vi "SOUR_POW_CORR_DATA.vi"(0 "VISA IN":refnum<visa-resource-name>, 5 "error in":errorcluster, 7 "Channel":i32) -> (14 "VISA Out":refnum<visa-resource-name>, 19 "error out":errorcluster)   [LabVIEW 2018, in "PNA-X.lvlib"]
doc: "SOURce:POWer:CORRection:DATA \nParameters \n<char> Choose from: \nREAL,32 - (default value for REAL) Best for transferring large amounts of \nmeasurement data. \nREAL,64 - Slower but has more significant digits than REAL,32. Use \nREAL,64 if you have a computer that doesn't support REAL,32. \nASCii,0 - The easiest to implement, but very slow. Use if small amounts of \ndata to transfer. \nNote: The REAL,32 and REAL,64 arguments transfer data in block format as \nexplained in Transferring Measurement Data. \nExamples FORM REAL,64 \nformat:data ascii \nQuery Syntax FORMat:DATA? \nReturn Type Character,Character \nDefault ASCii,0 \n1603\n\nHardcopy Command \nLearn about Printing \nSCPI Command Tree \nHCOPy:FILE <filename> \n(Write-only) Saves the screen image to a file. \nParameters \n<filename> Name of the file to save the screen to. The file is saved to the current working \ndirectory unless a valid full path name is specified. \nUse one of the following suffixes: \n.bmp - not recommended due to large file size \n.jpg - not recommended due to poor quality \n.png - recommended \nExamples HCOPY:FILE \"myFile.png\" \nhcopy:file \"c:\\data\\myfile.png\" \nQuery Syntax Not Applicable \nDefault Not Applicable \nHCOPy[:IMMediate] \n(Write-only) Prints the screen to the default printer. \nExamples HCOP \nhcopy:immediate \nQuery Syntax Not applicable \nDefault Not Applicable \n1604\n\nInitiate Commands \nControls triggering signals \nClick on a blue keyword to view the command details. \nSee Also \nExample Triggering the PNA \nLearn about Triggering \nSynchronizing the PNA and Controller \nSCPI Command Tree \nINITiate:CONTinuous <boolean> \n(Read-Write) Specifies whether the PNA trigger source is set to Internal (continuous) or Manual. \nThis command is a subset of TRIG:SEQ:SOURce, which can also set the trigger source to External. \nTo set how a channel responds to trigger signals, use SENS:SWE:MODE. \nSee a map of user interface to SCPI triggering commands. \nFor more information on triggering, see the PNA Trigger Model. \nSee the Example program: Triggering the PNA using SCPI. \nParameters \n<boolean> ON (or 1) - Internal (continuous) trigger. \nOFF (or 0) - Manual sweep. Use INIT:IMMediate to send a trigger signal \nExamples INIT:CONT ON \ninitiate:continuous off \nQuery Syntax INITiate:CONTinuous? \nReturn Type Boolean (1 = ON, 0 = OFF) \nDefault ON \n1605\n\nINITiate<cnum>[:IMMediate] \n(Write-only) Stops the current sweeps and immediately sends a trigger. (Same as Trigger! on the PNA \nfront panel). \nSee the Example program: Triggering the PNA using SCPI \nNote: An SMC Fixed Output measurement cannot be triggered using this command. For more \ninformation, see the example program. \nThis command requires Trigger:Source to be set to Manual. This causes ONE trigger signal to be \nSENT each time INIT:IMM is issued. \nSens<ch>:Sweep:Mode sets the number of trigger signals each channel will ACCEPT (Continuous - \nunlimited, Groups - a specific number, or HOLD - none.) \nTo trigger ALL channels in turn: \nSet ALL channels to Sens<ch>:Sweep:Mode Continuous. The <ch> argument in INIT<ch>:IMM is \nignored. \nThen�\nTRIG:SCOP ALL triggers ALL channels (in sequence) each time Init:Imm is sent. \nTRIG:SCOP CURRent triggers ONLY the NEXT channel each time Init:Imm is sent. \nTo trigger ONLY a specified channel: \nSet ALL channels to Sens<ch>:Sweep:Mode HOLD 1. \nSend TRIG:SCOP CURRent 2. \nSend Init<ch>:Imm where <ch> is the channel to be triggered. 3. \nAdvanced Situations that require some channels to be in CONT and others in HOLD are rare. The \nfollowing describes the behavior of the Init:Imm command in these situations: \nWhen Trigger:Scope = Global: \nIf the SPECIFIED <cnum> channel is in hold mode, it is put in single trigger (accepts 1 trigger signal) and \ngoes to the end of the queue of channels to be triggered. The other 'non-hold' channels are triggered. The \nnext Init:Imm triggers the specified channel first. \nFor example: ch1 is in Hold, ch2 and ch3 are in CONT and we send INIT1:IMM \n1606\n\nOn the first INIT:IMM, ch2 and ch3 is triggered. \nnext INIT:IMM, ch1, ch2, ch3 is triggered. \nnext INIT:IMM, ch2 and ch3 is triggered. \nnext INIT:IMM, ch1, ch2, ch3 is triggered, and so forth. \nWhen Trigger:Scope = Channel \nOnly ONE channel is triggered for each issued INIT<ch>:IMM command. \nIf the specified channel is in hold, it is put in single trigger (accepts 1 trigger signal) and goes the end of the \nqueue of channels to be triggered as in the 'Global' example. \nThis is one of the PNA overlapped commands. Learn more. \nParameters \n<cnum> Any existing channel number. If unspecified, value is set to 1 \nExamples INIT \ninitiate2:immediate \nQuery Syntax Not applicable \nDefault Not applicable \nLast modified: \nApril 23, 2007 Updated Init:Imm \n1607\n\nMemory Commands \nThe memory commands control saving and loading instrument states and measurement trace data to the \nhard drive. To read and write trace data in GPIB format, see CALC:DATA. \nClick on a blue keyword to view the command details. \nSee Also \nExample Programs \nLearn about Save / Recall and File Types \nSynchronizing the PNA and Controller \nSCPI Command Tree \nSpecifying Path Names \nThe MMEM commands use the following rules to specify path names: \nThe default folder is \"C:\\Program Files\\Agilent\\Network Analyzer\\Documents\" \nYou can change the active directory using MMEMory:CDIRectory. \nSpecify only the file name if using the active directory. \nYou can also use an absolute path name to specify the folder and file. \nMMEMory:CATalog[:<char>]? [<folder>] \n1608\n\n(Read-only) Returns a comma-separated string of file names that are in the specified folder. If there \nare no files of the specified type, \"NO CATALOG\" is returned. Learn about File Types \nParameters \n<char> The type of files to list. Choose from: \nSTATe - Instrument states (.sta) \nCORRection - Calibration Data (.cal) \nCSARchive - Instrument state and calibration data (.csa) \nCSTate - Instrument state and link to Calibration data (.cst) \nIf unspecified then ALL file types (even unknown types) are listed. \n<folder> String - Any existing folder name. See Specifying Path Names \nExamples MMEM:CAT? 'lists all files from the current folder \nmmemory:catalog:correction? 'C:\\Program Files\\Agilent\\Network \nAnalyzer\\Documents' 'lists .cal files from the specified folder \nDefault Not applicable \nMMEMory:CDIRectory <folder> \n(Read-Write) Changes the folder name. \nParameters \n<folder> Any drive and folder name that already exists. \nIf the same level as \"C:\\Program Files\\Agilent\\Network Analyzer\\Documents\", \nthen no punctuation is required \nMMEM:CDIR Service \nIf the new folder is at a different level than \"C:\\Program Files\\Agilent\\Network \nAnalyzer\\Documents\", use a slash (\\) before the folder name and enclose in \nquotes. \nmmemory:cdirectory '\\automation' 'changes default directory up \none level. \nYou can use an absolute path to specify the new folder. \nmmemory:cdirectory 'c:\\automation\\service' \nQuery Syntax MMEMory:CDIRectory? 'Returns the current folder name \n1609\n\nReturn Type String \nDefault 'C:\\Program Files\\Agilent\\Network Analyzer\\Documents' \nMMEMory:COPY <file1>,<file2> \n(Write-only) Copies file1 to file2. Extensions must be specified. \nParameters \n<file1> String - Name of the file to be copied. See Specifying Path Names \n<file2> String - Name of the file to be created from file1. \nExamples MMEM:COPY 'MyFile.cst','YourFile.cst' \nQuery Syntax Not applicable \nDefault Not applicable \nMMEMory:DELete <file> \n(Write-only) Deletes file. Extensions must be specified. \nParameters \n<file> String - Name of the file to be deleted. See Specifying Path Names \nExamples MMEM:DEL 'MyFile.cst' \nQuery Syntax Not applicable \nDefault Not applicable \nMMEMory:LOAD[:<char>] <file> \n1610\n\n(Write-only) Loads the specified file. Learn about File Types \nParameters \n<char> The type of file to load. Choose from: \nSTATe - Instrument states (.sta) \nCORRection - Calibration Data (.cal) \nCSARchive - Instrument state and calibration data (.csa) \nCSTate - Instrument state and link to Calibration data (.cst) \nIf <char> is unspecified, the extension must be included in the filename. \nIf an extension is specified in <file> that does not agree with <char> then no \naction is taken. \n<file> String - Name of the file to be loaded. See Specifying Path Names \nExamples MMEM:LOAD 'MyFile.cst' \nmmemory:load:state 'MyInstState' \nQuery Syntax Not applicable \nDefault Not applicable \nMMEMory:MDIRectory <folder> \n(Write-only) Makes a folder. \nParameters \n<folder> String - Name of the folder to make. See Specifying Path Names \nExamples MMEM:MDIR 'MyFolder' \nmmemory:mdirectory 'c:\\NewFolder' \nQuery Syntax Not applicable \nDefault Not applicable \nMMEMory:MOVE <file1>,<file2> \n1611\n\n(Write-only) Renames <file1> to <file2>. File extensions must be specified. \nParameters \n<file1> String - Name of the file to be renamed. See Specifying Path Names \n<file2> String - Name of the new file. \nExamples MMEM:MOVE 'MyFile.cst','YourFile.cst' \nQuery Syntax Not applicable \nDefault Not applicable \nMMEMory:RDIRectory <folder> \n(Write-only) Removes the specified folder. \nParameters \n<folder> String - Name of the folder to remove. See Specifying Path Names \nExamples MMEM:RDIR 'MyFolder' \nQuery Syntax Not applicable \nDefault Not applicable \nMMEMory:STORe[:<char>] <file> \n(Write-only) Stores the specified file (.sta, .cal, .csa, .cst, prn). \nTo save snp files, use Calc:Data:SNP:PORTs:SAVE. \nTo save *.cti files, use MMEM:STOR:CIT:DATA or MMEM:STOR:CIT:FORM. \nParameters \n<char> The type of file to store. Choose from: \nSTATe - Instrument states (.sta) \nCORRection - Calibration Data (.cal) \nCSARchive - Instrument state and calibration data (.csa) \nCSTate - Instrument state and link to Calibration data (.cst) \nNo <char> is specified for prn. \n1612\n\nIf <char> is unspecified, then the extension must be included in the filename. \nIf an extension is specified in <file> that does not agree with <char> then no \naction is taken. \nLearn about File Types \n<file> String - Name of any valid file that is not already in existence. See Specifying \nPath Names \nExamples MMEM:STOR:STAT 'myState' \nmmemory:store 'c:\\bin\\myState.sta' \nMMEM:STOR 'MyData.prn' \nQuery Syntax Not applicable \nDefault Not applicable \nMMEMory:STORe:CITifile:DATA <filename> \n(Write only) Saves UNFORMATTED trace data to .cti file. Learn more. \nParameters \n<filename> Any drive and folder name that already exists. \nIf the same level as \"C:\\Program Files\\Agilent\\Network Analyzer\\Documents\", \nthen no punctuation is required \nMMEM:STOR:CIT:DATA MYCTIFile \nIf the new folder is at a different level than \"C:\\Program Files\\Agilent\\Network \nAnalyzer\\Documents\", use a slash (\\) before the folder name and enclose in \nquotes. \nmmemory:cdirectory '\\automation' 'changes default directory up \none level. \nYou can use an absolute path to specify the new folder. \nmmemory:cdirectory 'c:\\automation\\service' \nQuery Syntax Not Applicable \nDefault C:\\Program Files\\Agilent\\Network Analyzer\\Documents' \nMMEMory:STORe:CITifile:FORMat <filename> \n1613\n\n(Write only) Saves FORMATTED trace data to .cti file. Learn more. \nParameters \n<filename> Any drive and folder name that already exists. \nIf the same level as \"C:\\Program Files\\Agilent\\Network Analyzer\\Documents\", \nthen no punctuation is required \nMMEM:STOR:CIT:DATA MYFile \nIf the new folder is at a different level than \"C:\\Program Files\\Agilent\\Network \nAnalyzer\\Documents\", use a slash (\\) before the folder name and enclose in \nquotes. \nmmemory:cdirectory '\\automation' 'changes default directory up \none level. \nYou can use an absolute path to specify the new folder. \nmmemory:cdirectory 'c:\\automation\\service' \nQuery Syntax Not Applicable \nDefault C:\\Program Files\\Agilent\\Network Analyzer\\Documents' \nMMEMory:STORe:TRACe:CONTents:CITifile <char> \n(Read-Write) Specifies the contents of subsequent citifile save statements. (See Data Define Saves) \nParameters \n<char> Choose from: \nSING - Single trace \nDISP - All displayed traces \nAUTO - All displayed traces \nExamples MMEM:STOR:TRAC:CONT:CIT SING \nQuery Syntax MMEMory:STORe:TRACe:CONTents? \nReturn Type Character \nDefault Auto \nMMEMory:STORe:TRACe:FORMat:CITifile <char> \n1614\n\n(Read-Write) Specifies the format of subsequent citifile save statements. (See Data Define Saves) \nParameters \n<char> Format in which the citifile will be saved with subsequent \nMMEMory:STORe:CIT:FORMat statements. Choose from: \nMA - Linear Magnitude / degrees \nDB - Log Magnitude / degrees \nRI - Real / Imaginary \nAUTO - Format in which the trace is already displayed. If other than Log \nMag, Linear Magnitude, or Real/Imag, then the format will be in Real/Imag. \nExamples MMEM:STOR:TRAC:FORM:CIT MA \nQuery Syntax MMEMory:STORe:TRACe:FORMat:CITifile? \nReturn Type Character \nDefault Auto' \nMMEMory:STORe:TRACe:FORMat:SNP <char> \n(Read-Write) Specifies the format of subsequent .s1p, .s2p, .s3p; s4p save statements. (See Data \nDefine Saves). \nParameters \n<char> Choose from: \nMA - Linear Magnitude / degrees \nDB - Log Magnitude / degrees \nRI - Real / Imaginary \nAUTO - data is output in currently selected trace format. If other than LogMag, \nLinMag, or Real/Imag, then output is in Real/Imag. \nExamples MMEM:STOR:TRAC:FORM:SNP MA \nQuery Syntax MMEMory:STORe:TRACe:FORMat:SNP? \nReturn Type Character \nDefault Auto' \n1615\n\nMMEMory:TRANsfer <fileName>,<dataBlock> \n(Read-Write) Transfers data between the PNA and an external controller. Other MMEM commands \ntransfer data between the PNA application and the PNA hard drive. If <fileName> already exists, it \nwill be overwritten. The file must be no larger than 20MB. \nTo read trace data from the PNA in block format, use CALC:DATA. \nParameters \n<fileName> String - File name. See Specifying Path Names \n<dataBlock> Block Data - The contents of the file. \nThe data block is a block of binary data. Use the following syntax: \n#<num digits><byte count><data bytes><NL><END> \nwhere: \n<num_digits> specifies how many digits are contained in <byte_count> \n<byte_count> specifies how many data bytes will follow in <data bytes> \nExample See example program \nQuery Syntax MMEMory:TRANsfer? <fileName> \nReads block data from the specified file location. \nDefault Not applicable \nLast modified: \n9/12/06 MQ Store command has reference to PORTS Snp. \n1616\n\nOutput Command \nLearn about Power \nOUTPut[:STATe] <ON | OFF> \n(Read-Write) Turns RF power from the source ON or OFF. \nSee note about source power state with instrument state save and recall. \nParameters \n<ON | OFF> ON (or 1) - turns RF power ON \nOFF (or 0) - turns RF power OFF \nExamples OUTP ON \noutput:state off \nQuery Syntax OUTPut[:STATe]? \nReturn Type Boolean (1 = ON, 0 = OFF) \nDefault ON \n1617\n\nRoute Command \nLearn about Frequency Offset \nSCPI Command Tree \nROUTe<cnum>:PATH:LOOP[:R1] <char> \n(Read-Write) Throws internal switch to reference receiver when the specified channel is measured. \nThis feature is only available on PNA models with Option 081 - external reference switch. See block \ndiagram of the reference switch. \nParameters \n<cnum> Any existing channel number. If unspecified, value is set to 1 \n<char> Position of the switch. Choose from: \nINTernal - bypass R1 Loop. Connects the port 1 source directly to the R1 \nreceiver. \nEXTernal - flow through R1 Loop. Allows direct access to the R1 receiver \nthrough the Reference 1 front-panel connectors. \nExamples ROUT:PATH:LOOP INT \nroute2:path:loop:r1 external \nQuery Syntax ROUTe<cnum>:PATH:LOOP:R1? \nReturn Type Character \nDefault INTernal \n1618\n\nSense:Average Commands \nSets sweep-to-sweep averaging parameters. Averaging is a noise reduction technique that averages \neach data point over a user-specified number of sweeps. Averaging affects all of the measurements in \nthe channel. \nClick on a blue keyword to view the command details. \nSee Also \nExample using some of these commands. \nLearn about Averaging \nSynchronizing the PNA and Controller \nSCPI Command Tree \nSENSe<cnum>:AVERage:CLEar \n(Write-only) Clears and restarts averaging of the measurement data. Must also set \nSENS:AVER[:STATe] ON \nParameters \n<cnum> Any existing channel number; if unspecified, value is set to 1. \nExamples SENS:AVER:CLE \nsense2:average:clear \nQuery Syntax Not applicable \nDefault Not applicable \nSENSe<cnum>:AVERage:COUNt <num> \n1619\n\n(Read-Write) Sets the number of measurement sweeps to combine for an average. Must also set \nSENS:AVER[:STATe] ON \nParameters \n<cnum> Any existing channel number; if unspecified, value is set to 1. \n<num> Number of measurement sweeps to average. Choose any number between 1 \nand 65536 (2^16). \nExamples SENS:AVER:COUN 999 \nsense2:average:count 73 \nQuery Syntax SENSe<cnum>:AVERage:COUNt? \nReturn Type Numeric \nDefault 1 \nSENSe<cnum>:AVERage[:STATe] <ON | OFF> \n(Read-Write) Turns trace averaging ON or OFF. \nParameters \n<cnum> Any existing channel number; if unspecified, value is set to 1. \n<ON | OFF> ON (or 1) - turns averaging ON. \nOFF (or 0) - turns averaging OFF. \nExamples SENS:AVER ON \nsense2:average:state off \nQuery Syntax SENSe<cnum>:AVERage[:STATe]? \nReturn Type Boolean (1 = ON, 0 = OFF) \nDefault Off \n1620\n\nSense:Bandwidth Commands \nSee Also \nExample Programs \nLearn about IF Bandwidth \nSynchronizing the PNA and Controller \nSCPI Command Tree \nSENSe<cnum>:BANDwidth | BWIDth[:RESolution] <num> \n(Read-Write) Sets the bandwidth of the digital IF filter to be used in the measurement. (Use either \nSense:Bandwidth or Sense:Bwidth) \nParameters \n<cnum> Any existing channel number. If unspecified, value is set to 1 \n<num> IF Bandwidth in Hz. The list of valid IF Bandwidths is different depending on \nthe PNA model. (Click to see the lists.) If an invalid number is specified, the \nanalyzer will round up to the closest valid number. \nExamples SENS:BWID 1KHZ \nsense2:bandwidth:resolution 1000 \nQuery Syntax SENSe<cnum>:BANDwidth | BWIDth[:RESolution]? \nReturn Type Numeric \nDefault See Preset IFBW for your PNA model. \nSENSe<cnum>:BANDwidth | BWIDth:TRACk <bool> \n1621\n\n(Read-Write) Sets and returns the state of the Reduce IF BW at Low Frequencies feature. \n(Use either Sense:Bandwidth:Track or Sense:Bwidth:Track). \nParameters \n<cnum> Any existing channel number. If unspecified, value is set to 1 \n<bool> Choose from: \nON or 1 - Reduce IF BW at Low Frequencies is set ON \nOFF or 0 - Reduce IF BW at Low Frequencies is set OFF \nExamples SENS:BWID:TRAC OFF \nsense2:bandwidth:track 1 \nQuery Syntax SENSe<cnum>:BANDwidth | BWIDth:TRACk? \nReturn Type Boolean \nDefault ON \n1622\n\nSense:Correction Commands \nPerforms and applies calibration and other error correction features. \nTo perform Guided Calibration, see Sens:Corr Coll:GUIDed. \n1623\n\nClick on a blue keyword to view the command details. \nSee Also \nExample Programs \nNew See Calibrating the PNA Using SCPI \nLearn about Measurement Calibration \nSynchronizing the PNA and Controller \nSCPI Command Tree \nSENSe<cnum>:CORRection:CCHeck[:ACQuire] <mod>[,char] \n(Write-only) Reads the 'confidence data' associated with the specified ECal module and puts it into \nmemory. The measurement is selected using SENS:CORR:CCH:PAR. This command is compatible \nwith *OPC. \nParameters \n<cnum> Any existing channel number. If unspecified, value is set to 1. \n<mod> ECAL Module that contains the confidence data. Choose from: \nECAL1 \n..through.. \nECAL8 \n[char] Optional argument. Specifies which characterization within the ECal module \nthat the confidence data will be read from. \nCHAR0 Factory characterization (data that was stored in the ECal module by \n1624\n\nAgilent). Default if not specified. \nCHAR1 User characterization #1 \nCHAR2 User characterization #2 \nCHAR3 User characterization #3 \nCHAR4 User characterization #4 \nCHAR5 User characterization #5 \nExamples SENS:CORR:CCHeck ECAL2 \nsense2:correction:ccheck:acquire ecal1,char1 \nQuery Syntax Not applicable \nDefault Not applicable \nSENSe<cnum>:CORRection:CCHeck:DONE \n(Write-only) Concludes the Confidence Check and sets the ECal module back into the idle state. \nParameters \n<cnum> Any existing channel number. If unspecified, value is set to 1 \nExamples SENS:CORR:CCH:DONE \nsense2:correction:ccheck:done \nQuery Syntax Not applicable \nDefault Not applicable \nSENSe<cnum>:CORRection:CCHeck:PARameter <Mname> \n1625\n\n(Read-Write) Specifies an existing measurement to be used for the Confidence Check. \nParameters \n<cnum> Any existing channel number. If unspecified, value is set to 1 \n<Mname> Name of the measurement you are selecting for the confidence check. The \nmeasurement must already exist. \nExamples SENS:CORR:CCH:PAR 'TEST' \n'selects the measurement \"test\" on channel 1 for the confidence \ncheck \nsense2:correction:ccheck:parameter 'test' \n'selects the measurement \"test\" on channel 2 for the confidence \ncheck \nQuery Syntax SENSe<cnum>:CORRection:CCHeck:PARameter? \nReturns the name of the selected measurement on channel <cnum>. \nReturn Type String \nDefault Not applicable \nSENSe<cnum>:CORRection:COLLect[:ACQuire] <class>[,subclass] \n(Write-only) For UNGUIDED calibration, measures the specified standards from the selected \ncalibration kit. The calibration kit is selected using the Sense:Correction:Collect:CKIT command. \nFor using two sets of standards, see SENS:CORR:TST. \nNote: Before using this command you must select two items: \n1. Select a calibration method using SENS:CORR:COLL:METH \n2. Select a measurement using CALC:PAR:SEL. You can select one measurement for each channel. \nParameters \n<cnum> Any existing channel number. If unspecified, value is set to 1 \n<class> Measures the standards associated with these class labels. Choose from: \n1626\n\nLabel Forward Reverse \nSTAN1 S11A S22A \nSTAN2 S11B S22B \nSTAN3 S11C S22C \nSTAN4 S21T S12T \nSTAN5 Generic Isolation; not associated with calibration kit definition. \nECAL1 \nthrough \nECAL8 \nECAL modules \nPOWer Take a receiver power cal sweep and turn correction ON \nSLSET Sets 'sliding load type', and increments the \"number of slides\" count. \nThe total number of slides is critical to the correct calculation of the \nsliding load algorithm. See a sliding load cal example. \nSLDONE Computes the sliding load using a circle fit algorithm. \n[subclass] Optional argument. For mechanical calibration kits, choose from the following to \nspecify the standard to be acquired from the SENS:CORR:COLL:CKIT:ORDer list. \nIf not specified, subclass is set to SST1. \nSST1 First standard in the order list \nSST2 Second standard in the order list \nSST3 Third standard in the order list \nSST4 Fourth standard in the order list \nSST5 Fifth standard in the order list \nSST6 Sixth standard in the order list \nSST7 Seventh standard in the order list \nIf an ECAL module (1 through 8) is specified for <class>, choose one of the \nfollowing for specifying which characterization within the ECal module will be \nused for the acquire. If not specified, the default is CHAR0. \nCHAR0 Factory characterization (data that was stored in the ECal module by \nAgilent) \nCHAR1 User characterization #1 \nCHAR2 User characterization #2 \nCHAR3 User characterization #3 \nCHAR4 User characterization #4 \nCHAR5 User characterization #5 \n1627\n\nExamples SENS:CORR:COLL STAN1 \n'If SENS:CORR:COLL:CKIT:ORDer2 5,3,7 \nwas specified, the following command measures standard 3 (the \nsecond in the order list) \nsense1:correction:collect:acquire stan3,sst2 \nSENS:CORR:COLL ECAL4 \nsense2:correction:collect:acquire ecal2,char1 \nQuery Syntax Not applicable \nDefault Not applicable \nSENSe<cnum>:CORRection:COLLect:APPLy \n(Write-only) Applies error terms to the measurement that is selected using Calc:Par:Select. \nNote: Before using this command you must select a measurement using CALC:PAR:SEL. You can \nselect one measurement for each channel. \nNote: This command is only necessary if you need to modify error terms. If you do not need to modify \nerror terms, SENSe<cnum>:CORRection:COLLect:SAVE calculates and then automatically applies \nerror terms after you use SENS:CORR:COLL:ACQuire to measure cal standards. \nParameters \n<cnum> Any existing channel number. If unspecified, value is set to 1 \nExample CALCulate2:PARameter:SELect S21_2 'select the measurement to \napply terms to \n1. \nSENSe2:CORRection:COLLect:METHod SPARSOLT 'set type of cal \nmethod. \n2. \nCALCulate2:DATA? SCORR1 'download the error term of interest 3. \n'Modify the error term here 4. \nCALCulate2:DATA SCORR1 'upload the error term of interest 5. \nSENSe2:CORRection:COLLect:APPLy 'applies the error terms to \nthe measurement \n6. \nQuery Syntax Not applicable \nDefault Not applicable \n1628\n\nSENSe:CORRection:COLLect:ISOLation:AVERage:INCRement <num> \n(Read-Write) Specifies amount to increment (increase) the channel averaging factor during isolation \nmeasurement of the ECal module during an unguided ECal calibration. \nNote: if the channel currently has averaging turned OFF and <num> is greater than 1, averaging will \nbe turned ON only during the isolation measurements and with the averaging factor equal to <num>. \nParameters \n<num> Incremental Averaging factor. The maximum averaging factor is 65536 (2^16). \nExamples SENS:CORR:COLL:ISOL:AVER:INCR 16 \nsense:correction:collect:isolation:average:increment 0 \nQuery Syntax SENSe:CORRection:COLLect:ISOLation:AVERage:INCRement? \nReturn Type Numeric \nDefault 8 - If this command is NOT sent, but ECal isolation is measured, then \naveraging will be turned ON with factor set to 8 during the isolation \nmeasurement. \nSENSe<cnum>:CORRection:COLLect:ISOLation:ECAL:[:STATe] <bool> \n(Read-Write) Specifies whether or not the isolation state of the ECal module will be measured as part \nof an unguided ECal calibration. \nAn unguided calibration is performed using the SENS:CORR:COLL:METH and \nSENS:CORR:COLL:ACQ commands. \nNote: The inherent isolation of the PNA is better than that attained with this command. ONLY use \nthis command when using an external test set, and ONLY using a 8509x ECal module. \nParameters \n<cnum> Any existing channel number. If unspecified, value is set to 1 \n<bool> ON (or 1) - isolation is measured during the unguided ECal calibration. \nOFF (or 0) isolation is NOT measured during the unguided ECal calibration. \nExamples SENS1:CORR:COLL:ISOL:ECAL ON \nsense2:correction:collect:isolation:ecal:state 0 \nQuery Syntax SENSe:CORRection:COLLect:ISOLation:ECAL:STATe? \nReturn Type Boolean (1 = ON, 0 = OFF) \nDefault OFF \n1629\n\nSENSe<cnum>:CORRection:COLLect:METHod <char> \n(Read-Write) For UNGUIDED calibration, sets the calibration method (also known as 'Calibration \nType' on calibration dialog box.) To select a Cal Type from a Cal Set, use CALC:CORR:TYPE. \nNote: Before using this command you must select a measurement using CALC:PAR:SEL. You can \nselect one measurement for each channel. \nParameters \n<cnum> Any existing channel number. If unspecified, value is set to 1 \n<char> Choose from: \nMethod Description \nNONE No Cal method \nREFL1OPEN Response Open \nREFL1SHORT or \nREFL1 \nResponse Short \nREFL3 Full 1 port \nRPOWer Receiver Power Cal \nTRAN1 Response Thru \nTRAN2 Response Thru and Isolation \nSPARSOLT Full SOLT 2 port \nSPARTRL TRL Cal (not available on all PNAs.) \nExamples SENS:CORR:COLL:METH REFL1 \nsense2:correction:collect:method sparsolt \nQuery Syntax SENSe<cnum>:CORRection:COLLect:METHod? \nReturn Type Character \nDefault Not Applicable \nSENSe<cnum>:CORRection:COLLect:SAVE \n1630\n\n(Write-only) For UNGUIDED calibrations ONLY. This command does the following: \ncalculates the error terms using the selected :METHod, \napplies the error terms to the selected measurement (turns error correction ON.) \nsaves the calibration error-terms to the channels Cal Register or a User Cal Set. \nThe Cal Register or User Cal Set is determined by the setting of the \nSENS:CORR:PREFerence:CSET:SAVE command. \nDo NOT use this command during an ECAL. When performing an ECAL calibration using \nSENS:CORR:COLL:ACQuire, this SAVE operation is performed automatically before the \ncompletion of a successful ACQuire. \nBefore using this command you must select a measurement using CALC:PAR:SEL. You can select \none measurement for each channel. \nParameters \n<cnum> Any existing channel number. If unspecified, value is set to 1 \nExamples SENS:CORR:COLL:SAVE \nsense2:correction:collect:save \nQuery Syntax Not applicable \nDefault Not applicable \nSENSe:CORRection:IMPedance:INPut:MAGNitude <num> \n(Read-Write) Sets and returns the system impedance value for the analyzer. \nParameters \n<num> System Impedance value in ohms. Choose any number between 0 and 1000 \nohms. \nExamples SENS:CORR:IMP:INP:MAGN 75 \nsense:correction:impedance:input:magnitude 50.5 \nQuery Syntax SENSe:CORRection:IMPedance: \nINPut:MAGNitude? \nReturn Type Numeric \nDefault 50 \n1631\n\nSENSe<cnum>:CORRection:INTerpolate[:STATe] <ON | OFF> \n(Read-Write) Turns correction interpolation ON or OFF. \nNote: Before using this command you must select a measurement using CALC:PAR:SEL. You can \nselect one measurement for each channel. \nParameters \n<cnum> Any existing channel number. If unspecified, value is set to 1 \n<ON | OFF> ON (or 1) - turns interpolation ON. \nOFF (or 0) - turns interpolation OFF. \nExamples SENS:CORR:INT ON \nsense2:correction:interpolate:state off \nQuery Syntax SENSe<cnum>:CORRection:INTerpolate[:STATe]? \nReturn Type Boolean (1 = ON, 0 = OFF) \nDefault ON \nSENSe<cnum>:CORRection:ISOLation[:STATe] <ON | OFF> OBSOLETE \nThis command no longer works beginning in the PNA 5.2 release. To perform isolation as part of an \nunguided calibration, you must explicitly measure the isolation standard using \nSENS:CORR:COLL:ACQ Stan5. See Example program. \nTo measure isolation as part of an ECal, use SENS:CORR:COLL:ISOL:ECAL. \n(Read-Write) Turns isolation cal ON or OFF during Full 2-port calibration. If this command is not \nsent, the default state is to disable Isolation. \nParameters \n<cnum> Any existing channel number. If unspecified, value is set to 1 \n<ON | OFF> ON (or 1) - turns isolation ON. \nOFF (or 0) - turns isolation OFF. \nExamples SENS:CORR:ISOL ON \nsense2:correction:isolation:state off \nQuery Syntax SENSe<cnum>:CORRection:ISOLation[:STATe]? \nReturn Type Boolean (1 = ON, 0 = OFF) \nDefault OFF - (Isolation disabled) \nSENSe:CORRection:PREFerence:CSET:SAVE <char> \n1632\n\nImportant Notes: \nThis command replaces SENS:CORR:PREF:CSET:SAVU \nWith 6.0 we implemented a change that defaults to saving completed calibrations to Cal Registers instead \nof User Cal Sets. To revert to the old behavior, send this command with the USER argument. \n(Read-Write) Specifies the default manner in which calibrations that are performed using SCPI or \nCOM are to be stored. Cal data is ALWAYS stored to the channel Cal Register regardless of this \nsetting. \nThis setting survives instrument preset and reboot. It remains until changed by another execution of \nthis command. \nNote: Cal Set arguments used with commands such as SENS:CORR:COLL:GUID:INIT, \nSENS:CORR:COLL:GUID:SAVE and SENS:CORR:COLL:GUID:SAVE:CSET will override of any \nof these default preference settings. \nLearn about Cal Registers and User Cal Sets. \nParameters \n<char> CALRegister - Cal is saved ONLY to the channel Cal Register. \nUSER - Cal is saved to a new User Cal Set file when performing a SCPI \ncalibration. The Cal Set name is automatically generated. To change the name, \nsend SENS:CORR:CSET:NAME after the cal is complete. This reverts to pre- \n6.0 behavior. \nREUSe - The cal is saved to the Cal Set that is currently selected on the \nspecified channel, which could be the channel Cal Register. If the channel does \nnot yet have a selected Cal Set, the cal will be saved to a new User Cal Set with \nan automatically-generated name. \nExamples SENS:CORR:PREF:CSET:SAVE USER \nsense:correction:preference:cset:save reuse \nQuery Syntax SENSe:CORRection:PREFerence:CSET:SAVE? \nReturn Type Character \nDefault CALRegister \nSENSe:CORRection:PREFerence:CSET:SAVUser <bool> Superseded \n1633\n\nThis command is replace with SENS:CORR:PREF:CSET:SAVE \nNOTE: With 6.0 we implemented a change that defaults to saving completed calibrations to Cal \nRegisters instead of User Cal Sets. To revert to the old behavior, send this command as ON (1). For \nUI and COM use, this can be done from the GPIB console. \n(Read-Write) Specifies whether cal data is automatically saved to a User Cal Set file after performing \na SCPI calibration. Cal data is always saved to a Cal Register regardless of this setting. \nThis setting survives instrument preset and reboot. It remains until changed by another execution of \nthis command. \nLearn about Cal Registers and User Cal Sets. \nParameters \n<bool> ON or 1 - Cal is automatically saved to a User Cal Set file when performing a \nSCPI calibration. The Cal Set name is automatically generated. To change the \nname, send SENS:CORR:CSET:NAME after the cal is complete. Reverts to \npre-6.0 behavior. \nOFF or 0 - Cal is NOT automatically saved to a User Cal Set. To save a \ncalibration to a User Cal Set, use SENS:CORR:COLL:GUID:INIT. \nExamples SENS:CORR:PREF:CSET:SAVU 1 \nsense:correction:preference:cset:savuser 0 \nQuery Syntax SENSe:CORRection:PREFerence:CSET:SAVUser? \nReturn Type Boolean (1 = ON, 0 = OFF) \nDefault OFF (0) \nSENSe:CORRection:PREFerence:ECAL:ORIentation[:STATe] <ON|OFF> \n1634\n\n(Read-Write) Specifies whether or not the PNA should perform orientation of the ECal module \nduring calibration. Orientation is a technique by which the PNA automatically determines which \nports of the module are connected to which ports of the PNA. Orientation begins to fail at very low \npower levels or if there is much attenuation in the path between the PNA and the ECal module. If \norientation is turned OFF, the SENS:CORR:PREF:ECAL:PMAP command must be used to specify \nthe port connections before performing a cal. \nNote: For 3-port or 4-port measurements, when orientation is OFF, you are not allowed to specify \nhow the ECAL module is connected. Instead, the PNA determines the orientation. Use \nSENS:CORR:COLL:GUID:DESC? to query the orientation. The PNA does not verify that you made \nthe connection properly. \nThis setting remains until the PNA is restarted or this command is sent again. \nParameters \n<bool> ECAL orientation state. Choose from: \nON or 1 - PNA performs orientation of the ECal module. \nOFF or 0 - PNA does NOT performs orientation of the ECal module. \nExamples SENS:CORR:PREF:ECAL:ORI OFF \nsense:correction:preference:ecal:orientation:state on \nQuery Syntax SENSe:CORRection:PREFerence:ECAL:ORIentation[:STATe]? \nReturn Type Boolean (1 = ON, 0 = OFF) \nDefault ON (1) \nSENSe:CORRection:PREFerence:ECAL:PMAP <module>,<string> \n(Read-Write) When ECal module orientation is turned OFF (SENS:CORR:PREF:ECAL:ORI), this \ncommand specifies the port mapping (which ports of the module are connected to which ports of the \nPNA) prior to performing ECal calibrations. \nThis setting remains until the PNA is restarted or this command is sent again. \nParameters \n<module> Specifies which ECal module this port map is being applied to. Choose from: \nECAL1 \n.through. \nECAL8 \n1635\n\n<string> Format this parameter in the following manner: \nAw,Bx,Cy,Dz \nwhere\nA, B, C, and D are literal ports on the ECAL module \nw,x,y, and z are substituted for PNA port numbers to which the ECAL module port \nis connected. \nPorts of the module which are not used are omitted from the string. \nFor example, on a 4-port ECal module with \nport A connected to PNA port 2 \nport B connected to PNA port 3 \nport C not connected \nport D connected to PNA port 1 \nthe string would be: A2,B3,D1 \nIf either the receive port or source port (or load port for 2-port cal) of the \nCALC:PAR:SELected measurement is not in this string and orientation is OFF, \nan attempt to perform an ECal calibration will fail. \nExamples SENS:CORR:PREF:ECAL:PMAP ECAL2, 'A1,B2' \nsense:correction:preference:ecal:pmap ecal3, 'a2,b1,c3' \nQuery Syntax SENSe:CORRection:PREFerence:ECAL:PMAP? <module> \nReturn Type String \nDefault Null string () \nSENSe:CORRection:PREFerence:SIMCal <bool> \n1636\n\n(Read-Write) Sets and returns a preference for the Unguided Cal behavior described below. This \nsetting persists until it is changed. \nThis preference can also be set True by executing the script on the PNA at C:/Program \nFiles/Agilent/Network Analyzer/System/wincal32.reg. \nParameters \n<bool> Boolean - Choose from: \n0 - False - Reverts to new (preferred) behavior. An error is returned if standard \ndata is not acquired before sending SENS:CORR:COLL:SAVE. \n1 - True - (WinCal compatible) Prevents SENS:CORR:COLL:SAVE from \nfailing when standard data has not, and will not, be acquired. \nLearn more about old and new behaviors. \nExamples SENS:CORR:PREF:SIMC 0 \nsense:correction:preference:simcal 1 \nQuery Syntax SENSe:CORRection:PREFerence:SIMCal? \nReturn Type Boolean \nDefault 0 \nSENSe:CORRection:PREFerence:TRIG:FREE <char>, <bool> \n(Read-Write) Sets and returns the preference for the trigger behavior during a calibration. This setting \npersists until it is changed. \nNote: If TRIGger:SOURce = Manual, during a calibration the PNA ALWAYS switches to Internal for \none trigger, then back to Manual, regardless of this preference command. \nParameters \n<char> Character - Calibration type. Choose from: \nGUIDed - preference setting pertains to a Guided calibration. \nUNGuided - preference setting pertains to an Unguided calibration. \n<bool> Boolean - Choose from: \n0 - False - The trigger behavior during the specified calibration type DOES \nrespect the setting of the TRIGger:SOURce command. For example,when \nTrigger source = External, the single trigger method will wait for the External \n1637\n\ntrigger signal and then allow only one sweep. \n1 - True - (Pre-6.0 behavior) The trigger behavior during the specified \ncalibration type does NOT respect the setting of the TRIGger:SOURce \ncommand. For example, when Trigger source = External, during calibration the \nPNA switches to Internal sweep, responds to one trigger signal to measure the \nstandard, then switches back to External. \nExamples SENS:CORR:PREF:TRIG:FREE GUID,1 \nsense:correction:preference:trig:free unguided,0 \nQuery Syntax SENSe:CORRection:PREFerence:TRIG:FREE? <char> \nReturn Type Boolean \nDefault False for both calibration types. \nSENSe<cnum>:CORRection:RPOWer:OFFSet[:AMPLitude] <num> \n(Read-Write) Adjusts a receiver power cal to account for components or adapters that are added \nbetween the source port and receiver while performing this cal. For more information, see Receiver \nCal. \nParameters \n<cnum> Any existing channel number. If unspecified, value is set to 1 \n<num> Offset Value in dB. Specify loss as a negative number; and gain as a positive \nnumber. Choose a number between -200 and 200. \nExamples SENS:CORR:RPOW:OFFS .5 \nsense2:correction:rpower:offset:amplitude .-5 \nQuery Syntax SENSe<cnum>:CORRection:RPOWer:OFFSet[:AMPLitude]? \nReturn Type Numeric \nDefault 0 \nSENSe<cnum>:CORRection:RVELocity:COAX <num> \n1638\n\n(Read-Write) Sets the velocity factor to be used with Electrical Delay and Port Extensions. \nParameters \n<cnum> Any existing channel number. If unspecified, value is set to 1 \n<num> Velocity factor. Choose a number between 0 and 10 \n(.66 polyethylene dielectric; .7 teflon dielectric) \nExamples SENS:CORR:RVEL:COAX .66 \nsense2:correction:rvelocity:coax .70 \nQuery Syntax SENSe<cnum>:CORRection:RVELocity:COAX? \nReturn Type Numeric \nDefault 1 \nSENSe:CORRection:SFORward[:STATe] <boolean> \n(Read-Write) Sets the direction a calibration will be performed when only one set of standards is used. \nUse SENSe:CORRection:TSTandards[:STATe] OFF to specify that only one set of standards will be \nused. \nParameters \n<boolean> ON (1) - FORWARD direction of a 2-port calibration will be performed \nOFF (0) - REVERSE direction of a 2-port calibration will be performed \nExamples SENS:CORR:SFOR 1 \nsense:correction:sforward:state 0 \nSee an example using this command \nQuery Syntax SENSe:CORRection:SFORward[:STATe]? \nReturn Type Boolean \nDefault ON \nSENSe<cnum>:CORRection[:STATe] <ON | OFF> \n1639\n\n(Read-Write) Turns error correction ON and OFF for the specified channel. \nNote: Before using this command you must select a measurement using CALC:PAR:SEL. You can \nselect one measurement for each channel. \nParameters \n<cnum> Any existing channel number. If unspecified, value is set to 1 \n<ON | OFF> ON (or 1) - correction is applied to the channel. \nOFF (or 0) - correction is NOT applied to the channel. \nExamples SENS:CORR ON \nsense2:correction:state off \nQuery Syntax SENSe<cnum>:CORRection[:STATe]? \nTo query the error correction state for a measurement, use CALC:CORR:STATe? \nReturn Type Boolean (1 = ON, 0 = OFF) \nDefault OFF \nSENSe:CORRection:TSTandards[:STATe] <boolean> \n(Read-Write) Specifies the acquisition of calibration data using ONE or TWO sets of standards. \nParameters \n<boolean> ON (1) - TWO identical sets of standards will be used to simultaneously \ncalibrate two ports (for both Forward and Reverse parameters). \nOFF (0)- ONE set of standards will be used to perform a full 2-port calibration, \none port at a time. \nWhen specifying ON (use two sets), the SENS:CORR:COLL:ACQuire \ncommand uses the same standard index for each calibration class. To specify \nthe calibration standard gender for each port, you must first ensure that the \norder of calibration class accurately reflects the configuration of your DUT. \nFor example, for a DUT with a male connector on port 1 and a female \nconnector on port 2, order the devices within the S11 classes (A, B, and C) \nsuch that the MALE standards are first in the list. Then order the S22 classes \nspecifying the FEMALE standards as the first in the list. \nExamples SENS:CORR:TST 1 \nsense:correction:tstandard:state 0 \nSee an example using this command \n1640\n\nQuery Syntax SENSe:CORRection:TSTandards[:STATe]? \nReturn Type Boolean \nDefault ON \nSENSe:CORRection:TYPE:CATalog? <char> \n(Read-Write) Lists the Cal Types in the PNA by either GUID or registered name. Learn more about \napplying Cal Type using SCPI. \nNote: Before using this command you must select a measurement using CALC:PAR:SEL. You can \nselect one measurement for each channel. \nParameters \n<char> Specifies the type of list. Choose from: \nGUID - the registered GUID of the Cal Type \nNAME - the registered name of the Cal Type \nExamples SENS:CORR:TYPE:CAT? GUID \nQuery Syntax SENSe<cnum>:CORRection:TYPE:CATalog? <char> \nReturn Type Comma-separated string \nDefault Not Applicable \nLast modified: \nApril 14, \n2007 \nAddd ECal isolation commands \nOct 30, \n2006 \nModified SavUser command \n1641\n\nSense:Correction:Collect:Guided Commands \nPerforms and applies a SmartCal (Guided) calibration and other error correction features. \nClick on a blue keyword to view the command details. \nSee Also \nExamples using these commands. \n1642\n\nNew Calibrating the PNA Using SCPI \nLearn about Measurement Calibration \nSynchronizing the PNA and Controller \nSENSe:CORRection:COLLect:GUIDed:ACQuire <std> \n(Write-only) Initiates the measurement of the specified calibration standard. Executing this command \nwith an unnecessary standard has no affect. \nThe measured data is stored and used for subsequent calculations of error correction coefficients. All \nstandards must be measured before a calibration can be completed. Any measurement can be repeated \nuntil the SENS:CORR:COLL:GUID:SAVE command is executed. \nQuery the user prompt description using SENS:CORR:COLL:GUID:DESC? \nQuery the required calibration steps using SENS:CORR:COLL:GUID:STEP? \nParameters \n<cnum> Any existing channel number. If unspecified, value is set to 1 \n<std> Choose from:STAN1, STAN2, STAN3, through STAN40 \nExamples SENS:CORR:COLL:GUID:ACQ STAN1 \nsense:correction:collect:guided:acquire stan1 \nQuery Syntax Not Applicable \nDefault Not Applicable \nSENSe<cnum>:CORRection:COLLect:GUIDed:ADAPter:CREate? <conn1>, <conn2> \n(Read-only) Specifies the use of a THRU adapter to be used during the Guided Cal Unknown THRU \nand Adapter Removal Cal. Returns an adapter index <n> which is used to refer to the adapter in \nseveral related commands. See Cal Thru Methods. While the choice of which end of the adapter is \n<conn1> and <conn2> is arbitrary, it is necessary to remember which will be used on each test port. \nParameters \n<cnum> Any existing channel number. If unspecified, value is set to 1 \n<conn1> Adapter port 1 connector type. Use SENS:CORR:COLL:GUID:CONN:CAT? \nto return a list of valid connector types. \n<conn2> Adapter port 2 connector type. \nExamples See example using this command. \nReturn Type Numeric \n1643\n\nDefault Not Applicable \nSENSe<cnum>:CORRection:COLLect:GUIDed:ADAPter:COUNt? \n(Read-Only) Returns the number of THRU adapters that have been created for this calibration using \nSENS:CORR:COLL:GUID:ADAP:CREate? \nParameters \n<cnum> Any existing channel number. If unspecified, value is set to 1 \nExamples See example using this command. \nReturn Type Numeric \nDefault Not Applicable \nSENSe<cnum>:CORRection:COLLect:GUIDed:ADAPter<n>:DELay <coax>, [w phase, \nwdelay] \n(Write-only) Specifies the adapter delay. and optionally waveguide delay and optional phase offset \n(degrees) of adapter <n>. \nParameters \n<cnum> Any existing channel number. If unspecified, value is set to 1 \n<n> Adapter index number that was returned from \nSENS:CORR:COLL:GUID:ADAP:CREate? \n<coax> Delay value of coax adapter <n> in seconds. If the adapter has no coax \nconnector, enter 0. \n<wphase> Waveguide phase offset in degrees. If the adapter has no waveguide connector, \ndo not enter a value. \n<wdelay> Waveguide delay in seconds. If the adapter has no waveguide connector, do not \nenter a value. \nExamples See example using this command. \nDefault Not Applicable \nSENSe<cnum>:CORRection:COLLect:GUIDed:ADAPter<n>:DESCription <string> \n1644\n\n(Write-only) Specifies the adapter description for use as the guided cal connection prompts. \nParameters \n<cnum> Any existing channel number. If unspecified, value is set to 1 \n<n> Adapter index number that was returned from \nSENS:CORR:COLL:GUID:ADAP:CREate? \n<string> Adapter description. \nExamples See example using this command. \nQuery Syntax Not Applicable \nDefault Not Applicable \nSENSe<cnum>:CORRection:COLLect:GUIDed:ADAPter<n>PATHs <port pairs> \n(Write-only) Specifies the port pairs for which the adapter will be used for a THRU connection. \nFor example, for a 3-port cal on channel 1 using ports 1,2,and 3), to use adapter 1 between the ports (1 \nto 2) and (1 to 3) the following command is used: SENS1:CORR:COLL:GUID:ADAP1:PATH \n1,2,1,3. \nThe adapter must have the same DUT connectors as the ports that are already specified for these ports. \nParameters \n<cnum> Any existing channel number. If unspecified, value is set to 1 \n<n> Adapter index number that was returned from \nSENS:CORR:COLL:GUID:ADAP:CREate? \n<port pair> Ports for which the adapter will be used. The orientation is not critical, as the \nPNA will align the connector types as necessary. The minimum number of \nThru connections required is the number of ports to calibrated -1. \nExamples See example using this command. \nQuery Syntax Not Applicable \nDefault Not Applicable \nSENSe:CORRection:COLLect:GUIDed:CKIT:PORT<pnum>:CATalog? \n1645\n\n(Read-only) Returns a comma-separated list of valid kits for each port. In addition to mechanical \ncalibration kits, this will include applicable characterizations found within ECal modules currently \nconnected to the PNA. \nIf two or more identical ECal modules are connected to the PNA, the returned list will include the \nserial numbers to distinguish the ECal modules. \nUse items in the list to select the kit to be used with the SENS:CORR:COLL:GUID:CKIT:PORT \ncommand. \nParameters \n<pnum> Any existing port number. If unspecified, value is set to 1 \nExamples SENS:CORR:COLL:GUID:CKIT:PORT1:CAT? \n'When \"Type N (50) male\" is specified for connector type, \nreturns: \n\"85054D, 85032F\" \n'When two identical ECal modules are connected for the connector \ntype, \n'the return string includes serial numbers \n\"85092-60010 ECal 10675, 85092-60010 ECal 00758\" \nReturn Type String \nDefault Not Applicable \nSENSe:CORRection:COLLect:GUIDed:CKIT:PORT<pnum>[:SELect] <kit> \n(Read-Write) Specifies the calibration kit for each port to be used during a guided calibration. An \nunused port does NOT need to have a specified Cal Kit. \nIf two or more identical ECal modules are connected to the PNA, the serial number must be included \nin the <kit> string to distinguish the ECal modules. See \nSENS:CORR:COLL:GUID:CKIT:PORT:CAT? \nNote: Sliding loads are not fully supported from Sens:Corr:Coll:Guided... The Measure button must \nbe manually pressed. \n1. Specify the connector type for the port with SENS:CORR:COLL:GUID:CONN:PORT. \n2. Query the valid available kits for the connector on each port with \nSENS:CORR:COLL:GUID:CKIT:PORT:CAT? \n1646\n\n3. Specify the kit using this command. \n4. Perform a query of this command. If the <kit> parameter was incorrectly entered, an error will be \nreturned.\nParameters \n<pnum> Any existing port number. If unspecified, value is set to 1 \n<kit> Calibration kit to be used for the specified port. \nExamples SENS:CORR:COLL:GUID:CKIT:PORT1 '85055A' \n'The following includes a serial number when two or more ECal \nmods are connected \nsense:correction:collect:guided:ckit:port2:select '85092-60010 \nECal 10685' \nQuery Syntax SENSe:CORRection:COLLect:GUIDed:CKIT:PORT<pnum>[:SELect]? \nReturn Type String - If the <kit> parameter was incorrectly entered while writing, an error \nwill be returned. \nDefault Not Applicable \nSENSe:CORRection:COLLect:GUIDed:CONNector:CATalog? \n(Read only) Returns a list of valid connectors based on the connector descriptions of the available cal \nkits. Use an item from the returned list to specify a connector for \nSENS:CORR:COLL:GUID:CONN:PORT \nExamples SENS:CORR:COLL:GUID:CONN:CAT? \nReturns: \nType N (50) female, Type N (50) male, APC 7 (50), 3.5 mm (50) \nmale, 3.5 mm (50) female, User Connector A \nReturn Type Comma separated string values \nDefault Not Applicable \nSENSe:CORRection:COLLect:GUIDed:CONNector:PORT<pnum>[:SELect] <conn> \n1647\n\n(Read-Write) Specifies a connector type for every port during the Guided Calibration procedure. Valid \nconnector names are stored within calibration kits. Some cal kits may include both male and female \nconnectors. Therefore, specifying connector gender may be required. \nThe PNA remembers previous Guided Cal settings. Therefore, for completeness, unused ports should \nbe defined as \"Not used\". See Guided Cal examples. \nA single port with a valid <conn> name indicates a 1-Port calibration will be performed. \nTwo ports with valid <conn> names indicate either a 2-Port SOLT or TRL calibration will be performed \ndepending on the standards definition found within the cal kit and the capability of the PNA. \nThree ports with valid <conn> names indicate a 3-Port calibration will be performed, and so forth. \nThe following steps could be followed to ensure port connectors are specified correctly: \nUse SENS:CORR:COLL:GUID:CONN:CAT? to query available connectors before specifying the port \nconnector. \n1. \nSelect a connector type using this command. 2. \nPerform a query of this command. If the <conn> parameter was incorrectly entered, an error will be \nreturned. \n3. \nSpecify the cal kit to use for each port with SENS:CORR:COLL:GUID:CKIT:PORT 4. \nParameters \n<pnum> Any existing port number. If unspecified, value is set to 1 \n<conn> String - DUT connector type to connect with PNA port <pnum> \nExamples 'Specifying a 2-port cal (1 & 2) on a 4-port PNA \nSENS:CORR:COLL:GUID:CONN:PORT1 'Type N (50) female' \nSENS:CORR:COLL:GUID:CONN:PORT2 'Type N (50) male' \nSENS:CORR:COLL:GUID:CONN:PORT3 'Not Used' \nSENS:CORR:COLL:GUID:CONN:PORT4 'Not Used' \nQuery Syntax SENSe:CORRection:COLLect:GUIDed:CONNector:PORT<pnum>[:SELect]? \nReturn Type String \nDefault Not Applicable \nSENSe:CORRection:COLLect:GUIDed:DESCription? <step> \n1648\n\n(Read-only) Returns the connection description for the specified calibration step. \nParameters \n<step> A number from 1 to the number of steps required to complete the calibration \n(Use SENS:CORR:COLL:GUID:STEP? to query the number of steps ) \nExamples SENS:CORR:COLL:GUID:DESC? 10 \n'Returns: \nConnect APC 7 Open to port3 \nReturn Type String \nDefault Not Applicable \nSENSe:CORRection:COLLect:GUIDed:DMATch:APPLy[:IMMediate] [<CalSetGUID>] \n(Write-only) Specifies a Cal Set as a source of delta match correction. \nIf CalSetGUID is not specified, then the Global Delta Match Cal Set is assumed. An error is returned \nif the specified Cal Set does not meet the following Delta Match criteria. The Global Delta Match Cal \ncan ALWAYS be applied. \nMust have been performed using ECal or as a guided mechanical cal (not Unguided). \nMust have the same start freq, stop freq, and number of points as the channel being calibrated. \nMust calibrate the ports that are required by the TRL or Unknown Thru cal as indicated by \nSENS:CORR:COLL:GUID:DMATch:APPLy:PORTs?. \nLearn more about Delta match calibration. \nSee example of a complete Delta Match calibration. \nParameters \n<CalSetGUID> Optional. GUID of the Cal Set to use. If unspecified, the Global Delta Match \nCal Set is used. \nExamples SENS:CORR:COLL:GUID:DMAT:APPL \nsense:correction:collect:guided:dmatch:apply:immediate \n\"{2B893E7A-971A-11d5-8D6C-00108334AE96}\" \nQuery Syntax Not Applicable \nDefault Not Applicable \nSENSe:CORRection:COLLect:GUIDed:DMATch:APPLy:PORTs? \n1649\n\n(Read-only) Returns the port numbers for which delta match correction is required. 0 (zero) is \nreturned if the Cal does NOT require Delta Match correction for one of the following reasons: \nThe Cal does NOT involve Unknown THRU or TRL. You specify this using \nSENS:CORR:COLL:GUID:METH <UNKN | TRL>. \nThe Cal DOES involve Unknown THRU or TRL, but the delta match data can be calculated by the Unknown \nThru or TRL Cal. Learn how this is possible. However, you can force the Cal to use the Delta Match data \nfrom a Cal Set. \nLearn more about Delta match calibration. \nSee example of a complete Delta Match calibration. \nParameters \nExamples SENS:CORR:COLL:GUID:APPL:PORT? \n'Returns: \n1,2,3 \nReturn Type Numeric \nDefault Not Applicable \nSENSe:CORRection:COLLect:GUIDed:DMATch[:INITiate] <conn>,<cKit> \n(Write-only) Initiates a global delta match calibration. \nLearn more about Global Delta Match calibration. \nSee example of a complete Delta Match calibration. \nParameters \n<conn> String. Connector type for port 1. All other ports are set automatically. \n<cKit> String Cal Kit for all ports. If incorrectly entered while writing, an error is \nreturned. \nExamples SENS:CORR:COLL:GUID:DMAT APC 3.5 female,\"85052B\" \nQuery Syntax Not Applicable \nDefault Not Applicable \nSENSe:CORRection:COLLect:GUIDed:ETERms:LOAD[:CSET] <cset>,<calPort> [,csPort] \n1650\n\n(Write-only) Loads 1-port error terms from a Cal Set into the current Guided Cal sequence. When the \nCal steps are recomputed, connection steps are removed due to the loading of the error terms. \nSee example of how to use this command. \nParameters \n<cset> String Name of User Cal Set in which the error terms reside. \n<pnum> Integer Port number of the current cal to receive error terms. \n[csPort] Integer Optional argument. Port number associated with the error terms in the \nCal Set. If unspecified, the same port number as <calPort> is used. \nExamples See example \nQuery Syntax Not Applicable \nDefault Not Applicable \nSENSe<cnum>:CORRection:COLLect:GUIDed:INITiate [cal set name or GUID [,bool]] \n(Write-only) Initiates a guided calibration. \nThe PNA determines the measurements needed to perform the calibration using the settings specified from \nthe SENS:CORR:COLL:GUID:CONN:PORT and SENS:CORR:COLL:GUID:CKIT:PORT commands. \nAfter this command is executed, subsequent commands can be used to query the number of measurement \nsteps, issue the acquisition commands, query the connection description strings, and subsequently \ncomplete a guided calibration. \nParameters \n<cnum> Any existing channel number. If unspecified, value is set to 1 \n<cal set name or \nGUID> \n(String) Optional argument. If NOT specified, behavior depends on the \nSENS:CORR:PREFerence:CSET:SAVE setting. \nIf specified, choose an existing Cal Set, either by name or by GUID. \nCal Set name including quotes \nCalset GUID in the form: \"{GUID}\"; including quotes and curly brackets. \nQuery all Cal Set GUIDs with SENS:CORR:CSET:CAT? \nSENS:CORR:COLL:GUID:SAVE:CSET can be used instead of this optional \nargument to specify the GUID for a Cal Set. \nAn error is reported if the Cal Set is not found. \n1651\n\nThe Cal Set is either supplemented or overwritten depending on the method, \nconnectors, and ports selected. Learn more about Cal Sets. \n<bool> Optional argument. \nFalse (0) If Cal Set stimulus settings differ from the existing channel, do not \nchange channel stimulus settings. The Cal Set is save to the current setting of \nthe SENS:CORR:PREF:CSET:SAVE command. This is the default setting if \nnot specified. \nTrue (1) If cal set stimulus settings differ from the existing channel, change \nthe channel stimulus settings to match the Cal Set settings. \nExamples SENS:CORR:COLL:GUID:INIT \"{2B893E7A-971A-11d5-8D6C- \n00108334AE96}\",1 \nsense2:correction:collect:guided:initiate 'myCalSet' \nQuery Syntax Not Applicable \nDefault Not Applicable \nSENSe:CORRection:COLLect:GUIDed:ISOLation:AVERage:INCRement <num> \n(Read-Write) Specifies amount to increment (increase) the channel�s averaging factor during \nmeasurement of isolation standards in a guided calibration. \nNote: If the channel has averaging turned OFF and the value of <num> is greater than 1, averaging \nwill be turned ON only during the isolation measurements and with the averaging factor equal to \n<num>.\nParameters \n<num> Amount to increment the averaging factor for the isolation measurement. The \nmaximum averaging factor for the channel is 65536 (2^16). \nExamples 'Measure isolation on all paths for the cal \nSENS:CORR:COLL:GUID:ISOL ALL \n'Remove the port pairs 1-to-2 and 1-to-3 from the list of paths \non which to measure isolation \nsense:correction:collect:guided:isolation:paths REMove,1,2,1,3 \nQuery Syntax SENSe:CORRection:COLLect:GUIDed:ISOLation:PATHs? \nNote: if isolation is not measured, the query returns 0. \nReturn Type Numeric \n1652\n\nDefault 8 - If this command is NOT sent, but isolation is measured, then averaging will \nbe turned ON with factor set to 8 during the isolation measurements. \nSENSe:CORRection:COLLect:GUIDed:ISOLation[:PATHs] <char>[,<p1a, p1b, p2a, p2b,�>] \n(Read-Write) Specifies the paths (port pairs) to make isolation measurements on during a guided \ncalibration. \nParameters \n<char> ALL � Measure isolation on all pairings of the ports that are to be calibrated. \nNONE � Do not measure isolation on any pairing of the ports to be calibrated. \n(Default behavior). \nADD � Add one or more specific pairings of ports to the list of port pairings \nfor which isolation will be measured. \nREMove � Remove one or more specific pairings of ports from the list of port \npairings for which isolation will be measured. If many paths are to be \nmeasured, it may be easier to first send ALL, then REMove and specify the \npaths to remove. \n<p1a, p2a...> For use when <char> is ADD or REMove. \nSpecify Port numbers in pairs: \nFor 3-port cals, specify up to 3 pairs. \nFor 4-port cals, specify up to 6 pairs. \np1a, p1b (Path1 - port A and port B) \np2a, p2b (Path2 - port A and port B) \np3a, p3b (Path3 - port A and port B) \nExamples 'Measure isolation on all paths for the cal \nSENS:CORR:COLL:GUID:ISOL ALL \n'Remove the port pairs 1-to-2 and 1-to-3 from the list of paths \non which to measure isolation \nsense:correction:collect:guided:isolation:paths REMove,1,2,1,3 \n1653\n\nQuery Syntax SENSe:CORRection:COLLect:GUIDed:ISOLation:PATHs? \nNote: if isolation is not be measured on any of the paths, the query returns 0 \nReturn Type Numeric \nDefault 0 - Isolation not measured on any paths. \nSENSe:CORRection:COLLect:GUIDed:METHod <char> Superseded \nThis command is replaced with SENS:CORR:COLL:GUID:PATH:CMEThod and \nSENS:CORR:COLL:GUID:PATH:TMEThod. \n(Read-Write) Selects from one of several algorithms available for performing the THRU portion of a \nguided calibration. Learn more about THRU methods. \nParameters \n<char> DEFAULT - Informs guided calibrations to use the default algorithm when \ncomputing the number of needed standards acquisition steps. (default selection \nif omitted.) \nADAP - Use the adapter removal algorithm \nFLUSH - Use with insertable devices. \nUNKN - Use the Unknown THRU algorithm with calibrations for noninsertable \ndevices. \nDEFined - Use the THRU definition that you stored in the cal kit file, or ECal \nmodule. \nTRL - Select TRL Cal Type for guided cals. Valid for \"TRL ready\" Cal Kits \nwith properly assigned TRL cal classes. \nSOLT - Select SOLT Cal Type for guided cals. Valid for any kit with \nproperly assigned SOLT cal classes. \nExamples SENS:CORR:COLL:GUID:METH ADAP \nsense:correction:collect:guided:method unkn \nQuery Syntax SENSe:CORRection:COLLect:GUIDed:METHod? \nReturn Type Character \nDefault DEFAULT \n1654\n\nSENSe:CORRection:COLLect:GUIDed:PATH:CMEThod \n<port1>,<port2>,<caltype1[,caltype2]> \nNote: This command replaces SENS:CORR:COLL:GUID:METH. \n(Read-Write) Specifies the calibration method for each port pair. \nNote: Before using this command, first do the following: \nSet the connector types: SENS:CORR:COLL:GUID:CONN:PORTn \nSet cal kit: SENS:CORR:COLL:GUID:CKIT:PORT \nSet or query the thru path pairs: SENS:CORR:COLL:GUID:THRU:PORT \nAfter sending or querying this command, send the Thru method: \nSENS:CORR:COLL:GUID:PATH:TMEThod \nParameters \n<port1> First port of the pair to be calibrated. \n<port2> Second port of the pair to be calibrated. \n<caltype1[caltype2]> (String) Cal types for 1st and 2nd ports of the pair, enclosed in a single pair of \nquotes. NOT case-sensitive. \ncaltype1 Cal type for the pair if caltype2 is not specified. Otherwise, Cal type \nfor port 1. Choose from: \n�TRL� \n�SOLT� \n�QSOLTN� \n�EnhRespN \nFor the last two arguments, replace N with the port to be used as the source \nport, which MUST be one of the port pair. \ncaltype2 Optional argument. Use only when performing an adapter removal \ncal on the pair. This argument specifies the Cal type on the second port. \nCaltype1 then specifies the Cal type of the first port. \nChoose from the same arguments as caltype1. \nExamples SENS:CORR:COLL:GUID:PATH:CMEThod 2,3,\"QSOLT2\" \nsense:correction:collect:guided:path:cmethod 2,3,\"solt,trl\" \n1655\n\nQuery Syntax SENSe:CORRection:COLLect:GUIDed:PATH:CMEThod? <port1>,<port2> \nIf only one caltype is returned then it�s NOT adapter removal. \nReturn Type String \nDefault Not Applicable \nSENSe:CORRection:COLLect:GUIDed:PATH:TMEThod \n<port1>,<port2>,<thruType1[,thruType2]> \nNote: This command replaces SENS:CORR:COLL:GUID:METH. \n(Read-Write) Specifies the calibration THRU method for each port pair. \nNote: Before using this command, first do the following: \nSet the connector types: SENS:CORR:COLL:GUID:CONN:PORTn \nSet cal kit: SENS:CORR:COLL:GUID:CKIT:PORT \nSet or query the thru path pairs: SENS:CORR:COLL:GUID:THRU:PORT \nSet or query the Cal Type: SENS:CORR:COLL:GUID:PATH:CMEThod \nLearn more about thru methods. \nParameters \n<port1> First port of the port pair to be calibrated. \n<port2> Second port of the port pair to be calibrated. \n<thruType1[,thruType2]> (String) Thru methods for 1st and 2nd ports of the pair, enclosed in a \nsingle pair of quotes. NOT case-sensitive. \nthruType1 Calibration thru method for the pair if thruType2 is not \nspecified. Otherwise, thru method for port 1. \nChoose from: \n�Defined Thru� A thru type for which there is a stored definition in the Cal \nKit. \n�Zero Thru� Zero length thru, also known as flush-thru. \n�Undefined Thru� A thru type for which there is NOT a stored definition in \nthe Cal Kit. Also known as Unknown Thru. Valid ONLY for SOLT cal type. \n1656\n\n�Undefined Thru using a Defined Thru� Using an ECal module, measure \nthe internal thru using the \"Undefined Thru\" method. \nthruType2 Optional argument. Use only when performing an adapter \nremoval cal on the pair as determined by \nSENS:CORR:COLL:GUID:PATH:CMEThod. The only valid arguments \nfor ThruType1&2 is \"Defined Thru, Defined Thru\". \nExamples SENS:CORR:COLL:GUID:PATH:TMEThod 2,3,�Zero Thru� \nsense:correction:collect:guided:path:tmethod 2,3,\"Defined \nThru,Defined Thru\" \nQuery Syntax SENSe:CORRection:COLLect:GUIDed:PATH:TMEThod \n<port1>,<port2>? \nAlways returns two parts: \nIf the second part of the string is empty, adapter removal is NOT being \nperformed. \nIf the string is \"Defined Thru, Defined Thru\", adapter removal IS being \nperformed. \nReturn Type String \nDefault Not Applicable \nSENSe:CORRection:COLLect:GUIDed:SAVE [bool] \n(Write-only) Completes the guided cal by computing the error correction terms, turning Correction \nON, and saving the calibration to a Cal Set. \nIf all of the required standards have not been measured, the calibration will not complete properly. \nParameters \n[bool] Optional argument. If unspecified, the default behavior is the current PNA \npreference setting of SENSe:CORRection:PREFerence:CSET:SAVE \nFalse (0) Save cal data ONLY to a Cal Register. \nTrue (1) Save cal data to a Cal Register and a User Cal Set. The filename is \nautomatically generated. \nExamples SENS:CORR:COLL:GUID:SAVE \nsense2:correction:collect:guided:save 0 \nQuery Syntax Not Applicable \nDefault Not Applicable \n1657\n\nSENSe:CORRection:COLLect:GUIDed:SAVE:CSET <cal set name or guid> \n(Write-only) Completes the guided cal by computing the error correction terms, turning Correction \nON, and saving the calibration to the specified Cal Set. This command performs the same function as \nSENSe:CORRection:COLLect:GUIDed:SAVE, but this command allows the name or GUID of the \nCal Set to be specified. \nUse this command instead of the optional name or GUID argument in SENS:CORR:COLL:GUID:INIT. \nUse SENS:CORRection:CSET commands to get names or GUIDs of existing Cal Sets. \nThe cal data is also saved to the channel Cal Register. \nIf all of the required standards have not been measured, the calibration will not complete properly. \nParameters \n<cal set name or \nguid> \nString - Name or GUID of an existing Cal Set to be overwritten. If specifying a \nGUID, curly brackets must be included. \nExamples SENS:CORR:COLL:GUID:SAVE:CSET \"{2B893E7A-971A-11d5-8D6C- \n00108334AE96}\" \nsense:correction:collect:guided:save:cset \"MyCalSet\" \nQuery Syntax Not Applicable \nDefault Not Applicable \nSENSe:CORRection:COLLect:GUIDed:STEPs? \n(Read-only) Returns the number of measurement steps required to complete the current guided \ncalibration. This command is sent after the SENS:CORR:COLL:GUID:INIT, \nSENS:CORR:COLL:GUID:CONN:PORT and SENS:CORR:COLL:GUID:CKIT:PORT commands. \nExamples SENS:CORR:COLL:GUID:STEP? \nsense2:correction:collect:guided:steps? \nReturn Type Numeric \nDefault Not Applicable \nSENSe:CORRection:COLLect:GUIDed:THRU:PORTs <t1a, t1b, t2a, t2b, t3a, t3b...> \n1658\n\n(Read-Write) For calibrating more than 2-ports ONLY. Specifies the port pairs for the thru \nconnections of the calibration. \nUse the query to learn the port pairs that the PNA suggests. \nUse the set command to override these thru pairs. \nParameters \n<t1a,...> Specify Port numbers in pairs: \nFor 3-port cals, specify two or three pairs. \nFor 4-port cals, specify from three up to six pairs. \nt1a, t1b (Thru1 - port A and port B) \nt2a, t2b (Thru2 - port A and port B) \nt3a, t3b (Thru3 - port A and port B) \n...and so forth up to six pairs. \nExamples SENS:CORR:COLL:GUID:THRU:PORT 1,2,1,3,1,4 '4-port measurement \nsense:correction:collect:guided:thru:ports 1,2,2,3 '3-port \nmeasurement \nQuery Syntax SENSe:CORRection:COLLect:GUIDed:THRU:PORTs? \nReturn Type Numeric \nDefault Port pairings that were used in the previous cal. \nLast modified: \nApril 14, 2007 Added Cal Set by name and isolation commands \n8-Mar-2007 Added CMethod and TMethod \nOct 23, 2006 Fixed wording in Conn:Port:Sel \n1659\n\nSense:Correction:CKIT Commands \nManages the list of cal kits that are installed in the PNA. \nClick on a blue keyword to view the command details. \nNew See Calibrating the PNA Using SCPI \nLearn about Modifying Cal Kits \nSynchronizing the PNA and Controller \nSCPI Command Tree \nSENSe:CORRection:CKIT:CLEar[:IMMediate] \n(Write-only) Deletes ALL installed cal kits. \nExamples SENS:CORR:CKIT:CLE \nQuery Syntax Not Applicable \nDefault Not Applicable \nSENSe:CORRection:CKIT:COUNt? \n(Read-only) Returns the number of installed cal kits. \nExamples SENS:CORR:CKIT:COUNt? \nQuery Syntax SENS:CORR:CKIT:COUNt? \nReturn Type Numeric \nDefault Not Applicable \n1660\n\nSENSe:CORRection:CKIT:ECAL<mod>:CLISt? \n(Read-only) Returns a list of characterizations stored in the specified ECal module. \nParameters \n<mod> ECal module from which to read user characterization numbers. If unspecified, \nvalue is set to 1. \nExamples Module 1 contains User Characterizations 1 and 3. \nSENSe:CORRection:CKIT:ECAL:CLIST? \n'Returns the following (0 always indicates the factory \ncharacterization): \n0,1,3 \nReturn Type Numeric list, separated by commas. \nDefault Not Applicable \nSENSe:CORRection:CKIT:ECAL<mod>:INFormation? [<char>] \n(Read-only) Reads the user-characterization information from the specified ECal module. This \ncommand returns the same values as SENS:CORR:COLL:CKIT:INF? \nParameters \n<mod> ECal module to read characterizations from. Choose from: \n1 through 8. If unspecified, value is set to 1. \n<char> Optional argument. Specifies which characterization within the ECal module to \nread information from. If not specified, value is set to CHAR0. \nChoose from: \nCHAR0 Factory characterization (data that was stored in the ECal module by \nAgilent) \nCHAR1 User characterization #1 \nCHAR2 User characterization #2 \nCHAR3 User characterization #3 \nCHAR4 User characterization #4 \nCHAR5 User characterization #5 \nExamples SENS:CORR:CKIT:ECAL2:INFormation? char5 \n1661\n\n'Example return string: \nModelNumber: 85092-60007, SerialNumber: 01386, ConnectorType: \nN5FN5F, PortAConnector: Type N (50) female, PortBConnector: Type \nN (50) female, MinFreq: 30000, MaxFreq: 9100000000, \nNumberOfPoints: 250, Calibrated: July 4 2002 \nReturn Type Character \nDefault Not Applicable \nSENSe:CORRection:CKIT:ECAL:LIST? \n(Read-only) Returns a list of index numbers to be used for referring to the ECal modules that are \ncurrently attached to the PNA. \nExamples SENS:CORR:CKIT:ECAL:LIST? \n'If 2 modules are attached to the PNA \n'then the returned list will be: \n1,2 \nReturn Type Numeric list, separated by commas. \nDefault Not Applicable \nSENSe:CORRection:CKIT:ECAL[num]:PATH:COUNt? <path> \n(Read-only) Returns the number of unique states that exist for the specified path name on the selected \nECal module. \nThis command performs exactly the same function as CONT:ECAL:MOD:PATH:COUNt? \nUse the CONT:ECAL:MOD:PATH:STAT command to set the module into one of those states. \nUse SENS:CORR:CKIT:ECAL:PATH:DATA? to read the data for a state. \nParameters \n[num] Optional argument. USB number of the ECal module. If unspecified (only one \nECal module is connected to the USB), <num> is set to 1. If two or more \nmodules are connected, use SENS:CORR:CKIT:ECAL:LIST? to determine \nhow many, and SENS:CORR:CKIT:ECAL:INF? to verify their identities. \n<path> Name of the path for which to read number of states. Choose from: \nReflection paths \n1662\n\nA\nB\nC (4-port modules) \nD (4-port modules) \nTransmission paths \nAB \nAC (4-port modules) \nAD (4-port modules) \nBC (4-port modules) \nBD (4-port modules) \nCD (4-port modules) \nExamples CONT:ECAL:MOD:PATH:COUNt? \ncontrol:ecal:module2:path:count? \nReturn Type Integer \nDefault Not Applicable \nSENSe<ch>:CORRection:CKIT:ECAL[num]:PATH:DATA? <path>, <stateNum>|,<char>| \n(Read-only) Returns the data for a state from the memory of the selected ECal module. The returned \ndata is interpolated if necessary to have the same stimulus values as the specified channel <ch>. \nFor a reflection path state, the data is reflection S-parameter data. The number of values equals the \nnumber of stimulus points on the channel multiplied by 2 (because they are complex numbers). \nFor a transmission path state, the data is all 4 S-parameters of the state. The number of values returned is \n4 times that of a reflection state. \nThe data is returned in the same format as CALC:DATA:SNP? \nNote: This command returns SNP data without header information, and in columns, not in rows as \n.SnP files. This means that the data returned from this command sends all frequency data, then all Sx1 \nmagnitude data, then all Sx1 phase data, and so forth. \nParameters \n<ch> Any existing channel number. If unspecified, value is set to 1. \n1663\n\n[num] Optional argument. USB number of the ECal module. If unspecified (only one \nECal module is connected to the USB), <num> is set to 1. If two or more \nmodules are connected, use SENS:CORR:CKIT:ECAL:LIST? to determine \nhow many, and SENS:CORR:CKIT:ECAL:INF? to verify their identities. \n<path> Name of the path for which to read number of states. Choose from: \nReflection paths \nA\nB\nC (4-port modules) \nD (4-port modules) \nTransmission paths \nAB \nAC (4-port modules) \nAD (4-port modules) \nBC (4-port modules) \nBD (4-port modules) \nCD (4-port modules) \n<stateNum> Number of the state to set. Refer to the following table to associate the \n<stateNum> with a state in your ECal module. \nIn addition, CONT:ECAL:MOD:PATH:COUNt? returns the number of states \nin the specified ECal module. \n1664\n\n<stateNum> N4432A \nand \nN4433A \nStates \nN4431A \nStates \nN469x \nStates** \n8509x \nStates \nOne-Port Reflection States \n1 Open Open Impedance \n1 \nOpen \n2 Short Short Impedance \n2 \nShort \n3 Impedance \n1 \nImpedance \n1 \nImpedance \n3 \nImpedance \n1 \n4 Impedance \n2 \nImpedance \n2 \nImpedance \n4 \nImpedance \n2 \n5 Impedance \n5 \n6 Impedance \n6 \n7 Impedance \n7 \nTwo-Port Transmission States \n1 Thru Thru Thru Thru \n2 Confidence Confidence Confidence Confidence \n** The following modules have only FOUR Impedance states (1, 2, 3, 4): \nN4690B ,N4691B ,N4692A ,N4696B. \n<char> Optional argument. Specifies which characterization within the ECal module to \nread information from. If not specified, value is set to CHAR0. \nChoose from: \nCHAR0 Factory characterization (data that was stored in the ECal module by \nAgilent) \nCHAR1 User characterization #1 \nCHAR2 User characterization #2 \nCHAR3 User characterization #3 \nCHAR4 User characterization #4 \nCHAR5 User characterization #5 \n1665\n\nExamples SENS:CORR:CKIT:ECAL1:PATH:DATA? \nReturn Type S1P or S2P \nDefault Not Applicable \nSENSe:CORRection:CKIT:IMPort <string> \n(Write-only) Imports the specified cal kit (.ckt file) and appends the imported kit to the end of the list \nof kits whenever the file import succeeds. \nParameters \n<string> Path and cal kit name. \nExamples SENSe:CORRection:CKIT:IMPort \"C:/Program Files/Agilent/Network \nAnalyzer/Documents/85033D.ckt\" \nQuery Syntax Not Applicable \nDefault Not Applicable \nSENSe:CORRection:CKIT:INITialize[:IMMediate] \n(Write-only) Restores all default factory installed cal kits. \nParameters \nExamples SENS:CORR:CKIT:INITialize \nsense:correction:ckit:initialize \nQuery Syntax Not Applicable \nDefault Not Applicable \nSENSe:CORRection:CKIT:LOAD <string> \n(Write-only) Loads the specified collection of cal kits from a .wks file. You can make your own \ncollection of cal kits from the Advanced Modify Cal Kit menu. \nParameters \n<string> Path and file name of the cal kit collection. \nExamples sense:correction:ckit:load \"C:/Program Files/Agilent/Network \nAnalyzer/PnaCalKits/factory/wMyCalKits.wks \nQuery Syntax Not Applicable \nDefault Not Applicable \n1666\n\nLast modified: \n10/16/06 Modified Ecal:Data to include <ch> \n1667\n\nSense:Correction:Collect:Ckit Commands \nUse to change the definitions of calibration kit standards. \nClick on a blue keyword to view the command details. \nMost of these commands act on the currently selected standard from the currently selected calibration \nkit. \nTo select a Calibration kit, use SENS:CORR:COLL:CKIT:SEL. \nTo select a Calibration standard, use SENS:CORR:COLL:CKIT:STAN:SEL \nSee an example program that CREATES a New Cal Kit \nSee an example program that MODIFIES an Existing Cal Kit \nLearn about Modifying Cal Kits \nSynchronizing the PNA and Controller \nSCPI Command Tree \nNote: You should provide data for every definition field - for every standard in your calibration kit. If a \nfield is not set, the default value may not be what you expect. \nSENSe:CORRection:COLLect:CKIT:CONNector:ADD \n<family>,<start>,<stop>,<z0>,<gender>,<media>,<cutoff> \n1668\n\n(Write only) Creates a new connector. The connector is automatically added to the list of available \nconnectors for the currently selected cal kit. If a connector includes both male and female connectors, \neach connector must be added separately. \nParameters \n<family> (String) Name of connector family. Limited to 50 characters. \n<start> Start frequency \n<stop> Stop frequency \n<z0> Characteristic Impedance of the connector in ohms. \n<gender> Connector gender. Choose from: \nMALE \nFEMALE \nNONE \n<media> Media of the connector. Choose from: \nCOAX - coaxial \nWAVE - waveguide \n<cutoff> Cutoff frequency of the connector (waveguide only). \nExamples SENS:CORR:COLL:CKIT:CONN:ADD \"PSC 1.8 mm\",0 HZ,999.9 \nGHZ,50,FEMALE,COAX,0.0 \nSENS:CORR:COLL:CKIT:CONN:ADD \"PSC 1.8 mm\",0 HZ,999.9 \nGHZ,50,MALE,COAX,0.0 \nQuery Syntax Not applicable \nDefault Not Applicable \nSENSe:CORRection:COLLect:CKIT:CONNector:CATalog? \n1669\n\n(Read-only) Returns a comma-separated list of all connectors defined within the currently selected cal \nkit. The returned string includes the connector family name followed by the connector gender, if any. \nKits may include a primary connector family name and additional connector family names. \nConnector family names are case sensitive. A connector family named \"PSC 2.4\" is different from a \nconnector family named \"psc 2.4\". \nLearn more about Connector Family Name \nExamples SENS:CORR:COLL:CKIT:CONN:CAT? \n'Returned string \n\"Type-N (50) male, Type-N (50) female\" \nDefault Not Applicable \nSENSe:CORRection:COLLect:CKIT:CONNector:DELete \n(Write-only) Deletes the primary connector family name from the selected kit. The PNA allows \nmultiple connector families for each kit. If a kit includes multiple connector families, only the first \nlisted (primary) connector family name is deleted. \nOnce the connector family is deleted, the connector may not be assigned to any new or existing \nstandard within the kit. \nThe previously defined standards retain their association to the deleted connector name. To reassign \nstandards to a new connector family name, use SENS:CORR:COLL:CKIT:CONN:SNAMe. \nExamples SENS:CORR:COLL:CKIT:CONN:DEL \nQuery Syntax Not Applicable \nDefault Not Applicable \nSENSe:CORRection:COLLect:CKIT:CONNector:FNAME <name> \n1670\n\n(Read-Write) Replaces the primary connector family name from the selected kit with a new connector \nfamily name. The connector family name is replaced in all standards in the kit that share that name. \nThe PNA allows multiple connector families for each kit. If a kit includes multiple connector \nfamilies, only the first listed (primary) connector family name is replaced. Use the query form of this \ncommand to return the name of the primary connector family. \nParameters \n<name> New connector family name. Limited to 50 characters. \nExamples SENS:CORR:COLL:CKIT:CONN:FNAM 'MYPSC35' \nSense:correction:collect:ckit:connector:name 'My Type N' \nQuery Syntax SENSe:CORRection:COLLect:CKIT:CONNector:FNAMe? \nReturn Type String \nDefault Not Applicable \nSENSe:CORRection:COLLect:CKIT:CONNector:SNAMe <family>,<gender>,<port> \n(Read-Write) Assigns a family name to the currently selected standard from the currently selected kit. \nSpecify each port of a 2-port standard individually. Use the query form of this command to read the \nconnector family name assigned to the current standard. The name is not assigned unless the \nconnector family name is previously defined within the selected kit. \nParameters \n<family> String. Connector family name. \n<gender> Connector gender. Choose from: \nMALE \nFEMALE \nNONE \n<port> Number of the connector port to be assigned the connector family name. 2-port \nstandards such as a thru line must be assigned separately. It is not relevant \nwhich connector is port 1 or port 2. \n1 Specifies a 1-port standard or the first port of a 2-port standard. \n2 Specifies the second port of a 2-port standard. \nExamples SENS:CORR:COLL:CKIT:CONN:SNAMe \"Type-N (50)\",MALE,1 \nQuery Syntax SENSe:CORRection:COLLect:CKIT:CONNector:SNAMe? \nReturn Type String \n1671\n\nDefault Not Applicable \nSENSe:CORRection:COLLect:CKIT:DESCription <string> \n(Read-Write) Modifies the cal kit description field of the selected kit. This description appears in the \nEdit PNA Cal Kit dialog box. \nParameters \n<string> Description of the cal kit. Limited to 50 characters. \nExamples SENS:CORR:COLL:CKIT:DESC \"My New CalKit\" \nQuery Syntax SENSe:CORRection:COLLect:CKIT:DESCription? \nReturn Type String \nDefault Not Applicable \nSENSe:CORRection:COLLect:CKIT:INFormation? <module>[,char] \n(Read Only) Reads characterization information from an ECal module. \nParameters \n<module> Specifies which ECal module to read from. Choose from: \nECAL1 \n.through. \nECAL8 \n[char] \nOptional argument. \nSpecifies which characterization within the ECal module to read information \nfrom. If this argument is not used, the default is CHAR0. CHAR1 through \nCHAR5 are for user characterizations that may have been written to the \nmodule by the User Characterization feature on the PNA. Choose from: \nCHAR0 Factory characterization (data that was stored in the ECal module by \nAgilent) \nCHAR1 User characterization #1 \nCHAR2 User characterization #2 \nCHAR3 User characterization #3 \n1672\n\nCHAR4 User characterization #4 \nCHAR5 User characterization #5 \nExamples SENS:CORR:COLL:CKIT:INF? ECAL4 \nsense:correction:collect:ckit:information? ecal2,char1 \nExample return string: \nModelNumber: 85092-60007, SerialNumber: 01386, ConnectorType: \nN5FN5F, PortAConnector: Type N (50) female, PortBConnector: Type \nN (50) female, MinFreq: 30000, MaxFreq: 9100000000, \nNumberOfPoints: 250, Calibrated: July 4 2002 \nReturn Type Character \nDefault Not Applicable \nSENSe:CORRection:COLLect:CKIT:NAME <name> \n(Read-Write) Sets a name for the selected calibration kit. \nParameters \n<name> Calibration Kit name. Any string name, can include numerics, period, and \nspaces; any length (although the dialog box display is limited to about 30 \ncharacters). \nExamples SENS:CORR:COLL:CKIT:NAME 'MYAPC35' \nsense:correction:collect:ckit:name 'mytypen' \nQuery Syntax SENSe:CORRection:COLLect:CKIT:NAME? \nReturn Type String \nDefault Not Applicable \nSENSe:CORRection:COLLect:CKIT:OLABel<class> <name> \n(Read-Write) Sets the label for the calibration class designated by <class>. The label is used in the \nprompts for connecting the calibration standards associated with that <class>. \nParameters \n<class> Number of the calibration class. Choose a number between: 1 and 18. The \n<class> numbers are associated with the following calibration Classes: \n1673\n\nClass Description \n1 S11A Reflection standard \n2 S11B Reflection standard \n3 S11C Reflection standard \n4 S21T Thru/Delay standard \n5 S22A Reflection standard \n6 S22B Reflection standard \n7 S22C Reflection standard \n8 S12T Thru/Delay standard \n3-port analyzers only \n9 S33A Reflection standard \n10 S33B Reflection standard \n11 S33C Reflection standard \n12 S32T Thru/Delay standard \n13 S23T Thru/Delay standard \n14 S31T Thru/Delay standard \n15 S13T Thru/Delay standard \nTRL Calibrations \n16 TRL \"T\" Thru standard \n17 TRL \"R\" Reflect standard \n18 TRL \"L\" Line standard \n<name> Label for the calibration class. Must be enclosed in quotes. Any string \nbetween 1 and 12 characters long. Cannot begin with a numeric. \nExamples SENS:CORR:COLL:CKIT:OLAB3 'LOADS' \nsense:correction:collect:ckit:olabel4 'Thru' \nReturn Type String \nDefault Not Applicable \nSENSe:CORRection:COLLect:CKIT:OLIST[class]? \n(Read-only) Returns seven values of standards that are assigned to the specified class. \nParameters \n<class> Number of the calibration class to be queried. The <class> numbers are \nassociated with the following calibration Classes: \n1674\n\nClass Description \n1 S11A Reflection standard \n2 S11B Reflection standard \n3 S11C Reflection standard \n4 S21T Thru/Delay standard \n5 S22A Reflection standard \n6 S22B Reflection standard \n7 S22C Reflection standard \n8 S12T Thru/Delay standard \n3-port analyzers ONLY \n4-port analyzers use S11 and S22 classes (see example program) \n9 S33A Reflection standard \n10 S33B Reflection standard \n11 S33C Reflection standard \n12 S32T Thru/Delay standard \n13 S23T Thru/Delay standard \n14 S31T Thru/Delay standard \n15 S13T Thru/Delay standard \nTRL Calibrations \n16 TRL \"T\" Thru standard \n17 TRL \"R\" Reflect standard \n18 TRL \"L\" Thru standard \nExamples SENS:CORR:COLL:CKIT:OLIST8? \nAlways returns 7 standard numbers. Unassigned standards return 0 \nReturn Type Numeric; returns the <class> number of the selected standard. \nDefault Not Applicable \nSENSe:CORRection:COLLect:CKIT:ORDer<class> <std> [,<std>] [,<std>] [,<std>] [,<std>] \n[,<std>] [,<std>] \n1675\n\n(Read-Write) Sets a standard number to a calibration class. Does NOT set or dictate the order for \nmeasuring the standards. For more information, see Assigning Standards to a Calibration Class \nParameters \n<class> Number of the calibration class that is assigned to <standard>. Choose a \nnumber between: 1 and 18. The <class> numbers are associated with the \nfollowing calibration Classes: \nClass Description \n1 S11A Reflection standard \n2 S11B Reflection standard \n3 S11C Reflection standard \n4 S21T Thru/Delay standard \n5 S22A Reflection standard \n6 S22B Reflection standard \n7 S22C Reflection standard \n8 S12T Thru/Delay standard \n3-port analyzers ONLY \n4-port analyzers use S11 and S22 classes (see example program) \n9 S33A Reflection standard \n10 S33B Reflection standard \n11 S33C Reflection standard \n12 S32T Thru/Delay standard \n13 S23T Thru/Delay standard \n14 S31T Thru/Delay standard \n15 S13T Thru/Delay standard \nTRL Calibration \n16 TRL \"T\" Thru standard \n17 TRL \"R\" Reflect standard \n18 TRL \"L\" Line standard \n1676\n\n<std> Standard number to be assigned to the class; Choose a standard between 1 and \n8. One standard is mandatory; up to six additional standards are optional. \nExamples Assigns standard 3 to S11A class: \nSENS:CORR:COLL:CKIT:ORD1 3 \nAssigns standard 2 and 5 to S21T class class: \nsense:correction:collect:ckit:order4 2,5 \nQuery Syntax SENSe:CORRection:COLLect:CKIT:ORDer<class>? \n'Returns only the first standard assigned to the specified class. To \nquery the remaining standards, use \nSENSe:CORRection:COLLect:CKIT:OLIST[1-15]? \nReturn Type Numeric \nDefault Not Applicable \nSENSe:CORRection:COLLect:CKIT:RESet <num> - Superseded \nThis command is replaced by Sens:Corr:Ckit:Init. \n(Write-only) Resets the selected calibration kit to factory default definition values. \nParameters \n<num> The number of the calibration kit to be reset. Choose any integer between: \n1 and 8 \nExamples SENS:CORR:COLL:CKIT:RESet 1 \nsense:correction:collect:ckit:reset 4 \nQuery Syntax Not Applicable \nDefault Not Applicable \nSENSe:CORRection:COLLect:CKIT[:SELect] <num> \n1677\n\n(Read-Write) Selects (makes active) a calibration kit for performing a calibration or for modifying \nstandards. All subsequent \"CKIT\" commands that are sent apply to this selected calibration kit. Select \na calibration standard using SENS:CORR:COLL:CKIT:STAN <num> \nParameters \n<num> The number of the calibration kit. Choose from: \nUse SENSe:CORRection:COLLect:CKIT:RESet to restore Cal Kits to default \nvalues. \nName \n1 User Defined 1 \n2 User Defined 2 \n3 User Defined 3 \n'' \n'' \n48 User Defined 48 \n49 User Defined 49 \n50 User Defined 50 \n99 ECAL module \nExamples SENS:CORR:COLL:CKIT 2 \nsense2:correction:collect:ckit:select 7 \nQuery Syntax SENSe:CORRection:COLLect:CKIT? \nReturn Type Numeric \nDefault Last kit selected \nSENSe:CORRection:COLLect:CKIT:STANdard:C0 <num> \n1678\n\n(Read-Write) Sets the C0 value (the first capacitance value) for the selected standard. For a detailed \ndiscussion of this value, search for App Note 8510-5B at www.Agilent.com. \nParameters \n<num> Value for C0 in femtofarads (1E-15) \nExamples The following commands set C0=15 femtofarads: \nSENS:CORR:COLL:CKIT:STAN:C0 15 \nsense:correction:collect:ckit:standard:c0 15 \nQuery Syntax SENSe:CORRection:COLLect:CKIT:STANdard:C0? \nReturn Type Numeric \nDefault Not Applicable \nSENSe:CORRection:COLLect:CKIT:STANdard:C1 <num> \n(Read-Write) Sets the C1 value (the second capacitance value) for the selected standard. For a detailed \ndiscussion of this value, search for App Note 8510-5B at www.Agilent.com. \nParameters \n<num> Value for C1. \nExamples The following two commands set C1=15: \nSENS:CORR:COLL:CKIT:STAN:C1 15 \nsense:correction:collect:ckit:standard:c1 15 \nQuery Syntax SENSe:CORRection:COLLect:CKIT:STANdard:C1? \nReturn Type Numeric \nDefault Not Applicable \nSENSe:CORRection:COLLect:CKIT:STANdard:C2 <num> \n1679\n\n(Read-Write) Sets the C2 value (the third capacitance value) for the selected standard. For a detailed \ndiscussion of this value, search for App Note 8510-5B at www.Agilent.com. \nParameters \n<num> Value for C2. \nExamples The following two commands set C2: \nSENS:CORR:COLL:CKIT:STAN:C2 15 \nsense:correction:collect:ckit:standard:c2 15 \nQuery Syntax SENSe:CORRection:COLLect:CKIT:STANdard:C2? \nReturn Type Numeric \nDefault Not Applicable \nSENSe:CORRection:COLLect:CKIT:STANdard:C3 <num> \n(Read-Write) Sets the C3 value (the fourth capacitance value) for the selected standard. For a detailed \ndiscussion of this value, search for App Note 8510-5B at www.Agilent.com. \nParameters \n<num> Value for C3. \nExamples The following two commands set C3 \nSENS:CORR:COLL:CKIT:STAN:C3 15 \nsense:correction:collect:ckit:standard:c3 15 \nQuery Syntax SENSe:CORRection:COLLect:CKIT:STANdard:C3? \nReturn Type Numeric \nDefault Not Applicable \nSENSe:CORRection:COLLect:CKIT:STANdard:CHARacter <char> \n1680\n\n(Read-Write) Sets the media type of the selected calibration standard. \nParameters \n<char> Media type of the standard. Choose from: \nCoax - Coaxial Cable \nWave - Waveguide \nExamples SENS:CORR:COLL:CKIT:STAN:CHAR COAX \nsense:correction:collect:ckit:standard:character wave \nQuery Syntax SENSe:CORRection:COLLect:CKIT:STANdard:CHARacter? \nReturn Type Numeric \nDefault Coax \nSENSe:CORRection:COLLect:CKIT:STANdard:DELay <num> \n(Read-Write) Sets the electrical delay value for the selected standard. \nParameters \n<num> Electrical delay in picoseconds \nExamples The following two commands set delay to 50 picoseconds \nSENS:CORR:COLL:CKIT:STAN:DEL 50e-12 \nsense2:correction:collect:ckit:standard:delay 50ps \nQuery Syntax SENSe:CORRection:COLLect:CKIT:STANdard:DELay? \nReturn Type Numeric \nDefault Not Applicable \nSENSe:CORRection:COLLect:CKIT:STANdard:FMAX <num> \n1681\n\n(Read-Write) Sets the maximum frequency for the selected standard. \nParameters \n<num> Maximum frequency in Hertz. \nExamples SENS:CORR:COLL:CKIT:STAN:FMAX 9e9 \nsense:correction:collect:ckit:standard:fmax 9Ghz \nQuery Syntax SENSe:CORRection:COLLect:CKIT:STANdard:FMAX? \nReturn Type Numeric \nDefault Not Applicable \nSENSe:CORRection:COLLect:CKIT:STANdard:FMIN <num> \n(Read-Write) Sets the minimum frequency for the selected standard. \nParameters \n<num> Minimum frequency in Hertz. \nExamples SENS:CORR:COLL:CKIT:STAN:FMIN 1e3 \nsense:correction:collect:ckit:standard:fmin 1khz \nQuery Syntax SENSe:CORRection:COLLect:CKIT:STANdard:FMIN? \nReturn Type Numeric \nDefault Not Applicable \nSENSe:CORRection:COLLect:CKIT:STANdard:IMPedance <num> \n(Read-Write) Sets the characteristic impedance for the selected standard. \nParameters \n<num> Impedance in Ohms \nExamples SENS:CORR:COLL:CKIT:STAN:IMP 75 \nsense:correction:collect:ckit:standard:impedance 50.3 \nQuery Syntax SENSe:CORRection:COLLect:CKIT:STANdard:IMPedance? \nReturn Type Numeric \nDefault 50 \nSENSe:CORRection:COLLect:CKIT:STANdard:L0 <num> \n1682\n\n(Read-Write) Sets the L0 value (the first inductance value) for the selected standard. For a detailed \ndiscussion of this value, search for App Note 8510-5B at www.Agilent.com. \nParameters \n<num> Value for L0 in femtohenries (1E-15) \nExamples The following two commands set L0=15 femtohenries: \nSENS:CORR:COLL:CKIT:STAN:L0 15 \nsense:correction:collect:ckit:standard:l0 15 \nQuery Syntax SENSe:CORRection:COLLect:CKIT:STANdard:L0? \nReturn Type Numeric \nDefault Not Applicable \nSENSe:CORRection:COLLect:CKIT:STANdard:L1 <num> \n(Read-Write) Sets the L1 value (the second inductance value) for the selected standard. For a detailed \ndiscussion of this value, search for App Note 8510-5B at www.Agilent.com. \nParameters \n<num> Value for L1. \nExamples The following two commands set L1=15: \nSENS:CORR:COLL:CKIT:STAN:L1 15 \nsense:correction:collect:ckit:standard:l1 15 \nQuery Syntax SENSe:CORRection:COLLect:CKIT:STANdard:L1? \nReturn Type Numeric \nDefault Not Applicable \nSENSe:CORRection:COLLect:CKIT:STANdard:L2 <num> \n1683\n\n(Read-Write) Sets the L2 value (the third inductance value) for the selected standard. For a detailed \ndiscussion of this value, search for App Note 8510-5B at www.Agilent.com. \nParameters \n<num> Value for L2. \nExamples The following two commands set L2=15: \nSENS:CORR:COLL:CKIT:STAN:L2 15 \nsense:correction:collect:ckit:standard:l2 15 \nQuery Syntax SENSe:CORRection:COLLect:CKIT:STANdard:L2? \nReturn Type Numeric \nDefault Not Applicable \nSENSe:CORRection:COLLect:CKIT:STANdard:L3 <num> \n(Read-Write) Sets the L3 value (the fourth inductance value) for the selected standard. For a detailed \ndiscussion of this value, search for App Note 8510-5B at www.Agilent.com. \nParameters \n<num> Value for L3. \nExamples The following two commands set L3=15: \nSENS:CORR:COLL:CKIT:STAN:L3 15 \nsense:correction:collect:ckit:standard:l3 15 \nQuery Syntax SENSe:CORRection:COLLect:CKIT:STANdard:L3? \nReturn Type Numeric \nDefault Not Applicable \nSENSe:CORRection:COLLect:CKIT:STANdard:LABel <name> \n1684\n\n(Read-Write) Sets the label for the selected standard. The label is used to prompt the user to connect \nthe specified standard. \nParameters \n<name> Label for the standard; Must be enclosed in quotes. Any string between 1 and \n12 characters long. Cannot begin with a numeric. \nExamples SENS:CORR:COLL:CKIT:STAN:LAB 'OPEN' \nsense:correction:collect:ckit:standard:label 'Short2' \nQuery Syntax SENSe:CORRection:COLLect:CKIT:STANdard:LABel? \nReturn Type String \nDefault Not Applicable \nSENSe:CORRection:COLLect:CKIT:STANdard:LOSS <num> \n(Read-Write) Sets the insertion loss for the selected standard. \nParameters \n<num> Insertion loss in Gohms / sec. (GigaOhms per second of electrical delay) \nExamples SENS:CORR:COLL:CKIT:STAN:LOSS 3.5e9 \nsense:correction:collect:ckit:standard:loss 3 \nQuery Syntax SENSe:CORRection:COLLect:CKIT:STANdard:LOSS? \nReturn Type Numeric \nDefault Not Applicable \nSENSe:CORRection:COLLect:CKIT:STANdard:REMove \n(Write only) Deletes the selected standard from the selected cal kit. \nExamples SENS:CORR:COLL:CKIT:STAN:REMove \nDefault Not Applicable \nSENSe:CORRection:COLLect:CKIT:STANdard:SDEScription <string> \n1685\n\n(Read-Write) Modifies the description of the selected standard of the selected kit. This description \nappears in the edit kit dialog box. \nParameters \n<string> Description of the standard. \nExamples SENS:CORR:COLL:CKIT:STAN:SDES \"My New Standard\" \nQuery Syntax SENSe:CORRection:COLLect:STANdard:SDEScription? \nReturn Type String \nDefault Not Applicable \nSENSe:CORRection:COLLect:CKIT:STANdard[:SELECT] <num> \n(Read-Write) Selects the calibration standard. All subsequent \"CKIT\" commands to modify a standard \nwill apply to the selected standard. Select a calibration kit using SENS:CORR:COLL:CKIT:SEL \nParameters \n<num> Number of the standard. Choose any number between: \n1 and 30 \nExamples SENS:CORR:COLL:CKIT:STAN 3 \nsense:correction:collect:ckit:standard:select 8 \nQuery Syntax SENSe:CORRection:COLLect:CKIT:STANdard[:SELect]? \nReturn Type Numeric \nDefault 1 \nSENSe:CORRection:COLLect:CKIT:STANdard:TYPE <char> \n1686\n\n(Read-Write) Sets the type for the selected standard. \nParameters \n<char> Choose from: \nOPEN \nSHORT \nLOAD \nSLOAD (sliding load) \nTHRU (through) \nARBI(arbitrary) \nExamples SENS:CORR:COLL:CKIT:STAN:TYPE LOAD \nsense:correction:collect:ckit:standard:type short \nQuery Syntax SENSe:CORRection:COLLect:CKIT:STANdard:TYPE? \nReturn Type Character \nDefault Not Applicable \nSENSe:CORRection:COLLect:CKIT:STANdard:TZReal <num> \n(Read-Write) Sets the TZReal component value of the Terminal Impedance for the selected standard. \nNote: Only applicable when the Standard Type is set to ARBI \nParameters \n<num> Value for TZReal in Ohms \nExamples The following commands set TZReal=15 Ohms: \nSENS:CORR:COLL:CKIT:STAN:TZReal 15 \nsense:correction:collect:ckit:standard:TZReal 15 \nQuery Syntax SENSe:CORRection:COLLect:CKIT:STANdard:TZReal? \nReturn Type Numeric \nDefault Not Applicable \nSENSe:CORRection:COLLect:CKIT:STANdard:TZImag <num> \n1687\n\n(Read-Write) Sets the TZImag component value of the Terminal Impedance for the selected standard. \nNote: Only applicable when the Standard Type is set to ARBI \nParameters \n<num> Value for TZImag in Ohms \nExamples The following two commands set TZImag=15 Ohms: \nSENS:CORR:COLL:CKIT:STAN:TZImag 15 \nsense:correction:collect:ckit:standard:TZImag 15 \nQuery Syntax SENSe:CORRection:COLLect:CKIT:STANdard:TZImag? \nReturn Type Numeric \nDefault Not Applicable \n1688\n\nSense:Correction:Cset Commands \nPerforms actions on calibration sets. \nClick on a blue keyword to view the command details. \nSee Also \nCreating Cal Sets \nExample Programs \nLearn about Cal Sets \nSynchronizing the PNA and Controller \nSENSe<cnum>:CORRection:CSET:ACTivate <string>, <bool> \nThis command replaces SENS:CORR:CSET:GUID \n(Read-Write) Selects and applies a Cal Set to the specified channel. \nUse SENS:CORR:CSET:CAT? to list the Cal Sets. \nParameters \n<cnum> Any existing channel number. If unspecified, value is set to 1 \n<string> Cal Set to make active. Specify the Cal Set by GUID or Name. Use \nSENS:CORR:CSET:CAT? to list the available Cal Sets in either format. \n<bool> Should the Cal Set stimulus values be applied to the channel. Choose from: \nON (1) Apply the Cal Set stimulus values to the channel. \nOFF (0) Do NOT apply the Cal Set stimulus values. If the Cal Set stimulus \nvalues do not match the channel stimulus values, then the following will occur: \n1689\n\nIf interpolation is ON, then interpolation will be attempted. This may fail if the \nchannel frequency is outside the range of the Cal Set. \nIf interpolation is OFF, the selection will be abandoned and an error is returned: \nExamples SENS:CORR:CSET:ACT \"My2Port\",1 \nsense:correction:cset:activate? name \n'returns \n\"My2Port\" \nQuery Syntax SENSe<cnum>:CORRection:CSET:ACTivate? [GUID|NAME] \nReturns the name of the Cal Set that is applied to the specified channel. Choose \nfrom GUID or NAME to specify which string is returned. If unspecified, the \nGUID of the Cal Set is returned. If no Cal Set is applied to the specified \nchannel, then \"No Calset Selected\" is returned. \nReturn Type String \nDefault Not Applicable \nSENSe:CORRection:CSET:CATalog? [char] \n(Read-only) Returns a list of Cal Sets. \nParameters \n<char> Optional argument. The list is returned in one of the following formats. Both \nreturn comma-separated string lists. \nGUID Cal Sets are listed by GUID (Default if unspecified). \nNAME Cal Sets are listed by Name \nExamples SENS:CORR:CSET:CAT? \n'Returns: \n{FD6F863E-9719-11d5-8D6C-00108334AE96},{1B03B2CE-971A-11d5-8D6C- \n00108334AE96} \nsense2:correction:cset:catalog? name \nDefault Not Applicable \nSENSe<cnum>:CORRection:CSET:CREate [name] \n1690\n\n(Write-only) Creates an empty Cal Set and attaches it to the specified channel. This command is \nONLY necessary before remotely filling the Cal Set with error term data. (For Advanced Users). \nA Cal Set is automatically created, applied to the channel, and saved at the completion of a guided cal \naccording to the preference setting SENS:CORR:PREF:CSET:SAVE. \nParameters \n<cnum> Any existing channel number. If unspecified, value is set to 1 \n[name] Optional argument. Name of the Cal Set. Spaces or punctuation are NOT \nallowed. If unspecified, a unique name is chosen in the form \"Calset_N\" where \nN is a unique number. \nExamples SENS:CORR:CSET:CRE 'My2Port' \nQuery Syntax Not Applicable \nDefault Not Applicable \nSENSe<cnum>:CORRection:CSET:DATA <eterm, portA, portB,>[<param>,] <block> \n(Read-Write) Read or Write a specific error term from/to the Cal Set currently attached to the \nspecified channel. (For Advanced Users). \nParameters \n<cnum> Any existing channel number. If unspecified, value is set to 1 \n<eterm, portA, \nportB> \nError Term, Port pair of the specified error term. \nAlthough not all error terms use two port numbers, two are required by the \nPNA in all cases. Each port number must be between 1 and the number of ports \non the PNA. \nEDIR - directivity \nportA: the port at which directivity is measured \nportB: Not used, but must be a valid PNA port number. \nESRM - source match \nportA: the port at which source match is measured \nportB: Not used, but must be a valid PNA port number. \n1691\n\nERFT - reflection tracking \nportA: the port at which reflection tracking is measured \nportB: Not used, but must be a valid PNA port number. \nELDM - load match \nportA: the port at which load match is measured \nportB: the source port. \nLoad match is measured with a cable connected between the measured port \n(portA) and the source port (portB). \nThe cal system requires that the complete matrix of loadmatch arrays be filled. \nIn most cases you can measure loadmatch once at a port, driven by any other \nport. Then use that data for all variations of the receive port. (The exception is \nthe 3-port PNA models, which requires the loadmatch-measured port to be \ndriven by every other port.) \nFor example: Measure the loadmatch at port2 while driving port1. Then upload \nthis same data to the following arrays: \nELDM,2,1,<data> \nELDM,2,3,<data> \nELDM,2,4,<data> \nETRT - transmission tracking \nportA: the receive port \nportB: the source port for this measurement \nEXTLK - crosstalk \nportA: the receive port \nportB: the source port for this measurement \nERSPT - response tracking. \nportA: Not used, but must be a valid PNA port number. \nportB: Not used, but must be a valid PNA port number. \n1692\n\nERSPI - response isolation. \nportA: Not used, but must be a valid PNA port number. \nportB: Not used, but must be a valid PNA port number. \n<param> <string> - required ONLY when Eterm is response tracking (ERSPT) or \nresponse isolation (ERSPI). Specify the S-parameter, ratio, or unratioed \nmeasurement for which the Eterm applies. \nLogical receiver notation is allowed. Ratioed measurements do not require \nsource port to be specified. \nA full 4-port calibration requires the following terms be uploaded: \nPORT B \n1 2 3 4 \nP\nO\nR\nT \nA \n1 \nEDIR,1,1 \nERFT,1,1 \nESRM,1,1 \nELDM,1,2 \nETRT,1,2 \nEXTLK,1,2 \nELDM,1,3 \nETRT,1,3 \nEXTLK,1,3 \nELDM,1,4 \nETRT,1,4 \nEXTLK,1,4 \n2 \nELDM,2,1 \nETRT,2,1 \nEXTLK,2,1 \nEDIR,2,2 \nERFT,2,2 \nESRM,2,2 \nELDM,2,3 \nETRT,2,3 \nEXTLK,2,3 \nELDM,2,4 \nETRT,2,4 \nEXTLK,2,4 \n3 \nELDM,3,1 \nETRT,3,1 \nEXTLK,3,1 \nELDM,3,2 \nETRT,3,2 \nEXTLK,3,2 \nEDIR,3,3 \nERFT,3,3 \nESRM,3,3 \nELDM,3,4 \nETRT,3,4 \nEXTLK,3,4 \n4 \nELDM,4,1 \nETRT,4,1 \nEXTLK,4,1 \nELDM,4,2 \nETRT,4,2 \nEXTLK,4,2 \nELDM,4,3 \nETRT,4,3 \nEXTLK,4,3 \nEDIR,4,4 \nERFT,4,4 \nESRM,4,4 \nReflection terms \nTransmission terms \nExamples SENS:CORR:CSET:DATA EXTLK,3,1 'cross talk between port 3 receiver \nand port 1 source. \nSENS:CORR:CSET:DATA ERSPT,1,1, \"a3/b4\" 'response tracking term \nfor ratioed measurement of port 4 test receiver over port 3 \nreference receiver. \n1693\n\nQuery Syntax SENSe<cnum>:CORRection:CSET:DATA? <eterm,portA, portB> \nReturn Type Block data \nDefault Not Applicable \nSENSe:CORRection:CSET:DELete <string> \n(Write-only) Deletes a Cal Set from the list of available Cal Sets. \nParameters \n<string> The GUID of the Cal Set to be deleted. The curly brackets and hyphens must \nbe included. Not case sensitive. \nExamples SENS:CORR:CSET:DEL '{2B893E7A-971A-11d5-8D6C-00108334AE96}' \nsense2:correction:cset:delete '{2B893E7A-971A-11d5-8D6C- \n00108334AE96}' \nQuery Syntax Not Applicable \nDefault Not Applicable \nSENSe<cnum>:CORRection:CSET:DESCription <string> \n(Read-Write) Sets or returns the descriptive string assigned to the selected Cal Set. Change this string \nso that you can easily identify each Cal Set. Apply and select the Cal Set using \nSENS:CORR:CSET:ACT. \nParameters \n<cnum> Any existing channel number. If unspecified, value is set to 1 \n<string> The descriptive string associated with the currently-selected Cal Set \nExamples SENS:CORR:CSET:DESC 'MyCalSet' \nsense2:correction:cset:description 'thisCalSet' \nQuery Syntax SENSe<cnum>:CORRection:CSET:DESCription? \nReturn Type String \nDefault Not Applicable \nSENSe<cnum>:CORRection:CSET:GUID <string> Superseded \n1694\n\nThis command is replaced by SENS:CORR:CSET:ACTivate. \n(Read-Write) Selects the Cal Set identified by the string parameter (GUID) and applies it to the \nspecified channel. \nA Cal Set cannot be selected for a channel which is not ON. \nIf the stimulus settings of the selected Cal Set differ from those of the selected channel, the instrument will \nautomatically change the channel's settings to match the Cal Set. \nParameters \n<cnum> Any existing channel number. If unspecified, value is set to 1 \n<string> GUID of the desired Cal Set. The curly brackets and hyphens must be included. \nExamples SENS:CORR:CSET:GUID '{2B893E7A-971A-11d5-8D6C-00108334AE96}' \nsense2:correction:cset:guid '{2B893E7A-971A-11d5-8D6C- \n00108334AE96}' \nQuery Syntax SENSe<cnum>:CORRection:CSET:GUID? \nReturns the GUID of the currently-selected Cal Set for the specified \nchannel. \nReturn Type String \nDefault Not Applicable \nSENSe<cnum>:CORRection:CSET:NAME <string> \n(Read-Write) Sets or queries the name of the Cal Set currently applied to the specified channel. \nParameters \n<cnum> Any existing channel number. If unspecified, value is set to 1 \n<string> Name of the Cal Set. Spaces or punctuation NOT allowed. \nExamples SENS:CORR:CSET:NAME 'MyCalSet' \nsense2:correction:cset:name 'thisCalSet' \nQuery Syntax SENSe<cnum>:CORRection:CSET:NAME? \nReturn Type String \nDefault Not Applicable \nSENSe<cnum>:CORRection:CSET[:SELect] <char> Superseded \n1695\n\nThis command is replaced by MMEM:LOAD \n(Read-Write) Restores a state file from memory. The file name is \"CSETx.cst\" where x is the user \nnumber assigned to <char>, and .cst specifies a cal set and instrument state. This is not the same \nsyntax as a file saved through the default choices from the front panel, which is \"at00x.cst\". For more \ninformation on the file naming syntax, see the MMEMory subsystem. Learn more about \nInstrument/Cal States. \nNote: This command does NOT select a Cal Set for a channel. To select a Cal Set, use \nSENS:CORR:CSET:ACTivate \nParameters \n<cnum> Any existing channel number. If unspecified, value is set to 1 \n<char> Choose from: \nDEF - Presets the analyzer \nUSER01 - Restores User01 calibration data \nUSER02 - Restores User02 calibration data \nthrough... \nUSER10 - Restores User10 calibration data \nExamples SENS:CORR:CSET DEF \nsense2:correction:cset:select user02 \nQuery Syntax SENSe<cnum>:CORRection:CSET[:SELect]? \nReturn Type Character \nDefault DEF \nSENSe<cnum>:CORRection:CSET:SAVE <char> \n1696\n\nThis command is NOT necessary after completion of a calibration. A Cal Set is automatically created, \napplied to the channel, and saved at the completion of a guided cal according to the preference setting \nSENS:CORR:PREF:CSET:SAVE. \n(Read Write) \nSaves the channel's Cal Set to the PNA hard drive. For example, use this command after writing data \nto a Cal Set using SENS:CORR:CSET:DATA (For Advanced Users). \nThe file name is saved as \"CSETx.cst\" where x is the user number assigned to <char>, and .cst \nspecifies a Cal Set and instrument state. This is not the same syntax as a file saved through the default \nchoices from the front panel, which is \"at00x.cst\". For more information on the file naming syntax, \nsee the MMEMory subsystem. Learn more about Instrument/Cal States. \nParameters \n<cnum> Any existing channel number. If unspecified, value is set to 1 \n<char> Choose from: \nUSER01 \nUSER02... \nUSER10 \nExamples SENS:CORR:CSET:SAVE USER03 \nsense2:correction:cset:save user09 \nQuery Syntax SENSe<cnum>:CORRection:CSET:SAVE? \nQueries the last correction set saved. \nReturn Type Character \nDefault Not applicable \nSENSe:CORRection:CSET:TSET:ALLPorts? <cset> \n1697\n\n(Read-only) Reads the port mapping used for the specified Cal Set. The returned values are the \nphysical ports. The POSITION of the returned values corresponds to the logical ports. \nFor example, with an N44xx test set, if the returned string is \"PNA 1,TS 2,PNA 2, TS 4\" this means: \nPNA 1 is assigned to logical port 1 \nTS 2 is assigned to logical port 2 \nPNA 2 is assigned to logical port 3 \nTS 4 is assigned to logical port 4 \nParameters \n<cset> (String) Name or GUID of the Cal Set. Use SENS:CORR:CSET:CAT? to read \nthe list of available Cal Set names or GUIDs. \nExamples SENS:CORR:CSET:TSET:ALLP? \"MyCalSet\" \nsens:correction:cset:tset:allports? \"{2B893E7A-971A-11d5-8D6C- \n00108334AE96}\" \nReturn Type String \nDefault Not Applicable \nSENSe:CORRection:CSET:TSET:TYPE? <cset> \n(Read-only) Reads the test set type (model) used for the specified Cal Set. \nParameters \n<cset> (String) Name or GUID of the Cal Set. Use SENS:CORR:CSET:CAT? to read \nthe list of available Cal Set names or GUIDs. \nExamples SENS:CORR:CSET:TSET:TYPE? \"MyCalSet\" \n'returns \"N44xx\" \nsens:correction:cset:tset:type? \"{2B893E7A-971A-11d5-8D6C- \n00108334AE96}\" \nReturn Type String \nDefault Not Applicable \nSENSe<ch>:CORRection:CSET:TYPE:CATalog? [format] \n1698\n\n(Read-only) Query the Cal Types available in the selected Cal Set. The output is a comma separated \nlist of Guids or a Cal Type names. Learn more about applying Cal Types using SCPI. \nUse CALC:CORR:TYPE to apply a Cal Type. \nParameters \n<ch> Any existing channel number. If unspecified, value is set to 1 \n[format] (Optional) Format of the output of cal types. choose from: \nNAME - (default) returns a list of cal type string names. \nGUID - returns a list of cal type GUIDs \nExamples SENS:CORR:CSET:TYPE:CAT? NAME \nSENS2:CORRection:CSET:TYPE:CAT? \nReturn Type String \nDefault Not Applicable \nLast modified: \n9/12/06 MQ Added TSET commands for multiport. \n1699\n\nSense:Correction:Extension Commands \nPerforms and applies Port Extensions. \nClick on a blue keyword to view the command details. \nSee Also \nExample Programs \nLearn about Port Extensions \nSynchronizing the PNA and Controller \nSCPI Command Tree \nSENSe<cnum>:CORRection:EXTension:AUTO:CONFig <char> \n(Read-Write) Sets the frequencies used to calculate Automatic Port Extension. Learn more about \ncalculating Automatic Port Extension. \nParameters \n<cnum> Any existing channel number. If unspecified, value is set to 1 \n<char> Frequencies to be used: \nCSPN Use current frequency span. \nAMKR - Use active marker frequency. \nUSPN - Use custom user span. Use SENS:CORR:EXT:AUTO:STAR and \nSENS:CORR:EXT:AUTO:STOP to specify start and stop frequency. \nExamples SENS:CORR:EXT:AUTO:CONF CSPN \nsense2:correction:extension:auto:config amkr \nQuery Syntax SENSe<cnum>:CORRection:EXTension:AUTO:CONFig ? \n1700\n\nReturn Type Character \nDefault CSPN \nSENSe<cnum>:CORRection:EXTension:AUTO:DCOFfset <bool> \n(Read-Write) Specifies whether or not to include DC Offset as part of automatic port extension. Learn \nmore about Automatic DC Offset. Only allowed when SENS:CORR:EXT:AUTO:LOSS is set to ON. \nParameters \n<cnum> Any existing channel number. If unspecified, value is set to 1 \n<bool> ON (or 1) - Includes DC Offset correction. \nOFF (or 0) - Does NOT include DC Offset correction. \nExamples SENS:CORR:EXT:AUTO:DCOF 1 \nsense2:correction:extension:auto:dcoffset off \nQuery Syntax SENSe<cnum>:CORRection:EXTension:AUTO:DCOFfset? \nReturn Type Boolean \nDefault OFF (0) \nSENSe<cnum>:CORRection:EXTension:AUTO:LOSS <bool> \n(Read-Write) Specifies whether or not to include loss correction as part of automatic port extension. \nLearn more about Loss Compensation in port extension. \nParameters \n<cnum> Any existing channel number. If unspecified, value is set to 1 \n<bool> ON (or 1) - Includes Loss correction. \nOFF (or 0) - Does NOT include Loss correction. \nExamples SENS:CORR:EXT:AUTO:LOSS 1 \nsense2:correction:extension:auto:loss off \nQuery Syntax SENSe<cnum>:CORRection:EXTension:AUTO:LOSS? \nReturn Type Boolean \nDefault OFF (0) \nSENSe<cnum>:CORRection:EXTension:AUTO:MEASure <char> \n1701\n\n(Write-only) Measures either an OPEN or SHORT standard. When this command is sent, the PNA \nacquires the measurement with which to set automatic port extensions. Learn more about which \nstandard to measure. \nParameters \n<cnum> Any existing channel number. If unspecified, value is set to 1 \n<char> Standard to be measured. Choose from: \nOPEN Measure OPEN standard \nSHORt Measure SHORT standard \nExamples SENS:CORR:EXT:AUTO:MEAS OPEN \nsense2:correction:extension:auto:measure short \nQuery Syntax Not Applicable \nDefault Not Applicable \nSENSe<cnum>:CORRection:EXTension:AUTO:PORT<n> <bool> \n(Read-Write) Enables and disables automatic port extensions on the specified port. \nParameters \n<cnum> Any existing channel number. If unspecified, value is set to 1 \n<n> PNA Port number to enable or disable for automatic port extensions. \n<bool> ON (or 1) - Enable \nOFF (or 0) - Disable \nExamples SENS:CORR:EXT:AUTO:PORT2 0 \nsense2:correction:extension:auto:port4 on \nQuery Syntax SENSe<cnum>:CORRection:EXTension:AUTO:PORT<n>? \nReturn Type Boolean \nDefault All ports ON (enabled) \nSENSe<cnum>:CORRection:EXTension:AUTO:RESet \n1702\n\n(Write-only) Clears old port extension delay and loss data in preparation for acquiring new data. Send \nthis command prior to sending a new series of SENS:CORR:EXT:AUTO:MEAS. If acquiring both \nOPEN and SHORT standards, do not send this command between those acquisitions. \nParameters \n<cnum> Any existing channel number. If unspecified, value is set to 1 \nExamples SENS:CORR:EXT:AUTO:RES \nsense2:correction:extension:auto:reset \nQuery Syntax Not Applicable \nDefault Not Applicable \nSENSe<cnum>:CORRection:EXTension:AUTO:STARt <value> \n(Read-Write) Set the start frequency for custom user span. Learn more about User Span. \nParameters \n<cnum> Any existing channel number. If unspecified, value is set to 1 \n<value> User span start value. Must be within the frequency range of the active channel \nand less than the value set by SENS:CORR:EXT:AUTO:STOP. \nExamples SENS:CORR:EXT:AUTO:STAR 1E9 \nsense2:correction:extension:auto:start 200e6 \nQuery Syntax SENSe<cnum>:CORRection:EXTension:AUTO:STARt <value>? \nReturn Type Numeric \nDefault Start frequency of the current active channel. \nSENSe<cnum>:CORRection:EXTension:AUTO:STOP <value> \n1703\n\n(Read-Write) Set the stop frequency for custom user span. Learn more about User Span. \nParameters \n<cnum> Any existing channel number. If unspecified, value is set to 1 \n<value> User span stop value. Must be within the frequency range of the active channel \nand greater than the value set by SENS:CORR:EXT:AUTO:STARt \nExamples SENS:CORR:EXT:AUTO:STOP 1E9 \nsense2:correction:extension:auto:stop 200e6 \nQuery Syntax SENSe<cnum>:CORRection:EXTension:AUTO:STOP <value>? \nReturn Type Numeric \nDefault Stop frequency of the current active channel. \nSENSe<cnum>:CORRection:EXTension:PORT<pnum>:FREQ<n> <value> \n(Read-Write) Sets and returns the frequency \"Use\" number (1|2) for the specified port number. \nLearn about Loss Compensation values. \nParameters \n<cnum> Any existing channel number. If unspecified, value is set to 1 \n<pnum> Port Number that will receive the freq/loss settings. If unspecified, value is set \nto 1. \n<n> Frequency \"Use\" number. Choose from 1 or 2. If unspecified, value is set to 1. \n<value> Frequency value. Choose a frequency within the frequency span of the PNA. \nExamples SENS:CORR:EXT:PORT1:FREQ1 10E9 \nsense2:correction:extension:port2:freq2:2E10 \nQuery Syntax SENSe<cnum>:CORRection:EXTension:PORT<pnum>:FREQ<n>? \nReturn Type Numeric \nDefault 1 GHz \nSENSe<cnum>:CORRection:EXTension:PORT<pnum>:INCLude<n>:STATe <bool> \n1704\n\n(Read-Write) Sets and returns the ON/OFF state for the use of the Loss and Freq values for the \nspecified port number. \nLearn about Loss Compensation values. \nNote: This command affects ALL measurements on the specified channel. \nParameters \n<cnum> Any existing channel number. If unspecified, value is set to 1 \n<pnum> Port Number that will receive the Freq/Loss settings. If unspecified, value is set to \n1. \n<n> Freq and Loss pair. Choose from 1 or 2. If unspecified, value is set to 1. \n<value> State of Freq and Loss values for port extension. \n0 or OFF Specified Freq and Loss values are OFF \n1 or ON Specified Freq and Loss values are ON \nExamples SENS:CORR:EXT:PORT:INCL 0 \nsense2:correction:extension:port2:include:state on \nQuery Syntax SENSe<cnum>:CORRection:EXTension:PORT<pnum>:INCLude:STATe? \nReturn Type Boolean \nDefault OFF \nSENSe<cnum>:CORRection:EXTension:PORT<pnum>:LDC <value> \n(Read-Write) Sets and returns the Port Loss at DC value for the specified port number. \nLearn about Loss Compensation values. \nNote: This command affects ALL measurements on the specified channel. \nParameters \n<cnum> Any existing channel number. If unspecified, value is set to 1 \n<pnum> Port number to receive Loss value. If unspecified, value is set to 1. \n<value> Loss in dB. Choose a value between -90 and 90 \nExamples SENS:CORR:EXT:PORT:LDC 1.5 \nsense2:correction:extension:port2:ldc .1 \nQuery Syntax SENSe<cnum>:CORRection:EXTension:PORT<pnum>:LDC? \n1705\n\nReturn Type Numeric \nDefault 0 \nSENSe<cnum>:CORRection:EXTension:PORT<pnum>:LOSS<n> <value> \n(Read-Write) Sets and returns the Loss value for the specified port number. \nLearn about Loss Compensation values. \nNote: This command affects ALL measurements on the specified channel. \nParameters \n<cnum> Any existing channel number. If unspecified, value is set to 1 \n<pnum> Port Number that will receive the Freq/Loss settings. If unspecified, value is set \nto 1. \n<n> Loss \"Use\" number. Choose from 1 or 2. If unspecified, value is set to 1. \n<value> Loss in dB. Choose a value between -90 and 90 \nExamples SENS:CORR:EXT:PORT:LOSS1 1 \nsense2:correction:extension:port2:loss2 .1 \nQuery Syntax SENSe<cnum>:CORRection:EXTension:PORT<pnum>:LOSS<n>? \nReturn Type Numeric \nDefault 0 \nSENSe<cnum>:CORRection:EXTension:PORT<pnum>[:TIME] <num> \n1706\n\n(Read-Write) Sets the extension value at the specified port. Must also set SENS:CORR:EXT ON. \nNote: This command affects ALL measurements on the specified channel. \nParameters \n<cnum> Any existing channel number. If unspecified, value is set to 1 \n<pnum> Port Number that will receive the extension. If unspecified, value is set to 1. \n<num> The port extension in seconds; may include suffix. Choose a number between: \n-1E18 and 1E18 \nExamples SENS:CORR:EXT:PORT 2MS \nsense2:correction:extension:port2 .00025 \nQuery Syntax SENSe<cnum>:CORRection:EXTension:PORT<pnum> [:TIME]? \nReturn Type Numeric \nDefault 0 \nSENSe<cnum>:CORRection:EXTension:RECeiver<Rnum>[:TIME] <num> OBSOLETE \n(Read-Write) This command has NO replacement and no longer works. \nSets the extension value at the specified receiver. Must also set SENS:CORR:EXT ON. \nNote: Before using this command you must select a measurement using CALC:PAR:SEL. You can \nselect one measurement for each channel. \nParameters \n<cnum> Any existing channel number. If unspecified, value is set to 1 \n<Rnum> Number of the receiver that will receive the extension. If unspecified, value is \nset to 1 \nChoose from: \n1 for Receiver A \n2 for Receiver B \n<num> The electrical length in seconds; may include suffix. Choose a number \nbetween: \n-10 and 10 \nExamples SENS:CORR:EXT:REC 2MS \nsense2:correction:extension:receiver2:time .00025 \nQuery Syntax SENSe<cnum>:CORRection:EXTension:RECeiver<Rnum> [:TIME]? \n1707\n\nReturn Type Numeric \nDefault 0 \nSENSe<cnum>:CORRection:EXTension[:STATe] <ON | OFF> \n(Read-Write) Turns port extensions ON or OFF. \nParameters \n<cnum> Any existing channel number. If unspecified, value is set to 1 \n<ON | OFF> ON (or 1) - turns port extensions ON. \nOFF (or 0) - turns port extensions is OFF. \nExamples SENS:CORR:EXT ON \nsense2:correction:extension:state off \nQuery Syntax SENSe<cnum>:CORRection:EXTension[:STATe]? \nReturn Type Boolean (1 = ON, 0 = OFF) \nDefault OFF \n1708\n\nSense:Correction:Collect:Session Commands \nThe commands in this topic are common to perform both SMC and VMC calibrations. A calibration \nsession is a term used to describe an instance of a SMC or VMC calibration. For more commands, see \nSESS:SMC and SESS:VMC. \nCommands to read (STEP?) and describe (DESC?) each step are provided to facilitate a remote user \ninterface. \nTo perform a NON - SMC or VMC calibration, use either Guided or Mechanical SCPI commands. \nClick on a blue keyword to view the command details. \nSee Also \nSCPI SMC and VMC calibration examples. \nLearn about SMC and VMC calibrations \nSynchronizing the PNA and Controller \nSCPI Command Tree \nSENSe<ch>:CORRection:COLLect:SESSion<n>:ACQuire <step> \n1709\n\n(Write only) Acquire a calibration measurement. \nParameters \n<ch> Any existing channel number. If unspecified, value is set to 1. \n<n> Session number. Choose from 1 to 16. \n<step> Step number to acquire. Use SENS:CORR:COLL:SESS:STEPS? to find the \nnumber of steps required for the calibration. \nExamples SENSe2:CORR:COLL:SESS6:ACQ 5 \nQuery Syntax Not Applicable \nDefault Not Applicable \nSENSe<ch>:CORRection:COLLect:SESSion<n>:CKIT:PORT<p>:CATalog? \n(Read only) Returns a list of cal kits that are compatible with the connector on port <p>. The port \nconnector type is set with SENS:CORR:COLL:SESS:CONN:PORT \nParameters \n<ch> Any existing channel number. If unspecified, value is set to 1. \n<n> Session number. Choose from 1 to 16. \n<p> Port number of connector to query for compatible cal kits. \nExamples SENS2:CORR:COLL:SESS6:CKIT:PORT2:CAT? \nReturn Type Comma separated string values \nDefault Not Applicable \nSENSe<ch>:CORRection:COLLect:SESSion<n>:CKIT:PORT<p>[:SELect] <calkit> \n1710\n\n(Read-Write) Set or return the Cal Kit for the specified port. Use \nSENS:CORR:COLL:SESS:CKIT:PORT:CAT? to list compatible Cal Kits. \nParameters \n<ch> Any existing channel number. If unspecified, value is set to 1 \n<n> Session number. Choose from 1 to 16. \n<p> Port number for which to set cal kit. \n<calkit> Cal Kit Name \nExamples SENS:CORR:COLL:SESS:CKIT:PORT:SEL 85091A \nSENS2:CORR:COLL:SESS6:CKIT:PORT2:SEL? \nQuery Syntax SENS<ch>:CORR:COLL:SESS<n>:CKIT:PORT<p>[:SEL] ? \nReturn Type String \nDefault Not Applicable \nSENSe<ch>:CORRection:COLLect:SESSion<n>:CONN:PORT<p>[:SEL] <conn> \n(Read-Write) Set the connector type and sex for the specified port number. Catalog valid connector \ntypes using SENS:CORR:COLL:GUID:CONN:CAT? \nParameters \n<ch> Any existing channel number. If unspecified, value is set to 1 \n<n> Session number. Choose from 1 to 16. \n<p> Port number for which to select a connector type. \n<conn> Name of the connector type \nExamples SENS2:CORR:COLL:SESS6:CONN:PORT1:SEL \"N Type\" \nQuery Syntax SENS<ch>:CORR:COLL:SESS<n>:CONN:PORT<p>[:SEL] ? \nReturn Type String \nDefault Not Applicable \nSENSe<ch>:CORRection:COLLect:SESSion<n>:DESC? <step> \n1711\n\n(Read-only) Returns the connection prompt for the step. List the number of steps in the calibration \nusing SENS:CORR:COLL:SESS:STEPS?. \nParameters \n<ch> Any existing channel number. If unspecified, value is set to 1 \n<n> Session number. Choose from 1 to 16. \n<step> Step number \nExamples SENS1:CORR:COLL:SESS6:DESC?3 \nReturn Type Numeric \nDefault Not Applicable \nSENSe<ch>:CORRection:COLLect:SESSion<n>:DONE \n(Write only) Ends the calibration sessions. Use SAVE? to calculate error terms and save the CalSet. \nParameters \n<ch> Any existing channel number. If unspecified, value is set to 1 \n<n> Session number. Choose from 1 to 16. \nExamples SENS1:CORR:COLL:SESS6:DONE \nQuery Syntax Not Applicable \nDefault Not Applicable \nSENSe<ch>:CORRection:COLLect:SESSion<n>:INITiate <string> \n1712\n\n(Write only) Initiates an SMC or VMC calibration session. Use the session number for subsequent \nSMC or VMC commands. \nParameters \n<ch> Any existing channel number. If unspecified, value is set to 1 \n<n> Session number. Choose from 1 to 16. If the session number already exists it \nwill be terminated and a new session initiated. \n<string> Name of the calibration. Choose from: \n\"VMC\" or \"VectorMixerCal.VMCType\" \n\"SMC\" or \"ScalarMixerCal.SMCType\" \nExamples SENS1:CORR:COLL:SESS6:INITiate \"VectorMixerCal.VMCType\" \nQuery Syntax Not Applicable \nDefault Not Applicable \nSENSe<ch>:CORRection:COLLect:SESSion<n>:SAVE? \n(Read only) Finish the SMC or VMC calibration, compute error terms, populate and save the CalSet, \nand return the GUID of the Cal Set. \nNote: The destination (Cal Register or User Cal Set) is determined by the setting of the \nSENS:CORR:PREFerence:CSET:SAVE command. \nParameters \n<ch> Any existing channel number. If unspecified, value is set to 1 \n<n> Session number. Choose from 1 to 16. \nExamples SENS1:CORR:COLL:SESS6:SAVE? \nReturn Type String specifying the GUID of the CalSet produced by this session. \nDefault Not Applicable \nSENSe<ch>:CORRection:COLLect:SESSion<n>:STEPs? \n1713\n\n(Read-only) Returns the number of steps required by the Calibration. \nTo ensure this query always completes successfully, first send the write command: \nSENS:CORR:COLL:SESS:STEP, then send the query. \nParameters \n<ch> Any existing channel number. If unspecified, value is set to 1 \n<n> Session number. Choose from 1 to 16. \nExamples SENS1:CORR:COLL:SESS6:STEPs? \nReturn Type Numeric \nDefault Not Applicable \n1714\n\nSense:Correction:Collect:Session:SMC Commands \nPerforms scalar (SMC) calibration on a frequency converting device. \nClick on a blue keyword to view the command details. \nSee Also \nExample Programs \nLearn about FCA Calibrations \nSynchronizing the PNA and Controller \nSCPI Command Tree \nNOTE: To configure a power meter and sensor see SOURce:POWer: commands. \nSENSe<ch>:CORRection:COLLect:SESSion<n >:SMC:ECAL:CHARacteriza <mod> ,<char> \n1715\n\n(Read-Write) Specifies the ECal module and characterization to be used for the SMC calibration. \nParameters \n<ch> Any existing channel number. If unspecified, value is set to 1 \n<n> Session number. Choose from 1 to 16. Learn about Cal sessions. \n<mod> 1 - Electronic Calibration Module \n<char> Specifies which characterization within the ECal module from which to read \nthe confidence data. \n0 Factory characterization (data that was stored in the ECal module by \nAgilent). Default if not specified. \n1 User characterization #1 \n2 User characterization #2 \n3 User characterization #3 \n4 User characterization #4 \n5 User characterization #5 \nExamples SENS:CORR:COLL:SESS:SMC:ECAL:CHAR 1,2 \nQuery Syntax SENS:CORR:COLL:SESS:SMC:ECAL:CHAR? \nReturn Type Numeric \nDefault 1,0 \nSENSe<ch>:CORRection:COLLect:SESSion<n> :SMC:FSIMulator:NETWork<x>:MODE \n<char> \n1716\n\n(Read-Write) Allows you to embed (add) or de-embed (remove) circuit network effects on the input \nand output of your mixer measurement. Learn more. \nParameters \n<ch> Any existing channel number. If unspecified, value is set to 1 \n<n> Session number. Choose from 1 to 16. Learn about Cal sessions. \n<x> Apply network to input or output of mixer. Choose from: \n1 - Input of mixer \n2 - Output of mixer \n<char> Choose from: \nNONE - Do nothing with effects of S2P file. \nEMBed - Add effects of S2P file from the measurement results. \nDEEMbed - Remove effects of S2P file from the measurement results. \nExamples SENS:CORR:COLL:SESS:SMC:FSIM:NETW1:MODE EMB \nQuery Syntax SENS<ch>:CORRection:COLLect:SESSion<n> \n:SMC:FSIMulator:NETWork<x>:MODE? \nReturn Type Character \nDefault NONE \nSENSe<ch>:CORRection:COLLect:SESSion<n> :SMC:FSIMulator:NETWork<x>:FILename \n<string> \n1717\n\n(Read-Write) Specifies the S2P filename to embed or de-embed on the input or output of your mixer \nmeasurement. Learn more. \nParameters \n<ch> Any existing channel number. If unspecified, value is set to 1 \n<n> Session number. Choose from 1 to 16. Learn about Cal sessions. \n<x> Apply network to input or output of mixer. Choose from: \n1 - Input of mixer \n2 - Output of mixer \n<string> Filename of the S2P used for embedding or de-embedding. Use the full path \nname, file name, and .S2P suffix, enclosed in quotes. \nExamples SENS:CORR:COLL:SESS:SMC:FSIM:NETW1:FIL \"C:\\Program \nFiles\\Agilent\\Network Analyzer\\Documents\\WaveguideAdapt.S2P\" \nQuery Syntax SENS<ch>:CORRection:COLLect:SESSion<n> \n:SMC:FSIMulator:NETWork<x>:FILename? \nReturn Type String \nDefault Not Applicable \nSENSe<ch>:CORRection:COLLect:SESSion<n>:SMC:PWRCal:SRCPort <string> Obsolete \n(Read-Write) Specifies which port to calibrate. \nNote: Beginning with Rev 6.0, this command is no longer necessary. Learn more. Because of \nimproved calibration techniques, Both is always selected although a power meter measurement is \nperformed only on port 1. \nParameters \n<ch> Any existing channel number. If unspecified, value is set to 1 \n<n> Session number. Choose from 1 to 16. Learn about Cal sessions. \n<char> '1' Source port 1 (SMC forward direction) \n'2' Source port 2 (SMC reverse direction \n'BOTH' (both forward and reverse directions) \nExamples SENS:CORR:COLL:SESS:SMC:PWRC:SRCP 'both' \nSENSe2:CORRection:COLLection:SESSion6:SMC:PWRCal:SRCPort '2' \nQuery Syntax SENS:CORR:COLL:SESS:SMC:PWRC:SRCP? \n1718\n\nReturn Type String \nDefault 1 \nSENSe<ch>:CORRection:COLLect:SESSion<n>:SMC:TWOPort:ECAL:ORIentation[:STATe] \n<bool> \n(Read-Write) Sets ECAL Auto-Orientation ON or OFF. If setting auto-orientation OFF, you must \nmanually specify the orientation of the ECAL module with \nSENS:CORR:COLL:SESS:SMC:TWOP:ECAL:PORTmap. \nParameters \n<ch> Any existing channel number. If unspecified, value is set to 1 \n<n> Session number. Choose from 1 to 16. Learn about Cal sessions. \n<bool> 0 = Orientation OFF \n1 = Orientation ON \nExamples SENS:CORR:COLL:SESS:SMC:TWOP:ECAL:ORI 1 \nQuery Syntax SENS:CORR:COLL:SESS:SMC:TWOP:ECAL:ORI? \nReturn Type Boolean \nDefault 1 \nSENSe<ch>:CORRection:COLLect:SESSion<n>:SMC:TWOPort:ECAL:PORTmap <mod>, \n<string> \n(Read-Write) Specifies the manual orientation (which ports of the module are connected to which \nports of the PNA) when auto-orientation is OFF. \nParameters \n<ch> Any existing channel number. If unspecified, value is set to 1 \n<n> Session number. Choose from 1 to 16. Learn about Cal sessions. \n<mod> 1 - Electronic Calibration Module \n<string> Format in the following manner: \nAw,Bx,Cy,Dz \nwhere\nA, B, C, and D are literal ports on the ECAL module \n1719\n\nw,x,y, and z are substituted for PNA port numbers to which the ECAL module port \nis connected. \nPorts of the module which are not used are omitted from the string. \nFor example, on a 4-port ECal module with \nport A connected to PNA port 2 \nport B connected to PNA port 3 \nport C not connected \nport D connected to PNA port 1 \nthe string would be: A2,B3,D1 \nIf either the receive port or source port (or load port for 2-port cal) of the \nCALC:PAR:SELected measurement is not in this string and orientation is OFF, \nan attempt to perform an ECal calibration will fail. \nExamples SENS:CORR:COLL:SESS:SMC:TWOP:ECAL:PORTmap 1,'A1,B2' \nQuery Syntax SENS:CORR:COLL:SESS:SMC:TWOP:ECAL:PORTmap? \nReturn Type String \nDefault \"A1,B2\" \nSENSe<ch>:CORRection:COLLect:SESSion<n >:SMC:TWOPort:METHod <string> \n1720\n\n(Read-Write) Specifies the guided ECal method for performing the thru portion of the calibration. \nParameters \n<ch> Any existing channel number. If unspecified, value is set to 1 \n<n> Session number. Choose from 1 to 16. Learn about Cal sessions. \n<string> ECAL Method: Choose from: \n'DEFAULT' - Default \n'ADAP' - Adapter removal \n'FLUSH' - Flush Through \n'UNKN' - Unknown Thru \nExamples SENS:CORR:COLL:SESS:SMC:TWOPort:METH 'default' \nQuery Syntax SENS:CORR:COLL:SESS:SMC:TWOPort:METH? \nReturn Type String \nDefault DEFAULT \nSENSe<ch>:CORRection:COLLect:SESSion<n >:SMC:TWOPort:OMITisolat <bool> \n(Read-Write) Select to omit or perform the isolation portion of the ECAL. \nParameters \n<ch> Any existing channel number. If unspecified, value is set to 1 \n<n> Session number. Choose from 1 to 16. Learn about Cal sessions. \n<bool> 1 - Omit isolation \n0 - Perform isolation \nExamples SENS:CORR:COLL:SESS:SMC:TWOPort:OMIT 1 \nQuery Syntax SENS:CORR:COLL:SMC:TWOPort:OMIT? \nReturn Type Boolean \nDefault 1 \nSENSe<ch>:CORRection:COLLect:SESSion<n >:SMC:TWOPort:OPTion <string> \n1721\n\n(Read-Write) Sets the SMC calibration to ECAL or MECHanical \nParameters \n<ch> Any existing channel number. If unspecified, value is set to 1 \n<n> Session number. Choose from 1 to 16. Learn about Cal sessions. \n<char> Choose from: \n'ECAL' Electronic Calibration Module \n'MECH' Mechanical Calibration Kit \nExamples SENS:CORR:COLL:SESS:SMC:TWOPort:OPTion 'ECAL' \nQuery Syntax SENS:CORR:COLL:SESS:SMC:TWOPort:OPTion? \nReturn Type String \nDefault ECAL \n1722\n\nSense:Correction:Collect:Session:VMC Commands \nPerforms a vector (VMC) calibration on a frequency converting device. \nClick on a blue keyword to view the command details. \nSee Also \nExample Programs \nLearn about VMC Calibration \nSynchronizing the PNA and Controller \nSENSe<ch>:CORRection:COLLect:SESSion<n> :VMC:FSIMulator:NETWork<x>:MODE \n<char> \n1723\n\n(Read-Write) Allows you to embed (add) or de-embed (remove) circuit network effects on the input \nand output of your mixer measurement. Learn more. \nParameters \n<ch> Any existing channel number. If unspecified, value is set to 1 \n<n> Session number. Choose from 1 to 16. Learn about Cal sessions. \n<x> Apply network to input or output of mixer. Choose from: \n1 - Input of mixer \n2 - Output of mixer \n<char> Choose from: \nNONE - Do nothing with effects of S2P file. \nEMBed - Add effects of S2P file from the measurement results. \nDEEMbed - Remove effects of S2P file from the measurement results. \nExamples SENS:CORR:COLL:SESS:VMC:FSIM:NETW1:MODE EMB \nQuery Syntax SENS<ch>:CORRection:COLLect:SESSion<n> \n:VMC:FSIMulator:NETWork<x>:MODE? \nReturn Type Character \nDefault NONE \nSENSe<ch>:CORRection:COLLect:SESSion<n> :VMC:FSIMulator:NETWork<x>:FILename \n<string> \n1724\n\n(Read-Write) Specifies the S2P filename to embed or de-embed on the input or output of your mixer \nmeasurement. Learn more. \nParameters \n<ch> Any existing channel number. If unspecified, value is set to 1 \n<n> Session number. Choose from 1 to 16. Learn about Cal sessions. \n<x> Apply network to input or output of mixer. Choose from: \n1 - Input of mixer \n2 - Output of mixer \n<string> Filename of the S2P used for embedding or de-embedding. Use the full path \nname, file name, and .S2P suffix, enclosed in quotes. \nExamples SENS:CORR:COLL:SESS:VMC:FSIM:NETW1:FIL \"C:\\Program \nFiles\\Agilent\\Network Analyzer\\Documents\\WaveguideAdapt.S2P\" \nQuery Syntax SENS<ch>:CORRection:COLLect:SESSion<n> \n:VMC:FSIMulator:NETWork<x>:FILename? \nReturn Type String \nDefault Not Applicable \nSENSe<ch>:CORRection:COLLect:SESSion<n> :VMC:MIXer:CHARacterize:CAL:FILename \n<string> \n(Read-Write) Specifies the .S2P filename used for mixer characterization. Use the \nVMC:MIXer:CHARacterize:CAL: OPTion command to recall the file for mixer characterization. \nOnce recalled, use this command to query the current filename or set a new filename. \nParameters \n<ch> Any existing channel number. If unspecified, value is set to 1 \n<n> Session number. Choose from 1 to 16. Learn about Cal sessions. \n<string> Filename of the S2P used for mixer characterization. Use the full path name, \nfile name, and .S2P suffix, enclosed in quotes. \nExamples SENS2:CORR:COLL:SESS4:VMC:MIXer:CHAR:CAL:FILE \"C:\\Program \nFiles\\Agilent\\Network Analyzer\\Documents\\MyMixer.S2P\" \nQuery Syntax SENS:CORR:COLL:SESS:VMC:MIX:CHAR:CAL:FIL? \nReturn Type String \nDefault C:\\Program Files\\Agilent\\Network Analyzer\\Documents\\default.s2p \n1725\n\nSENSe<ch>:CORRection:COLLect:SESSion<n> :VMC:MIXer:CHARacterize:CAL: OPTion \n<char> \n(Read-Write) Sets the mixer characterization method to ECal, Mechanical, or read from a file. \nParameters \n<ch> Any existing channel number. If unspecified, value is set to 1 \n<n> Session number. Choose from 1 to 16. Learn about Cal sessions. \n<char> ECAL - Electronic Calibration Module \nMECH - Mechanical Calibration Kit \nFILE, <filename> - Retrieve a mixer characterization file. Also specify the \nfilename of the S2P used for mixer characterization. Use the full path name, \nfile name, and .S2P suffix. Use the VMC:CHARacterize:CAL:FILename \ncommand to query the filename.. \nExamples SENS:CORR:COLL:SESS:VMC:MIX:CHAR:CAL:OPT ECAL \nSENS2:CORR:COLL:SESS6:VMC:MIXer:CHAR:CAL:OPTion FILE, \nMyMixerFile.mxr \nQuery Syntax SENS:CORR:COLL:SESS:VMC:MIX:CHAR:CAL:OPT? \nReturn Type String \nDefault MECH \nSENSe<ch>:CORRection:COLLect:SESSion<n> :VMC:MIXer:CHARacterize:CAL: REVerse \n<bool> \n(Read-Write) Specifies the direction in which to characterize the calibration mixer. Learn more about \nthe calibration mixer. \nParameters \n<ch> Any existing channel number. If unspecified, value is set to 1 \n<n> Session number. Choose from 1 to 16. Learn about Cal sessions. \n<bool> False (0) - Characterize the calibration mixer in the SAME direction as that \nspecified in the mixer setup. \nTrue (1) - Characterize the calibration mixer in the REVERSE direction as that \nspecified in the mixer setup. \nExamples SENS:CORR:COLL:SESS:VMC:MIX:CHAR:CAL:REV 1 \n1726\n\nQuery Syntax SENS:CORR:COLL:SESS:VMC:MIX:CHAR:CAL:REV? \nReturn Type Boolean \nDefault False \nSENSe<ch>:CORRection:COLLect:SESSion<n > :VMC:MIXer:ECAL:CHARacteriza <mod> \n,<char> \n(Read-Write) Specifies the ECal module and characterization to be used for the mixer characterization \nportion of the calibration. \nParameters \n<ch> Any existing channel number. If unspecified, value is set to 1 \n<n> Session number. Choose from 1 to 16. Learn about Cal sessions. \n<mod> 1 - Electronic Calibration Module \n<char> Characterization number in the specified ECAL module. Choose from: \n0 Factory characterization (data that was stored in the ECal module by \nAgilent). Default if not specified. \n1 User characterization #1 \n2 User characterization #2 \n3 User characterization #3 \n4 User characterization #4 \n5 User characterization #5 \nExamples SENS:CORR:COLL:SESS:VMC:MIX:ECAL:CHAR 1,0 \nQuery Syntax SENS:CORR:COLL:SESS:VMC:MIX:ECAL:CHAR? \nReturn Type Numeric \nDefault 1,0 \nSENSe<ch>:CORRection:COLLect:SESSion<n> :VMC:MIXer:ECAL:PORTmap <mod>, \n<string> \n1727\n\n(Read-Write) Sets the port mapping for the mixer characterization with ECal. This command is \nrequired if SENS:CORR:COLL:SESS:VMC:MIX:CHAR:CAL:OPT ECAL is specified. \nParameters \n<ch> Any existing channel number. If unspecified, value is set to 1 \n<n> Session number. Choose from 1 to 16. Learn about Cal sessions. \n<mod> 1 - Electronic Calibration Module \n<string> Choose from: \n\"A1\" - ECAL module port A is connected to PNA port 1 \n\"B1\" - ECAL module port B is connected to PNA port 1 \nExamples SENS:CORR:COLL:SESS:VMC:MIX:ECAL:PORT? \nSENS2:CORR:COLL:SESS:VMC:MIXer:ECAL:PORTmap 1,\"A1\" \nQuery Syntax SENS:CORR:COLL:SESS:VMC:MIX:ECAL:PORTmap? \nReturn Type String \nDefault \"A1\" \nSENSe<ch>:CORRection:COLLect:SESSion<n>:VMC:OPERation <string> \n(Read-Write) Perform either full VMC calibration or mixer characterization only. \nParameters \n<ch> Any existing channel number. If unspecified, value is set to 1 \n<n> Session number. Choose from 1 to 16. Learn about Cal sessions. \n<char> 'CAL' - full calibration and mixer characterization \n'CHAR' - mixer characterization only (no reference mixer required) - Saves \nan .S2P file with the filename specified in \nSENS<ch>:CORR:COLL:SESSion<n >:VMC:CHARacterize:CAL:FILename \n<filename> . If none is specified, a filename is automatically generated and can \nbe queried using the filename command. \nExamples SENS:CORR:COLL:SESS:VMC:OPER 'CAL' \nQuery Syntax SENS:CORR:COLL:SESS:VMC:OPER? \nReturn Type String \nDefault CAL \n1728\n\nSENSe<ch>:CORRection:COLLect:SESSion<n> :VMC:TWOPort:ECAL:CHARacteriza <mod> \n,<char> \n(Read-Write) Specifies the ECal module and characterization to be used for the VMC calibration. \nParameters \n<ch> Any existing channel number. If unspecified, value is set to 1 \n<n> Session number. Choose from 1 to 16. Learn about Cal sessions. \n<mod> 1 - Electronic Calibration Module \n<char> Characterization number in the specified ECAL module. Choose from: \n0 Factory characterization (data that was stored in the ECal module by \nAgilent). Default if not specified. \n1 User characterization #1 \n2 User characterization #2 \n3 User characterization #3 \n4 User characterization #4 \n5 User characterization #5 \nExamples SENS:CORR:COLL:SESS:VMC:TWOP:ECAL:CHAR 1,1 \nQuery Syntax SENS:CORR:COLL:SESS:VMC:TWOP:ECAL:CHAR? \nReturn Type Integer \nDefault 1,0 \nSENSe<ch>:CORRection:COLLect:SESSion<n> :VMC:TWOPort:ECAL:ORIentation[:STATe] \n<bool> \n1729\n\n(Read-Write) Sets ECAL orientation for the VMC ECal. \nParameters \n<ch> Any existing channel number. If unspecified, value is set to 1 \n<n> Session number. Choose from 1 to 16. Learn about Cal sessions. \n<bool> 1 = ON \n0 = OFF \nExamples SENS:CORR:COLL:SESS:VMC:TWOP:ECAL:ORI 1 \nQuery Syntax SENS:CORR:COLL:SESSion:VMC:TWOPort:ECAL:ORIentation[:STATe]? \nReturn Type Integer \nDefault ON \nSENSe<ch>:CORRection:COLLect:SESSion<n> :VMC:TWOPort:ECAL:PORTmap <mod>, \n<string> \n(Read-Write) Specifies the manual orientation (which ports of the module are connected to which \nports of the PNA) when orientation is turned off. \nParameters \n<ch> Any existing channel number. If unspecified, value is set to 1 \n<n> Session number. Choose from 1 to 16. Learn about Cal sessions. \n<mod> 1 - Electronic Calibration Module \n<string> Port Map, formatted in the following manner: \nAw,Bx,Cy,Dz \nwhere: \nA, B, C, and D are literal ports on the ECAL module. \nw,x,y, z are substituted for PNA port numbers to which the ECAL module port is \nconnected. \nPorts of the module which are not used are omitted from the string. \nFor example, on a 4-port ECal module with: \nport A connected to PNA port 2 \n1730\n\nport B connected to PNA port 3 \nport C not connected \nport D connected to PNA port 1 \nthe string would be: A2,B3,D1 \nIf either the receive port or source port (or load port for 2-port cal) of the \nmeasurement is not in this string and orientation is OFF, an attempt to perform \nan ECal will fail. \nExamples SENS:CORR:COLL:SESS:VMC:TWOP:ECAL:PORTmap 1,\"A2,B1\" \nQuery Syntax SENS:CORR:COLL:SESS:VMC:TWOP:ECAL:PORTmap? \nReturn Type string \nDefault \"A1,B2\" \nSENSe<ch>:CORRection:COLLect:SESSion<n> :VMC:TWOPort:METHod <string> \n(Read-Write) Specifies the guided ECal method for performing the thru portion of the calibration. \nParameters \n<ch> Any existing channel number. If unspecified, value is set to 1 \n<n> Session number. Choose from 1 to 16. Learn about Cal sessions. \n<char> 'DEFAULT' - Default \n'ADAP' - Adapter removal \n'FLUSH' - Flush Through \n'UNKN' - Unknown Thru \nExamples SENS:CORR:COLL:SESS:VMC:TWOP:METH 'ADAP' \nSENSe2:CORR:COLL:SESSion6:VMC:TWOPort:METHod 'FLUSH' \nQuery Syntax SENS:CORR:COLL:SESS:VMC:TWOP:METH? \nReturn Type String \nDefault DEFAULT \nSENSe<ch>:CORRection:COLLect:SESSion<n> :VMC:TWOPort:OMITisolat <bool> \n1731\n\n(Read-Write) Select to omit or perform the isolation portion of the ECAL. \nParameters \n<ch> Any existing channel number. If unspecified, value is set to 1 \n<n> Session number. Choose from 1 to 16. Learn about Cal sessions. \n<bool> 1 - omit isolation \n0 - perform isolation \nExamples SENS:CORR:COLL:SESS:VMC:TWOP:OMIT 1 \nQuery Syntax SENS:CORR:COLL:SESS:VMC:TWOP:OMIT? \nReturn Type Numeric \nDefault 1 \nSENSe<ch>:CORRection:COLLect:SESSion<n> :VMC:TWOPort:OPTion <string> \n(Read-Write) Sets the 2-port calibration option to ECAL or MECHanical \nParameters \n<ch> Any existing channel number. If unspecified, value is set to 1 \n<n> Session number. Choose from 1 to 16. Learn about Cal sessions. \n<char> \nChoose from: \n'ECAL' Electronic Calibration Module \n'MECH' Mechanical Calibration Kit \nExamples SENS:CORR:COLL:SESS:VMC:TWOP:OPT 'MECH' \nSENSe2:CORR:COLL:SESSion6:VMC:TWOPort:OPTion 'ECAL' \nQuery Syntax SENS:CORR:COLL:SESS:VMC:TWOP:OPT? \nReturn Type String \nDefault \"MECH\" \n1732\n\nSense:Couple Commands \nClick on a blue keyword to view the command details. \nSee Also \nExample Programs \nSynchronizing the PNA and Controller \nSCPI Command Tree \nSENSe<cnum>:COUPle <ALL | NONE> \n(Read-Write) Sets the sweep mode as Chopped or Alternate. \nLearn about Alternate Sweep \nParameters \n<cnum> Any existing channel number; if unspecified, value is set to 1. \n<ALL | NONE> ALL - Sweep mode set to Chopped - reflection and transmission measured on \nthe same sweep. \nNONE - Sweep mode set to Alternate - reflection and transmission measured \non separate sweeps. Improves Mixer bounce and Isolation measurements. \nIncreases sweep time \nExamples SENS:COUP ALL \nsense2:couple none \nQuery Syntax SENSe<cnum>:COUPle? \nReturn Type Character \nDefault ALL \nSENSe<cnum>:COUPle:PARameter[:STATe] <bool> \n1733\n\n(Read-Write) Turns ON and OFF Time Domain Trace Coupling. All of the measurements in the \nspecified channel are coupled. \nTo select Transform parameters to couple, use CALC:TRAN:COUP:PAR \nTo select Gating parameters to couple, use CALC:FILT:COUP:PAR \nLearn more about Time Domain Trace Coupling. \nParameters \n<cnum> Any existing channel number; if unspecified, value is set to 1. \n<bool> ON (or 1) - Turns ON Time Domain Trace Coupling. \nOFF (or 0) - Turns OFF Time Domain Trace Coupling. \nExamples SENS:COUP:PAR 0 \nsense2:couple:parameter:state on \nQuery Syntax SENSe<cnum>:COUPle:PARameter[:STATe]? \nReturn Type Boolean \nDefault ON (or 1) \n1734\n\nSense:FOM (Frequency Offset) Commands \nControls the frequency offset settings which cause stimulus and response frequencies to be different. \nNote: These commands supersede previous FOM commands. Although the old commands will continue to work, \nthey can NOT be mixed with these new commands. \nClick on a blue keyword to view the command details. \nSee Also \nExample Programs \nLearn about Frequency Offset \nSynchronizing the PNA and Controller \nSCPI Command Tree \nSENSe<cnum>:FOM[:STATe] <bool> \n1735\n\n(Read-Write) Turns Frequency Offset ON and OFF. Frequency offset settings are not enabled until this setting is \nON. \nSend this command (FOM ON) AFTER sending other FOM settings to avoid 'out-or-range' errors. \nParameters \n<cnum> Any existing channel number; if unspecified, value is set to 1. \n<bool> ON (or 1) - turns FOM ON. \nOFF (or 0) - turns FOM OFF. \nExamples SENS:FOM 1 \nsense2:fom:state on \nQuery Syntax SENSe<cnum>:FOM:STATe? \nReturn Type Boolean \nDefault OFF \nSENSe<cnum>:FOM:CATalog? \n(Read-only) Returns a comma-separated list of available range names in the PNA. \nParameters \n<cnum> Any existing channel number; if unspecified, value is set to 1. \nExamples SENS:FOM:CAT? \n'returns \n\"Primary, Source, Receivers\" \nReturn Type String \nDefault Not Applicable \nSENSe<cnum>:FOM:COUNt? \n1736\n\n(Read-only) Returns the number of valid ranges in the PNA. \nParameters \n<cnum> Any existing channel number; if unspecified, value is set to 1. \nExamples SENS:FOM:COUN? \nsense2:fom:count? \nQuery Syntax SENSe<cnum>:FOM:COUNt? \nReturn Type Numeric \nDefault Not Applicable \nSENSe<cnum>:FOM:DISPlay:SELect <string> \n(Read-Write) Select the range to be displayed on the PNA x-axis. All traces in the channel have this same x-axis \nscaling. \nParameters \n<cnum> Any existing channel number; if unspecified, value is set to 1. \n<string> Range name. Case insensitive. Use SENSe:FOM:CAT? to see a list of available \nfrequency range names. \nExamples SENS:FOM:DISPlay:SELect \"source2\" \nsense2:fom:display:select \"source\" \nQuery Syntax SENSe<cnum>:FOM:DISPlay:SELect? \nReturn Type String \nDefault Receivers \nSENSe<cnum>:FOM:RNUM? <string> \n1737\n\n(Read-only) Returns the number of a specified range name. \nThe FOM range items are typically numbered as follows: \nPrimary 1. \nSource 2. \nReceivers 3. \nSource2 (if present) 4. \nParameters \n<cnum> Any existing channel number; if unspecified, value is set to 1. \n<string> Range name for which a number is being queried. Case insensitive. Use \nSENSe:FOM:CAT? to see a list of available range names. \nExamples SENS:FOM:RNUM? \"receivers\" \nsense2:fom:rnum? \"Source2\" \nReturn Type Numeric \nDefault Not Applicable \nSENSe<cnum>:FOM:RANGe<n>:COUPled <bool> \n(Read-Write) Sets and returns the state of coupling (ON or OFF) of the specified range to the primary range. \nParameters \n<cnum> Any existing channel number; if unspecified, value is set to 1. \n<n> Range number to couple to primary range. An error is returned when attempting to \ncouple to the Primary range (1). \n<bool> ON (or 1) - Couple range to primary range. \nOFF (or 0) - Do NOT couple to primary range. \nExamples SENS:FOM:RANG:COUP 1 \nsense2:fom:range2:coupled 0 \nQuery Syntax SENSe<cnum>:FOM:RANGe<n>:COUPled? \nReturn Type Boolean \nDefault ON (or 1) Coupled \n1738\n\nSENSe<cnum>:FOM:RANGe<n>:FREQuency:CW <num> \n(Read-Write) Sets and returns the CW frequency. \nThis setting is valid for the primary range, or if the specified range is already uncoupled from the primary range \nand if the sweep type is CW. \nParameters \n<cnum> Any existing channel number; if unspecified, value is set to 1. \n<n> Range number. If unspecified, value is set to 1. \n<num> CW frequency value in Hz. Choose any frequency within the range of the PNA. \nExamples SENS:FOM:RANG:FREQ:CW 1e9 \nsense2:fom:range2:frequency:cw 10000000 \nQuery Syntax SENSe<cnum>:FOM:RANGe:<n>:FREQuency:CW? \nReturn Type Numeric \nDefault Center frequency of the PNA. \nSENSe<cnum>:FOM:RANGe<n>:FREQuency:DIVisor <num> \n(Read-Write) Sets and returns the divisor value. \nThis setting is valid only if the specified range is coupled to the primary range. \nParameters \n<cnum> Any existing channel number; if unspecified, value is set to 1. \n<n> Range number. If unspecified, value is set to 1. \n<num> Divisor value (unitless). \nExamples SENS:FOM:RANG:FREQ:DIV 3 \nsense2:fom:range2:frequency:divisor 0 \nQuery Syntax SENSe<cnum>:FOM:RANGe<n>:FREQuency:DIVisor? \nReturn Type Numeric \nDefault 1 \n1739\n\nSENSe<cnum>:FOM:RANGe<n>:FREQuency:MULTiplier <num> \n(Read-Write) Sets and returns the multiplier value to be used when coupling this range to the primary range. \nThis setting is valid only if the specified range is coupled to the primary range. \nParameters \n<cnum> Any existing channel number; if unspecified, value is set to 1. \n<n> Range number. If unspecified, value is set to 1. \n<num> Multiplier value. (Unitless) \nExamples SENS:FOM:RANG:FREQ:MULT 1 \nsense2:fom:range2:frequency:multiplier 2 \nQuery Syntax SENSe<cnum>:FOM:RANGe<n>:FREQuency:MULTplier? \nReturn Type Numeric \nDefault 1 \nSENSe<cnum>:FOM:RANGe<n>:FREQuency:OFFSet <num> \n(Read-Write) Sets and returns the offset value to be used when coupling this range to the primary range. Learn \nmore about offset value. \nThis setting is valid only if the specified range is coupled to the primary range. \nParameters \n<cnum> Any existing channel number; if unspecified, value is set to 1. \n<n> Range number. If unspecified, value is set to 1. \n<num> Offset value. (Unitless) \nExamples SENS:FOM:RANG:FREQ:OFFS 1E9 \nsense2:fom:range2:frequency:offset 10000000 \nQuery Syntax SENSe<cnum>:FOM:RANGe<n>:FREQuency:OFFSet? \nReturn Type Numeric \nDefault 0 \nSENSe<cnum>:FOM:RANGe<n>:FREQuency:STARt <num> \n1740\n\n(Read-Write) Sets and returns the Start value of frequency range. Also specify Stop frequency. \nThis setting is valid for the primary range, or if the specified range is already uncoupled from the primary range \nand if the sweep type is LOG or LINear. \nParameters \n<cnum> Any existing channel number; if unspecified, value is set to 1. \n<n> Range number. If unspecified, value is set to 1. \n<num> Start value in Hz. Choose any frequency within the range of the PNA. \nExamples SENS:FOM:RANG:FREQ:STAR 1GHz \nsense2:fom:range2:frequency:start 100000000 \nQuery Syntax SENSe<cnum>:FOM:RANGe<n>:FREQuency:STARt? \nReturn Type Numeric \nDefault Minimum frequency of the PNA. \nSENSe<cnum>:FOM:RANGe<n>:FREQuency:STOP <num> \n(Read-Write) Sets and returns the Stop value of frequency range. Also specify Start frequency. \nThis setting is valid for the primary range, or if the specified range is already uncoupled from the primary range \nand if the sweep type is LOG or LINear. \nParameters \n<cnum> Any existing channel number; if unspecified, value is set to 1. \n<n> Range number. If unspecified, value is set to 1. \n<num> Stop value in Hz. Choose any frequency within the range of the PNA. \nExamples SENS:FOM:RANG:FREQ:STOP 1e12 \nsense2:fom:range2:frequency:stop 10000000000 \nQuery Syntax SENSe<cnum>:FOM:RANGe<n>:FREQuency:STOP? \nReturn Type Numeric \nDefault Maximum frequency of the PNA. \nSENSe<cnum>:FOM:RANGe<n>:NAME? \n1741\n\n(Read-only) Returns the name of range<n>. \nThe FOM range items are typically named as follows: \nPrimary 1. \nSource 2. \nReceivers 3. \nSource2 (if present) 4. \nParameters \n<cnum> Any existing channel number; if unspecified, value is set to 1. \n<n> Range number. If unspecified, value is set to 1. \nExamples SENS:FOM:RANG:NAME? \nsense2:fom:range2:name? \nReturn Type String \nDefault Not Applicable \nSENSe<cnum>:FOM:RANGe<n>:SWEep:TYPE <char> \n(Read-Write) Sets and returns the sweep type to be used with the specified range. \nThis setting is valid only if the specified range is already uncoupled from the primary range. \nLearn about Unsupported Sweep Type combinations. \nParameters \n<cnum> Any existing channel number; if unspecified, value is set to 1. \n<n> Range number. If unspecified, value is set to 1. \n<char> Sweep type. Choose from: \nCW - Also specify CW frequency. \nLINear - Also specify frequency Start/Stop or Center/Span \nLOG - Also specify frequency Start/Stop or Center/Span \nPOWer - Also specify power Start/Stop or Center/Span \nSEGMent - Also specify segment sweep settings. \n1742\n\nExamples SENS:FOM:RANG:SWE:TYPE LOG \nsense2:fom:range2:sweep:type linear: \nQuery Syntax SENSe<cnum>:FOM:RANGe<n>:SWEep:TYPE? \nReturn Type Character \nDefault Linear \nLast Modified: \n8-Mar-2007 MQX New topic \n1743\n\nSense:Frequency Commands \nSets the frequency sweep functions of the analyzer. \nClick on a blue keyword to view the command details. \nSee Also \nExample using some of these commands. \nLearn about Frequency Sweep \nSynchronizing the PNA and Controller \nSCPI Command Tree \nNote: All of the commands in this block will accept MIN or MAX instead of a numeric parameter. \nAlso, kHZ, MHz, and GHz are accepted as suffixes/units. \nSee SCPI Syntax for more information. \nSENSe<cnum>:FREQuency:CENTer <num> \n(Read-Write) Sets the center frequency of the analyzer. \nParameters \n<cnum> Any existing channel number. If unspecified, value is set to 1 \n<num> Center frequency. Choose any number between the minimum and maximum \nfrequency limits of the analyzer. Units are Hz. \nSee Note \nExamples SENS:FREQ:CENT 1000000 \nsense2:frequency:center 1mhz \nsense2:frequency:center 1e6 \nQuery Syntax SENSe<cnum>:FREQuency:CENTer? \nReturn Type Numeric \nDefault Center of the analyzer's frequency span \n1744\n\nSENSe<cnum>:FREQuency[:CW |:FIXed] <num> \n(Read-Write) Sets the Continuous Wave (or Fixed) frequency. Must also send SENS:SWEEP:TYPE \nCW to put the analyzer into CW sweep mode. \nParameters \n<cnum> Any existing channel number. If unspecified, value is set to 1 \n<num> CW frequency. Choose any number between the minimum and maximum \nfrequency limits of the analyzer. Units are Hz. \nSee Note \nExamples SENS:FREQ 1000000 \nSENS:FREQ:CW MIN \nsense2:frequency:fixed 1mhz \nQuery Syntax SENSe<cnum>:FREQuency[:CW | :FIXed]? \nReturn Type Numeric \nDefault 1 GHz \nSENSe<cnum>:FREQuency:SPAN <num> \n(Read-Write) Sets the frequency span of the analyzer. \nParameters \n<cnum> Any existing channel number. If unspecified, value is set to 1 \n<num> Frequency span. Choose any number between: \n0 (minimum) and the maximum frequency span of the analyzer. \nUnits are Hz \nSee Note \nExamples SENS:FREQ:SPAN 1000000 \nsense2:frequency:span max \nQuery Syntax SENSe<cnum>:FREQuency:SPAN? \nReturn Type Numeric \nDefault Maximum frequency span of the analyzer \nSENSe<cnum>:FREQuency:STARt <num> \n1745\n\n(Read-Write) Sets the start frequency of the analyzer. \nParameters \n<cnum> Any existing channel number. If unspecified, value is set to 1 \n<num> Start frequency. Choose any number between the MIN and MAX frequency \nlimits of the analyzer. Units are Hz \nIf FREQ:START is set greater than FREQ:STOP, then STOP is set equal to \nSTART. \nSee Note \nExamples SENS:FREQ:STAR 1000000 \nsense2:frequency:start MIN \nQuery Syntax SENSe<cnum>:FREQuency:STARt? \nIf Sweep type is segment, this query returns the start frequency of the first \nsegment. \nReturn Type Numeric \nDefault Minimum frequency of the analyzer \nSENSe<cnum>:FREQuency:STOP <num> \n(Read-Write) Sets the stop frequency of the analyzer. \nParameters \n<cnum> Any existing channel number. If unspecified, value is set to 1 \n<num> Stop frequency. Choose any number between: \nthe minimum and maximum frequency limits of the analyzer. Units are Hz \nIf FREQ:STOP is set less than FREQ:START, then START will be set equal to \nSTOP. \nSee Note \nExamples SENS:FREQ:STOP 1000000 \nsense2:frequency:stop max \nQuery Syntax SENSe<cnum>:FREQuency:STOP? \nIf Sweep type is segment, this query returns the stop frequency of the last segment. \nReturn Type Numeric \nDefault Maximum frequency of the analyzer \n1746\n\n1747\n\nSense:IF Commands \nControls the IF source and gain settings for use with the E836x H11 Option. \nSee IF/DSP and Pulse commands for the PNA-X. \nClick on a blue keyword to view the command details. \nSee IF Access User Interface Settings \nSynchronizing the PNA and Controller \nSCPI Command Tree \nSENSe<cnum>:IF:FILTer:SAMPle:COUNt <num> \n(Read-Write) Sets and returns the number of taps in the IF filter. The IF filter sample count setting is \nonly used when SENSe:IF:FILTer:SAMPle:COUNt:MODE is set to MANUAL. Critical Note: \nParameters \n<cnum> Existing channel number to manipulate. If unspecified, <cnum> is set to 1. \n<num> An integer value. (MIN and MAX return the minimum and maximum allowed values, \nrespectively.) \nExamples SENS:IF:FILT:SAMP:COUN 40 \nsense2:if:filter:sample:count maximum \nQuery Syntax SENS:IF:FILTer:SAMPle:COUNt? \nReturn Type Numeric \nDefault Instrument dependent. \nSENSe<cnum>:IF:FILTer:SAMPle:COUNt:MODE <char> \n1748\n\n(Read-Write) Sets and returns the IF filter sample count mode to the specified value. When in \nMANUAL mode, the value specified for the IF Filter sample count is used as the number of taps in the \nIF filter. Critical Note: \nParameters \n<cnum> Existing channel number to manipulate. If unspecified, <cnum> is set to 1. \n<char> Choose either AUTO or MANUAL. \nExamples SENS:IF:FILT:SAMP:COUN:MODE MANUAL \nsense2:if:filter:sample:count:mode AUTO \nQuery Syntax SENS:IF:FILTer:SAMPle:COUNt:MODE? \nReturn Type Character \nDefault AUTO \nSENSe<cnum>:IF:FILTer:SAMPle:PERiod <num> \n(Read-Write) Sets and returns the IF filter sample period. The IF filter sample period setting is only \nused by the instrument when the SENS:IF:FILT:SAMP:PER:MODE is set to MANUAL. Critical \nNote: \nParameters \n<cnum> Existing channel number to manipulate. If unspecified, <cnum> is set to 1. \n<num> Sample period. Choose from values returned from the \nSENS:IF:FILTer:SAMPle:PERiod:CAT? command. \nExamples SENS:IF:FILT:SAMP:PER 6 us \nsense2:if:filter:sample:period maximum \nQuery Syntax SENS:IF:FILTer:SAMPle:PERiod? \nReturn Type Numeric \nDefault Instrument dependent. \nSENSe<cnum>:IF:FILTer:SAMPle:PERiod:CATalog? \n(Read-Only) Returns the list of allowed IF filter sample periods for this instrument. Critical Note: \nParameters \n<cnum> Existing channel number to manipulate. If unspecified, <cnum> is set to 1. \nExamples SENS:IF:FILT:SAMP:PER:CAT? \nsense2:if:filter:sample:period:catalog? \nQuery Syntax SENS:IF:FILTer:SAMPle:PERiod:CATalog? \nReturn Type String \nDefault AUTO \n1749\n\nSENSe<cnum>:IF:FILTer:SAMPle:PERiod:MODE <char> \n(Read-Write) Sets and returns the IF filter sample period mode to the specified value. Critical Note: \nParameters \n<cnum> Existing channel number to manipulate. If unspecified, <cnum> is set to 1. \n<char> Sample period mode. Choose from AUTO or MANUAL. \nExamples SENS:IF:FILT:SAMP:PER:MODE MANUAL \nsense2:if:filter:sample:period:mode AUTO \nQuery Syntax SENS:IF:FILTer:SAMPle:PERiod:MODE? \nReturn Type Character \nDefault AUTO \nSENSe<cnum>:IF:GAIN:ALL[:STATe] <char> \n(Write only) Sets the gain state for ALL receivers to Auto or Manual. \nParameters \n<cnum> Existing channel number to manipulate. If unspecified, <cnum> is set to 1. \n<char> Choose from AUTO or MANUAL \nExamples SENS:IF:GAIN:ALL AUTO \nsense:if:gain:all:state manual \nQuery Syntax Not Applicable \nReturn Type Character \nDefault AUTO \nSENSe<cnum>:IF:GAIN:LEVel <id>, <level> \n1750\n\n(Read Write) Manually sets the gain level for the specified receiver. \nParameters \n<cnum> Existing channel number to manipulate. If unspecified, <cnum> is set to 1. \n<id> Choose from: 'A', 'B', 'R1', 'R2'. \nNote: The A and R1 receivers are always switched together. B and R2 are also \nalways switched together. For example, if you specify 'A', R1 will also be \nswitched. \n<level> Gain level. Choose from: \n0 - Lowest gain setting \n1\n2 - Highest gain setting \nExamples SENS:IF:GAIN:LEVel 'A', 1 \nQuery Syntax SENSe<cnum>:IF:GAIN:LEVel? <id> \nReturn Type Numeric \nDefault 0 \nSENSe<cnum>:IF:GAIN[:STATe]?, <id> \n(Read only) Returns the gain state for the specified receiver. Use SENS:IF:GAIN:ALL. to set the gain \nstate for all channels. \nParameters \n<cnum> Existing channel number to manipulate. If unspecified, <cnum> is set to 1. \n<id> Choose from: 'A', 'B', 'R1', 'R2'. \nNote: The A and R1 receivers are always switched together. B and R2 are also \nalways switched together. For example, if you specify 'A', R1 will also be \nswitched. \nExamples SENS:IF:GAIN? 'A' \nReturn Type Boolean \nDefault Not Applicable \n1751\n\nSENSe<cnum>:IF:GATE:STATe <boolean> \n(Read-Write) Sets or returns the IF filter gate state. \nParameters \n<cnum> Existing channel number to manipulate. If unspecified, <cnum> is set to 1. \n<boolean> Choose from ON or OFF \nExamples SENS:IF:FILT:GATE:STAT ON \nsense2:if:filter:gate:state 0 \nQuery Syntax SENS:IF:FILTer:SAMPle:COUNt:MODE? \nReturn Type Boolean \nDefault AUTO \nSENSe<cnum>:IF:SOURce:PATH <id>, <char> \n(Read Write) Sets the source path for the specified receiver. An error is returned if <id> is not valid, \nor if <char> is not valid for the specified <id>. \nParameters \n<cnum> Existing channel number to manipulate. If unspecified, <cnum> is set to 1. \n<id> Choose from: 'A', 'B', 'R1', 'R2' \nNote: The A and R1 receivers are always switched together. B and R2 are also \nalways switched together. For example, if you specify \"A\", R1 will also be \nswitched. \n<char> Choose from: \nNORMal - the PNA decides the appropriate IF input paths. \nEXTernal - always use the rear panel IF inputs. \nExamples SENS:IF:SOUR:PATH 'A', Ext \nQuery Syntax SENSe<cnum>:IF:SOURce:PATH? <id> \nReturn Type Character \nDefault Normal \n1752\n\nSense:IF Commands \nControls the IF filter for use with the PNA X. \nClick on a blue keyword to view the command details. \nSynchronizing the PNA and Controller \nSCPI Command Tree \nPNA-X DSP Block diagram \nAll of the Sense:IF commands, except the frequency commands, make settings related to the DSP section of the IF Path. \nSee the entire IF Path Configuration. \nNote: For any of the Filter \"Stage\" parameters to take effect, SENS:IF:FILT:AUTO must be set to OFF \n(MANUAL) and mode, and SENS:IF:FILT:CMOD must be set to OFF. \n1753\n\nCritical Note: These commands act on the selected measurement. You can select one measurement for \neach channel using Calc:Par:Select \nSENSe<cnum>:IF:FILTer:AUTO <bool> \n(Read-Write) Sets and returns whether the PNA configures the 3-stage digital filter settings or they \nwill be configured manually. When making manual settings, also send SENS:IF:FILT:CMOD OFF \nwhich routes the IF through the 3-stage filter. \nCritical Note \nParameters \n<cnum> Existing channel number. If unspecified, <cnum> is set to 1. \n<bool> (Boolean) \nON (or 1) - Automatic: PNA controls digital filter settings. \nOFF (or 0) - Manual: You control digital filter settings using other Sens:IF \ncommands. \nExamples SENS:IF:FILT:AUTO 1 \nsense2:if:filter:auto 0 \nQuery Syntax SENSe<cnum>:IF:FILTer:AUTO? \nReturn Type Boolean \nDefault ON \nSENSe:IF:FILTer:CMODe <bool> \n(Read-Write) Sets and returns the ADC capture mode modeled as a 2-pole switch in the above \ndiagram. The switch either bypasses or routes the IF through the 3-stage digital filter. \nCritical Note \nParameters \n<bool> (Boolean) \nON (or 1) - The digital filters are bypassed and the raw ADC readings are taken \ndirectly. A maximum of 4096 data points per sweep can be acquired. \nOFF (or 0) - The digital filters are used to process IF information. The filters \ncan be configured automatically or manually using SENS:IF:FILT:AUTO. \nExamples SENS:IF:FILT:CMOD 1 \nsense2:if:filter:cmode 0 \nQuery Syntax SENSe<cnum>:IF:FILTer:CMODe? \n1754\n\nReturn Type Boolean \nDefault OFF \nSENSe<cnum>:IF:FILTer:ERRors? \n(Read-only) Returns the error string associated with the digital filters. The return string has three fields \nseparated by commas: \"stage1 status, stage2 status, stage3 status\" \nEach of these fields can contain one or more of the following error codes: \nNO ERROR \n*NUMBER-OF-COEFFICIENTS - the number of coefficients is excessive for that filter-stage \n*COEFFICIENT VALUE - one or more coefficients are out of range for that filter-stage \n*SUM-OF-COEFFICIENTS - the sum of all coefficients is excessive for that filter-stage, \n*FREQUENCY - the frequency for Stage 1 is out of range (only applies stage1 field), \n*PARAMETER - one or more parameters are out of range (only applies to stage 3 field) \nCritical Note \nParameters \n<cnum> Existing channel number. If unspecified, <cnum> is set to 1. \nExamples SENS:IF:FILT:ERR? \n'example return strings\" \nNO ERROR, NO ERROR, NO ERROR \nindicates no errors, \n*SUM-OF-COEFFICIENTS, NO ERROR, NO ERROR \nindicates that the sum of all filter coefficients exceed the \nmaximum value for the Stage-1 filter, \n*COEFFICIENT *SUM-OF-COEFFICIENTS, NO ERROR, *PARAMETER \nindicates a problems with Stage 1 coefficients and a problem with \none or more of the parameters associated with the Stage 3 filter. \nReturn Type String \nDefault Not Applicable \nSENSe<cnum>:IF:FILTer:STAGE<n>:COEFficients <coef> \n1755\n\n(Read-Write) Sets and returns the digital filter coefficients of the specified stage. \nCritical Note \nParameters \n<cnum> Existing channel number. If unspecified, <cnum> is set to 1. \n<n> Stage number. Choose 1 or 2 \n<coef> An array of real numbers. Filter coefficients \nExamples SENS:IF:FILT:STAG2:COEF 0,0.1,0.7,0.7,0.1 \nsense2:if:filter:stage1:coefficients \nQuery Syntax SENSe<cnum>:IF:FILTer:STAGE<n>:COEFficients? \nExample SENS:IF:FILT:STAG2:COEF? \nsense2:if:filter:stage1:coefficients? \nReturn Type Numeric \nDefault Stage dependent \nSENSe<cnum>:IF:FILTer:STAGE<n>:COUNt? [char] \n(Read-only) Returns the number of taps in the digital filter of the specified stage. The filter sample \ncount setting is only used when SENSe:IF:FILTer:AUTO is set to False (MANUAL). \nCritical Note \nParameters \n<cnum> Existing channel number. If unspecified, <cnum> is set to 1. \n<n> Stage number. Choose 1 or 2 \n[char] Optional parameter. Choose from: \nnot specified - returns the current number of coefficients for the specified \nstage. \nMIN - returns the minimum number of coefficients for the specified \nstage. Stage1: 10, Stage2: 1 \nMAX - returns the maximum number of coefficients for the specified \nstage. Stage1 & 2: 1024 \nExamples SENS:IF:FILT:STAG2:COUN? \nsense2:if:filter:stage1:count? max \nReturn Type Numeric \nDefault Stage dependent \n1756\n\nSENSe<cnum>:IF:FILTer:STAGE1:FREQuency <value> \n(Read-Write) Sets and returns the Numerically Controlled Oscillator (NCO) frequency. This command \nis only used when SENSe:IF:FILTer:AUTO is set to False (Manual). \nCritical Note \nParameters \n<cnum> Existing channel number. If unspecified, <cnum> is set to 1. \n<value> Stage 1 Frequency. Min value= 0 Hz, Max value= 15 MHz. Or \nprogrammatically use the Max and Min queries to determine the range of \nsettable values. \nExamples SENS:IF:FILT:STAGe1:FREQ 9e6 \nsense2:if:filter:stage1:frequency 9.2e6 \nQuery Syntax SENSe<cnum>:IF:FILTer:STAGE1:FREQuency? \n'returns the current parameter value \nSENSe<cnum>:IF:FILTer:STAGE1:FREQuency? Min \n'returns the minimum frequency value. \nSENSe<cnum>:IF:FILTer:STAGE1:FREQuency? Max \n'returns the maximum frequency value. \nReturn Type Numeric \nDefault 9 MHz \nSENSe<cnum>:IF:FILTer:STAGE3:CATalog? \n(Read-only) Returns a list of strings for the currently supported filter types that can be used for the \nstage 3 filter. This command is only used when SENSe:IF:FILTer:AUTO is set to False (Manual). See \nSENS:IF:FILT:STAGe3:TYPE for a list of currently supported filter types. \nCritical Note \nParameters \n<cnum> Existing channel number. If unspecified, <cnum> is set to 1. \nExamples SENS:IF:FILT:STAGe3:CAT? \nsense2:if:filter:stage3:catalog? \nReturn Type String array \nDefault Not Applicable \n1757\n\nSENSe<cnum>:IF:FILTer:STAGe3:TYPE <value> \n(Read-Write) Sets and returns the Stage 3 filter type. This command is only used when \nSENSe:IF:FILTer:AUTO is set to False (Manual). \nCritical Note \nParameters \n<cnum> Existing channel number. If unspecified, <cnum> is set to 1. \n<value> (String) Filter type. Chose from: \n\"RECT\" Rectangular Window Filter \n\"TUKEY\" Tukey Filter \n\"PWIN\" Pulse Window Filter \nExamples SENS:IF:FILT:STAGe3:TYPE RECT \nsense2:if:filter:stage3:type pwin \nQuery Syntax SENSe<cnum>:IF:FILTer:STAGE3:TYPE? \nReturn Type String \nDefault \"TUKEY\" \nSENSe<cnum>:IF:FILTer:STAGe3:PARameter <p>, <value> \n(Read-Write) Sets and returns the Stage 3 filter parameters. \nMust first select the filter type (SENS:IF:FILT:STAGe3:TYPE) before setting these parameters \nUse SENSe:IF:FILT:STAGE3:PCAT? to return a list of the available parameters for the currently \nselected filter type. \nCritical Note \nParameters \n<cnum> Existing channel number. If unspecified, <cnum> is set to 1. \n<p> (String) Filter parameter. Choose from: \n\"C\" - Tap count (Tukey, RECT, PWIN) \n\"P\" - Period (PWIN ONLY) \n\"D\" - Delay (PWIN ONLY) \n\"W\" - Width (PWIN ONLY) \n\"R\" - Ramp Count (PWIN ONLY) \n1758\n\n<value> (String) Parameter Value for the specified stage 3 parameter. Use the query form \nto return the minimum and maximum values for the specified parameter. \nExamples SENS:IF:FILT:STAGe3:PAR \"C\",64 \nsense2:if:filter:stage3:parameter \"d\",0.5E-6 \nQuery Syntax SENSe<cnum>:IF:FILTer:STAGE3:PARameter? <p> \nreturns the current parameter value \nSENSe<cnum>:IF:FILTer:STAGE3:PARameter? <p>,Min \nreturns the minimum parameter value. \nSENSe<cnum>:IF:FILTer:STAGE3:PARameter? <p>,Max \nreturns the maximum parameter value. \nExamples SENS:IF:FILT:STAGe3:PAR? \"C\" \nsense2:if:filter:stage3:parameter? \"d\",min \nReturn Type Numeric \nDefault RECT: C = 1 \nPWIN: C=1E6, P=10ms, D=50us, W=50us, R=7 \nTUKEY: C=1 \nSENSe<cnum>:IF:FILTer:STAGE3:PCATalog? \n(Read-only) Returns a list of the available parameters for the currently selected filter type. \nCritical Note \nParameters \n<cnum> Existing channel number. If unspecified, <cnum> is set to 1. \nExamples SENS:IF:FILT:STAGe3:PCAT? \nsense2:if:filter:stage3:pcatalog? \nReturn Type String \nDefault Not Applicable \nSENSe<cnum>:IF:FREQuency:AUTO <bool> \n1759\n\n(Read-Write) Sets and returns the method for specifying the way the IF Frequency is determined. \nCritical Note \nParameters \n<cnum> Existing channel number. If unspecified, <cnum> is set to 1. \n<bool> (Boolean) \nON (or 1) - Automatic. PNA determines the setting for the IF frequency. \nOFF (or 0) - Manual. Use SENS:IF:FREQ to set the frequency. \nExamples SENS:IF:FREQ:AUTO 1 \nsense2:if:frequency:auto 0 \nQuery Syntax SENSe<cnum>:IF:FREQuency:AUTO? \nReturn Type Boolean \nDefault ON \nSENSe<cnum>:IF:FREQuency[:VALue] <value> \n(Read-Write) Sets and returns the IF frequency for ALL receiver paths being used for the specified \nchannel. To set this frequency, SENS:IF:FREQ:AUTO must be set to OFF (Manual). \nAlso returns the maximum and minimum allowable frequency settings. \nCritical Note \nParameters \n<cnum> Existing channel number. If unspecified, <cnum> is set to 1. \n<value> (Numeric) Frequency value. \nExamples SENS:IF:FREQ \nsense2:if:frequency \nQuery Syntax SENSe<cnum>:IF:FREQuency? \n'returns the current frequency setting \nSENSe<cnum>:IF:FREQuency? Max \n'returns the maximum allowable frequency setting \nSENSe<cnum>:IF:FREQuency? Min \n'returns the minimum allowable frequency setting \nReturn Type Numeric \nDefault 9 MHz \n1760\n\nLast Modified: \n18-Jan-2007 MX New topic \n1761\n\nSense:Mixer Commands \nPerforms Mixer setup and configuration. \nClick on a blue keyword to view the command details. \nSee Also \nExample Programs \nLearn about the Frequency Converter Application \nSynchronizing the PNA and Controller \nSCPI Command Tree \nSENSe<ch>:MIXer:APPLy \n(Write only) Applies the mixer setup settings and turns the channel ON. (Performs the same function \nas the Apply button on the mixer setup dialog box). \nParameters \n<ch> Any existing channel number. If unspecified, value is set to 1 \nExamples SENS:MIX:APPL \nQuery Syntax Not Applicable \nDefault Not Applicable \n1762\n\nSENSe<ch>:MIXer:AVOidspurs <bool> \n(Read Write) Sets and returns the state of the avoid spurs feature. Learn more about avoid spurs. \nParameters \n<ch> Any existing channel number. If unspecified, value is set to 1 \n<bool> Avoid spurs state. Choose from \n0 - Avoid spurs OFF \n1 - Avoid spurs ON \nExamples SENS:MIX:AVO \nsense2:mixer:avoidspurs 1 \nQuery Syntax SENSe<ch>:MIXer:AVOidspurs? \nReturn Type Boolean \nDefault 0 (OFF) \nSENSe<ch>:MIXer:CALCulate <char> \n(Write only) Calculates the Input, IF, or Output frequencies of the mixer setup and updates the \nchannel settings. \nParameters \n<ch> Any existing channel number. If unspecified, value is set to 1 \n<char> Mixer port to be calculated. Choose from: \n1763\n\n<char> 1st or only stage \nrequires: \nIn addition, 2nd stage \nrequires: \nINPUT \nOutput Start and Stop \nfrequencies \nLO frequency \nOutput sideband (High or \nLow) \nIF Start and Stop \nfrequencies \n2nd LO frequency \nIF sideband (High or Low) \nBoth NA \nIF Start and Stop \nfrequencies \nBoth LO frequencies \nOUTPUT \nInput Start and Stop \nfrequencies \nLO frequency \nOutput sideband (High or \nLow) \nIF Start and Stop \nfrequencies \n2nd LO frequency \nIF sideband (High or Low) \nLO_1 \nInput Start and Stop \nfrequencies \nOutput frequency \nOutput sideband (High or \nLow) \nIF Start and Stop \nfrequencies \n2nd LO frequency \nIF sideband (High or Low) \nLO_2 NA Input Start and stop \nfrequencies \n1st LO start and stop \nfrequencies \nOutput frequency \nIF sideband(High or Low \nOutput sideband(High or \nLow) \nExamples SENS:MIX:CALC Output \nQuery Syntax Not Applicable \nDefault Not Applicable \nSENSe<ch>:MIXer:LOAD <name> \n1764\n\n(Write-only) Loads a previously-configured mixer attributes file (.mxr) \nParameters \n<ch> Any existing channel number. If unspecified, value is set to 1. \n<name> Path and file name (including .mxr extension) to load. \nExamples SENSe:MIXer:LOAD \"C:\\Program Files\\Agilent\\Network \nAnalyzer\\Documents\\Mixer\\MyMixer.mxr\" \nDefault Not Applicable \nSENSe<ch>:MIXer:SAVE <name> \n(Write-only) Saves the settings for the mixer/converter test setup to a mixer attributes file. \nParameters \n<ch> Any existing channel number. If unspecified, value is set to 1. \n<name> Path and file name (including .mxr extension) to save. \nExamples SENSe:MIXer:SAVE \"C:\\Program Files\\Agilent\\Network \nAnalyzer\\Documents\\Mixer\\MyMixer.mxr\" \nDefault Not Applicable \nSENSe<ch>:MIXer:STAGe <n> \n(Read-Write) Number of IF stages of the mixer. \nParameters \n<ch> Any existing channel number. If unspecified, value is set to 1. \n<n> Number of stages. Choose either 1 or 2 \nExamples SENSe:MIX:STAG 2 \nSENSe:MIXer:STAGE 1 \nQuery Syntax SENSe<ch>:MIXer:STAGe? \nReturn Type Numeric \nDefault 1 \nSENSe<ch>:MIXer:IF:FREQuency:DENominator <num> \n1765\n\n(Read-Write) Sets or returns the denominator value of the IF Fractional Multiplier. \nParameters \n<ch> Any existing channel number. If unspecified, value is set to 1. \n<num> Denominator value. \nExamples SENSe:MIX:IF:FREQ:DEN 5 \nSENSe2:MIXer:IF:FREQ:DENominator 4 \nQuery Syntax SENSe<ch>:MIXer:IF:FREQuency:DENominator? \nReturn Type Numeric \nDefault Not Applicable \nSENSe<ch>:MIXer:IF:FREQuency:FIXed <num> \n(Read-Write) Sets or returns the fixed frequency of the IF.. \nParameters \n<ch> Any existing channel number. If unspecified, value is set to 1. \n<num> Frequency. \nExamples SENSe:MIXer:IF:FREQ:FIXed 1e9 \nSENSe2:MIXer:IF:FREQ:FIXed 1000000000 \nQuery Syntax SENSe<ch>:MIXer:IF:FREQuency:FIXed? \nReturn Type Numeric \nDefault Not Applicable \nSENSe<ch>:MIXer:IF:FREQuency:NUMerator <num> \n(Read-Write) Sets or returns the numerator value of the IF Fractional Multiplier. \nParameters \n<ch> Any existing channel number. If unspecified, value is set to 1. \n<num> Numerator value of the IF fractional multiplier \nExamples SENSe:MIX:IF:FREQ:NUM 4 \nSENSe2:MIXer:IF2:FREQ:NUMerator 3 \nQuery Syntax SENSe<ch>:MIXer:IF:FREQuency:NUMerator? \nReturn Type Numeric \nDefault Not Applicable \n1766\n\nSENSe<ch>:MIXer:IF:FREQuency:SIDeband <char> \n(Read-Write) Sets or returns the value of the IF sideband. \nParameters \n<ch> Any existing channel number. If unspecified, value is set to 1. \n<char> Sideband value. Choose from \nLOW - Low or Difference (-) \nHIGH - High or Sum (+) \nExamples SENS:MIX:IF:FREQ:SIDE LOW \nSENSe2:MIXer:IF:FREQ:SIDEband HIGH \nQuery Syntax SENSe<ch>:MIXer:IF:FREQuency:SIDeband? \nReturn Type Character \nDefault LOW \nSENSe<ch>:MIXer:IF:FREQuency:STARt <num> \n(Read-Write) Sets or returns the IF start frequency value of the mixer. \nParameters \n<ch> Any existing channel number. If unspecified, value is set to 1. \n<num> IF Start Frequency value \nExamples SENS:MIX:IF:FREQ:STAR 1e9 \nSENSe2:MIXer:IF:FREQ:STARt 1000000000 \nQuery Syntax SENSe<ch>:MIXer:IF:FREQuency:STARt? \nReturn Type Numeric \nDefault Not Applicable \nSENSe<ch>:MIXer:IF:FREQuency:STOP <num>\n1767\n\n(Read-Write) Sets or returns the stop frequency value of the mixer IF frequency. \nParameters \n<ch> Any existing channel number. If unspecified, value is set to 1. \n<num> IF Stop Frequency value \nExamples SENS:MIX:IF:FREQ:STOP 2e9 \nSENSe2:MIXer:IF:FREQ:STOP 2000000000 \nQuery Syntax SENSe<ch>:MIXer:IF:FREQuency:STOP? \nReturn Type Numeric \nDefault Not Applicable \nSENSe<ch>:MIXer:INPut:FREQuency:DENominator <value> \n(Read-Write) Sets or returns the denominator value of the Input Fractional Multiplier. \nParameters \n<ch> Any existing channel number. If unspecified, value is set to 1. \n<value> Input denominator value. \nExamples SENS:MIX:INP:FREQ:DEN 5 \nSENS2:MIXer:INPut:FREQ:DENominator 4 \nQuery Syntax SENSe<ch>:MIXer:INPut:FREQuency:DENominator? \nReturn Type Numeric \nDefault Not Applicable \nSENSe<ch>:MIXer:INPut:FREQuency:FIXed<value> \n(Read-Write) Sets or returns the fixed frequency of the input. \nParameters \n<ch> Any existing channel number. If unspecified, value is set to 1. \n<value> Input frequency. \nExamples SENSe:MIXer:INPut:FREQ:FIXed 1e9 \nSENSe2:MIXer:INPut:FREQ:FIXed 1000000000 \nQuery Syntax SENSe<ch>:MIXer:INPut:FREQuency:FIXed? \nReturn Type Numeric \nDefault Not Applicable \n1768\n\nSENSe<ch>:MIXer:INPut:FREQuency:MODE <char> \n(Read-Write) Sets or returns the Input sweep mode. \nParameters \n<ch> Any existing channel number. If unspecified, value is set to 1. \n<char> Input sweep mode. Choose either FIXED or SWEPT \nExamples SENS:MIX:INP:FREQ:MODE FIXED \nSENSe2:MIXer:INP:FREQ:MODE swept \nQuery Syntax SENSe<ch>:MIXer:INPut:FREQuency:MODE? \nReturn Type Character \nDefault Fixed \nSENSe<ch>:MIXer:INPut:FREQuency:NUMerator <value> \n(Read-Write) Sets or returns the numerator value of the Input Fractional Multiplier. \nParameters \n<ch> Any existing channel number. If unspecified, value is set to 1. \n<value> Input numerator value. \nExamples SENS:MIX:INP:FREQ:NUM 3 \nSENSe2:MIXer:INPut:FREQ:NUMerator 1 \nQuery Syntax SENSe<ch>:MIXer:INPut:FREQ:NUMerator? \nReturn Type Numeric \nDefault Not Applicable \nSENSe<ch>:MIXer:INPut:FREQuency:STARt <value> \n1769\n\n(Read-Write) Sets or returns the Input start frequency value of the mixer. \nParameters \n<ch> Any existing channel number. If unspecified, value is set to 1. \n<value> Input Start frequency \nExamples SENS:MIX:INP:FREQ:STAR 1e9 \nSENSe2:MIXer:INPut:FREQ:STARt 1000000000 \nQuery Syntax SENSe<ch>:MIXer:INPut:FREQuency:STARt? \nReturn Type Numeric \nDefault Not Applicable \nSENSe<ch>:MIXer:INPut:FREQuency:STOP <value> \n(Read-Write) Sets or returns the Input stop frequency value of the mixer. \nParameters \n<ch> Any existing channel number. If unspecified, value is set to 1. \n<value> Input stop frequency \nExamples SENS:MIX:INP:FREQ:STOP 2e9 \nSENSe2:MIXer:INPut:FREQ:STOP 2000000000 \nQuery Syntax SENSe<ch>:MIXer:INPut:FREQuency:STOP? \nReturn Type Numeric \nDefault Not Applicable \nSENSe<ch>:MIXer:INPut:POWer <value> \n(Read-Write) Sets or returns the value of the Input Power. \nParameters \n<ch> Any existing channel number. If unspecified, value is set to 1. \n<value> Input power in dBm. \nExamples SENS:MIX:INP:POW 9 \nSENSe2:MIXer:INPut:POWer 5 \nQuery Syntax SENSe<ch>:MIXer:INPut:POWer? \nReturn Type Numeric \nDefault Not Applicable \n1770\n\nSENSe<ch>:MIXer:INPut:POWer:USENominal <bool> \n(Read-Write) Toggles the Nominal Incident Power setting ON and OFF. This setting is ONLY to be \nused with SMC measurements, not VMC. Learn more about Nominal Incident Power. \nParameters \n<ch> Any existing channel number. If unspecified, value is set to 1. \n<value> (boolean) - Nominal Incident Power State. Choose from: \nTrue (1) - Turn nominal incident power ON \nFalse (0) - Turn nominal incident power OFF \nExamples SENS:MIX:INP:POW:USEN 1 \nSENSe2:MIXer:INPut:POWer:USENominal false \nQuery Syntax SENSe<ch>:MIXer:INPut:POWer:USENominal? \nReturn Type Boolean \nDefault False \nSENSe<ch>:MIXer:LO<n>:FREQuency:DENominator <value> \n(Read-Write) Sets or returns the denominator value of the LO Fractional Multiplier. \nParameters \n<ch> Any existing channel number. If unspecified, value is set to 1. \n<n> LO stage number. Choose 1 or 2. \n<value> LO denominator. \nExamples SENS:MIX:LO:FREQ:DEN 5 \nSENSe2:MIXer:LO2:FREQ:DENominator 4 \nQuery Syntax SENSe<ch>:MIXer:LO<n>:FREQuency:DENominator? \nReturn Type Numeric \nDefault 1 \nSENSe<ch>:MIXer:LO<n>:FREQuency:FIXed <value> \n1771\n\n(Read-Write) Sets or returns the fixed frequency of the specified mixer LO. \nParameters \n<ch> Any existing channel number. If unspecified, value is set to 1. \n<n> LO stage number. Choose 1 or 2 \n<value> LO frequency. \nExamples SENS:MIX:LO:FREQ:FIX 1e9 \nSENSe2:MIXer:LO2:FREQ:FIXed 1000000000 \nQuery Syntax SENSe<ch>:MIXer:LO<n>:FREQuency:FIXed? \nReturn Type Numeric \nDefault Not Applicable \nSENSe<ch>:MIXer:LO<n>:FREQuency:ILTI <bool> \n(Read-Write) Specifies whether to use the Input frequency that is greater than the LO or less than \nthe LO. To learn more, see the mixer setup dialog box help. \nParameters \n<ch> Any existing channel number. If unspecified, value is set to 1. \n<n> LO stage number. Choose 1 or 2 \n<bool> True (1) - Use the Input that is Greater than the specified LO. \nFalse (0) - Use the Input that is Less than the specified LO. \nExamples SENS:MIX:LO1:FREQ:ILTI 1 \nsense2:mixer:lo2:frequency:ilti true \nQuery Syntax SENSe<ch>:MIXer:LO<n>:FREQuency:ILTI? \nReturn Type Boolean \nDefault False \nSENSe<ch>:MIXer:LO<n>:FREQuency:MODE <char> \n1772\n\n(Read-Write) Sets or returns the LO sweep mode. \nParameters \n<ch> Any existing channel number. If unspecified, value is set to 1. \n<n> LO stage number. Choose 1 or 2 \n<char> LO sweep mode. Choose either FIXED or SWEPT \nExamples SENS:MIX:LO:FREQ:MODE FIXED \nSENSe2:MIXer:LO2:FREQ:MODE swept \nQuery Syntax SENSe<ch>:MIXer:LO<n>:FREQuency:MODE? \nReturn Type Character \nDefault Fixed \nSENSe<ch>:MIXer:LO<n>:FREQuency:NUMerator <value> \n(Read-Write) Sets or returns the numerator value of the LO Fractional Multiplier. \nParameters \n<ch> Any existing channel number. If unspecified, value is set to 1. \n<n> LO stage number. Choose 1 or 2 \n<value> LO Numerator. \nExamples SENS:MIX:LO:FREQ:NUM 5 \nSENSe2:MIXer:LO2:FREQ:NUMerator 4 \nQuery Syntax SENSe<ch>:MIXer:LO<n>:FREQuency:NUMerator? \nReturn Type Numeric \nDefault Not Applicable \nSENSe<ch>:MIXer:LO<n>:FREQuency:STARt <value> \n1773\n\n(Read-Write) Sets or returns the LO start frequency value. \nParameters \n<ch> Any existing channel number. If unspecified, value is set to 1. \n<n> LO stage number. Choose 1 or 2 \n<value> LO Start Frequency in Hertz. \nExamples SENS:MIX:LO:FREQ:STAR 5E9 \nQuery Syntax SENSe<ch>:MIXer:LO<n>:FREQuency:STARt? \nReturn Type Numeric \nDefault Not Applicable \nSENSe<ch>:MIXer:LO<n>:FREQuency:STOP <value> \n(Read-Write) Sets or returns the LO stop frequency value. \nParameters \n<ch> Any existing channel number. If unspecified, value is set to 1. \n<n> LO stage number. Choose 1 or 2 \n<value> LO Stop Frequency in Hertz. \nExamples SENS:MIX:LO:FREQ:STOP 5E9 \nQuery Syntax SENSe<ch>:MIXer:LO<n>:FREQuency:STOP? \nReturn Type Numeric \nDefault Not Applicable \nSENSe<ch>:MIXer:LO<n>:NAME <value> \n1774\n\n(Read-Write) Sets or returns the name of the previously-configured external LO source. The external \nLO source must be configured and calibrated manually; there are no programming commands to \naccomplish this. The source must also be properly connected. \nParameters \n<ch> Any existing channel number. If unspecified, value is set to 1. \n<n> LO stage number. Choose 1 or 2. \n<value> External LO source name \nExamples SENS:MIX:LO:NAME \"MySource\" \nQuery Syntax SENSe<ch>:MIXer:LO<n>:NAME? \nReturn Type String \nDefault Not Controlled \nSENSe<ch>:MIXer:LO<n>:POWer <value> \n(Read-Write) Sets or returns the value of the LO Power. \nParameters \n<ch> Any existing channel number. If unspecified, value is set to 1. \n<n> LO stage. Choose 1 or 2 \n<value> LO Power in dBm \nExamples SENS:MIX:LO:POW 9 \nQuery Syntax SENSe<ch>:MIXer:LO<n>:POWer? \nReturn Type Numeric \nDefault Not Applicable \nSENSe<ch>:MIXer:OUTPut:FREQuency:FIXed <value> \n1775\n\n(Read-Write) Sets or returns the output fixed frequency of the mixer. \nParameters \n<ch> Any existing channel number. If unspecified, value is set to 1. \n<value> Output fixed frequency in Hertz. \nExamples SENS:MIX:OUTP:FREQ:FIX 5e9 \nQuery Syntax SENSe<ch>:MIXer:OUTPut:FREQuency:FIXed? \nReturn Type Numeric \nDefault Not Applicable \nSENSe<ch>:MIXer:OUTPut:FREQuency:MODE <char> \n(Read-Write) Sets or returns the Output sweep mode. \nParameters \n<ch> Any existing channel number. If unspecified, value is set to 1. \n<char> Output sweep mode. Choose either FIXED or SWEPT \nExamples SENS:MIX:OUT:FREQ:MODE FIXED \nSENSe2:MIXer:OUTput:FREQuency:MODE swept \nQuery Syntax SENSe<ch>:MIXer:OUTPut:FREQuency:MODE? \nReturn Type Character \nDefault Fixed \nSENSe<ch>:MIXer:OUTPut:FREQuency:SIDeband <value> \n1776\n\n(Read-Write) Sets or returns the value of the output sideband. \nParameters \n<ch> Any existing channel number. If unspecified, value is set to 1. \n<value> Boolean Sideband value. Choose from \nLOW - Low or Difference (-) \nHIGH - High or Sum (+) \nExamples SENS:MIX:OUTP:FREQ:SIDe LOW \nSENSe2:MIXer:OUTPut:FREQ:SIDeband HIGH \nQuery Syntax SENSe<ch>:MIXer:OUTPut:FREQuency:SIDeband? \nReturn Type Character \nDefault LOW \nSENSe<ch>:MIXer:OUTPut:FREQuency:STARt <value> \n(Read-Write) Sets or returns the Output start frequency of the mixer. \nParameters \n<ch> Any existing channel number. If unspecified, value is set to 1. \n<value> Output start frequency \nExamples SENS:MIX:OUTP:FREQ:STAR 1e9 \nSENSe2:MIXer:OUTPut:FREQ:STARt 1000000000 \nQuery Syntax SENSe<ch>:MIXer:OUTPut:FREQuency:STARt? \nReturn Type Numeric \nDefault Not Applicable \nSENSe<ch>:MIXer:OUTPut:FREQuency:STOP <value> \n1777\n\n(Read-Write) Sets or returns the Output stop frequency of the mixer. \nParameters \n<ch> Any existing channel number. If unspecified, value is set to 1. \n<value> Output stop frequency \nExamples SENS:MIX:OUTP:FREQ:STOP 1e9 \nSENSe2:MIXer:OUTPut:FREQ:STOP 1000000000 \nQuery Syntax SENSe<ch>:MIXer:OUTPut:FREQuency:STOP? \nReturn Type Numeric \nDefault Not Applicable \n1778\n\nSense:Multiplexer Commands \nControls External Test Sets (N44xx, E5091A, and Special Opts). \nClick on a blue keyword to view the command details. \nRed commands are superseded. \nSee Also \nSee an example program using these commands. \nLearn about External Test Set Control \nSynchronizing the PNA and Controller \nSCPI Command Tree \nSENSe:MULTiplexer<id>:ADDRess <address> \n(Read-Write) Sets and returns the address for the external test set at the specified ID. This command \nshould be immediately preceded by the SENSe:MULT:TYPE command. \nParameters \n<id> Id of the external test set. If unspecified, Id is assumed to be 1. Must be \npreviously set by the SENSe:MULT:TYPE command. \n<address> Integer The test set address. \nFor a GPIB test set (N44xx and some specials), this is the GPIB address. \nFor a test set I/O test set (some specials), it is the position of the test set in the chain \n(starting at 0). \nFor USB test sets (E5091A), the address is set by DIP switches on the rear panel. \n1779\n\nExamples SENS:MULT1:TYPE \"Z5623A_K66\" ' use K66 test set, and reference it \nthrough ID 1 \nSENS:MULT1:ADDR 0 ' first test set in sequence \n' All subsequent commands using SENS:MULT1 will refer to this \ntest set \nQuery Syntax SENSe:MULTiplexer<id>:ADDRess? \nReturn Type Numeric \nDefault Not Applicable \nSENSe<cnum>:MULTiplexer<id>:ALLPorts <string> \n(Read-Write) Sets or gets the port selections for all available ports on the specified channel. \nParameters \n<cnum> Any existing channel number. If unspecified, value is set to 1. \n<id> Id of the external test set. If unspecified, Id is assumed to be 1. Must be \npreviously set by the SENSe:MULT:TYPE command. \n<string> Comma-separated list of port selections, one for each port. Each port selection \nmust correspond to one of the values returned by SENS:MULT:PORT:CAT?. \nDo NOT include + and - . \nExamples ' for channel 5 and test set 1, set port 1 to T1, \n' port 2 to A, port 3 to R2+, port 4 to R3-. \nSENS5:MULT1:ALLP \"T1,A,R2,R3 \" \nQuery Syntax SENSe<cnum>:MULTiplexer<id>:ALLPorts? \nReturn Type STRING \nDefault Not Applicable \nSENSe:MULTiplexer:CATalog? \n(Read-Only) Returns a comma-separated list of the external test sets models that are currently \nsupported. Choose one of these items to send SENS:MULT1:TYPE. \nExamples SENS:MULT:CAT? \nReturn Type String \nDefault Not Applicable \n1780\n\nSENSe:MULTiplexer<id>:COUNt? \n(Read-Only) Returns the total number of ports of the specified test set. \nReturns 0 if no test set is connected (GPIB test sets only). \nParameters \n<id> Id of the external test set. If unspecified, Id is assumed to be 1. Must be \npreviously set by the SENSe:MULT:TYPE command. \nExamples SENS:MULT1:COUN? \nsense:multiplexer2:count? \nReturn Type Numeric \nDefault Not Applicable \nSENSe:MULTiplexer<id>:DISPlay[:STATe] <bool> \n(Read-Write) Turns ON and OFF the display of the test set control status bar. This status bar indicates \nthe test set that is being controlled and the current port mappings. This setting is turned ON \nautomatically when the test set is enabled. \nParameters \n<id> Id of the external test set. If unspecified, Id is assumed to be 1. Must be \npreviously set by the SENSe:MULT:TYPE command. \n<bool> ON(1) Turns ON the display. \nOFF (0) Turns OFF the display. \nExamples SENS:MULT1:DISP 1 \nsense:multiplexer2:display:state on \nQuery Syntax SENSe:MULTiplexer<id>:DISPlay[:STATe]? \nReturn Type Boolean \nDefault OFF (0) \nSENSe:MULTiplexer<id>:INCount? \n1781\n\n(Read-Only) Returns the number of input ports for the specified test set. \nFor test sets such as the E5091A that do NOT use jumper cables to route the stimulus and response signals, \nthis command returns the number of test set ports that can be connected to the PNA. \nFor test sets that DO use jumper cables to route the stimulus and response signals, such as the N44xx, the \nreturn value is not valid. \nParameters \n<id> Id of the external test set. If unspecified, Id is assumed to be 1. Must be \npreviously set by the SENSe:MULT:TYPE command. \nExamples SENS3:MULT1:INC? ' returns the number of input ports for test \nset 1 on channel 3 \nReturn Type Numeric \nDefault Not Applicable \nSENSe<cnum>:MULTiplexer:LABel <string> \n(Read-Write) Sets and returns the display label for the testset on the specified channel. The label \nappears in a status bar at the bottom of the PNA display when SENS:MULT:DISP is set to TRUE. \nParameters \n<cnum> Any existing channel number. If unspecified, value is set to 1. \n<string> Display label text. \nExamples SENS3:MULT:LAB 'High-power output' \nQuery Syntax SENSe<cnum>:MULTiplexer:LABel? \nReturn Type String \nDefault Not Applicable \nSENSe<cnum>:MULTiplexer<id>:OUTPut[:DATa] <num> \n1782\n\n(Read-Write) Sets or returns the control line value for the specified channel. \nParameters \n<cnum> Any existing channel number. If unspecified, value is set to 1. \n<id> Id of the external test set. If unspecified, Id is assumed to be 1. Must be \npreviously set by the SENSe:MULT:TYPE command. \n<numr> An integer specifying the decimal value of the control line. Values are obtained \nby adding weights from the following table that correspond to individual lines. \nHIGH =1; LOW=0. \nLine Weight \n1 1 \n2 2 \n3 4 \n4 8 \n5 16 \n6 32 \n7 64 \n8 128 \n0 - Sets all lines low \n255 - Sets all lines high \nExamples SENS3:MULT1:OUTP 48 'For test set 1 on channel 3, sets lines 5 \nand 6 to HIGH state; all other lines are set to LOW state. \nQuery Syntax SENSe<cnum>:MULTiplexer<id>:OUTPut[:DATa]? \nReturn Type Numeric \nDefault Not Applicable \nSENSe:MULTiplexer<id>:PORT<pnum>CATalog? \n1783\n\n(Read-Only) Returns a comma-separated list of valid port selections for the specified port. \nParameters \n<id> Id of the external test set. If unspecified, Id is assumed to be 1. Must be \npreviously set by the SENSe:MULT:TYPE command. \n<pnum> Integer - Input port number for which to return valid Output port selections. \nRead the number of input ports for the test set using SENS:MULT:INCount? \nExamples SENS:MULT1:PORT3:CAT? ' returns the valid port selections for \nport 3 \nReturn Type String \nDefault Not Applicable \nSENSe<cnum>:MULTiplexer<id>:PORT<logi>SELect <phys> \n(Write-Only) Sets and returns a port mapping for a single port. If this command creates a conflict with \nan existing port, the PNA will resolve the conflict. \nNote: This command is currently not supported for the Z5623AK44. \nParameters \n<cnum> Channel number of the measurement. If unspecified, value is set to 1. \n<id> Id of the external test set. If unspecified, Id is assumed to be 1. Must be \npreviously set by the SENSe:MULT:TYPE command. \n<logi> Integer - Logical port number. \n<string> String - Physical port number. \nExamples SENS:MULT1:PORT3:SEL \"4\" 'sets logical port 3 to physical port \n4. \nReturn Type String \nDefault Not Applicable \nSENSe:MULTiplexer<id>:STATe <bool> \n1784\n\n(Read-Write) Enables and disables (ON/OFF) the port mapping and control line output of the \nspecified test set. \nIf the specified test set is not connected or not ON, then setting State ON will report an error. All other \nproperties can be set when the test set is not connected. \nWhen this command is set to ON, then the display of the test set status bar (SENS:MULT:DISP) is \nalso set to ON. \nParameters \n<id> Id of the external test set. If unspecified, Id is assumed to be 1. Must be \npreviously set by the SENSe:MULT:TYPE command. \n<bool> ON(1) Enables test set control. \nOFF (0) Disables test set control. \nExamples SENS:MULT1:STAT 1 \nsense2:multiplexer2:state on \nQuery Syntax SENSe<cnum>:MULTiplexer<id>:STATe? \nReturn Type Boolean \nDefault OFF (0) \nSENSe<cnum>:MULTiplexer<id>:TSET9:OUTPut[:DATA] <data> Superseded \nNote: This command is replaced with SENS:MULT:OUTP \n(Read-Write) Sets the control lines of the specified E5091A. Control lines, provided through a \nE5091A front panel connector, are used to control external equipment such as a part handler. See your \nE5091A documentation to learn more about control lines. \nParameters \n<cnum> Channel number of the measurement. If unspecified, value is set to 1. \n<id> Id of the E5091A test set. Choose from 1 or 2. Learn how to set ID value. \n<data> Data value used to set control lines. Values are obtained by adding weights \nfrom the following table that correspond to individual lines. HIGH =1; \nLOW=0. \n1785\n\nLine Weight \n1 1 \n2 2 \n3 4 \n4 8 \n5 16 \n6 32 \n7 64 \n8 128 \n0 - Sets all lines low \n255 - Sets all lines high \nExamples 'The following sets line 3 and 4 high. All other lines low. \nSENS:MULT1:TSET9:OUTP 12 \nQuery Syntax SENSe<cnum>:MULTiplexer<id>:TSET9:OUTPut[:DATA]? \nReturn Type Numeric \nDefault 0 \nSENSe<cnum>:MULTiplexer<id>:TSET9:PORT1 <char> Superseded \nNote: This command is replaced with SENS:MULT:ALLPorts which sets ALL ports to the specified \noutputs. \n(Read-Write) Switches Port 1 of the specified E5091A to one of the available outputs. \nParameters \n<cnum> Any existing channel number; if unspecified, value is set to 1. \n<id> Id of the E5091A test set. Choose from 1 or 2. Learn how to set ID value. \n<char> Output port to be switched to. Choose from: \nA\nT1 - (If Port 2 already is connected to T1, then Port 2 will be switched to T2.) \nExamples SENS:MULT1:TSET9:PORT1 A \nQuery Syntax SENSe<cnum>:MULTiplexer<id>:TSET9:PORT1? \n1786\n\nReturn Type Character \nDefault A \nSENSe<cnum>:MULTiplexer<id>:TSET9:PORT2 <char> Superseded \nNote: This command is replaced with SENS:MULT:ALLPorts which sets ALL ports to the specified \noutputs. \n(Read-Write) Switches Port 2 of the specified E5091A to one of the available outputs. \nParameters \n<cnum> Any existing channel number; if unspecified, value is set to 1. \n<id> Id of the E5091A test set. Choose from 1 or 2. Learn how to set ID value. \n<char> Output port to be switched to. Choose from: \nT1 - If Port 1 already is connected to T1, then Port 1 will be switched to A. \nT2 \nExamples SENS:MULT1:TSET9:PORT2 T2 \nQuery Syntax SENSe<cnum>:MULTiplexer<id>:TSET9:PORT2? \nReturn Type Character \nDefault T1 \nSENSe<cnum>:MULTiplexer<id>:TSET9:PORT3 <char> Superseded \nNote: This command is replaced with SENS:MULT:ALLPorts which sets ALL ports to the specified \noutputs. \n(Read-Write) Switches Port 3 of the specified E5091A to one of the available outputs. \nParameters \n<cnum> Any existing channel number; if unspecified, value is set to 1. \n<id> Id of the E5091A test set. Choose from 1 or 2. Learn how to set ID value. \n<char> Output port to be switched to. Choose from: \nR1 (R1+) \nR2 (R2+) \n1787\n\nR3 (R3+) If option 007 (7port), R2 is selected. \nExamples SENS:MULT1:TSET9:PORT3 R2 \nQuery Syntax SENSe<cnum>:MULTiplexer<id>:TSET9:PORT3? \nReturn Type Character \nDefault R1 \nSENSe<cnum>:MULTiplexer<id>:TSET9:PORT4 <char> Superseded \nNote: This command is replaced with SENS:MULT:ALLPorts which sets ALL ports to the specified \noutputs. \n(Read-Write) Switches Port 4 of the specified E5091A to one of the available outputs. \nParameters \n<cnum> Any existing channel number; if unspecified, value is set to 1. \n<id> Id of the E5091A test set. Choose from 1 or 2. Learn how to set ID value. \n<char> Output port to be switched to. Choose from: \nR1 (R1-) \nR2 (R2-) \nR3 (R3-) If option 007 (7port), R2 is selected. \nExamples SENS:MULT1:TSET9:PORT4 R2 \nQuery Syntax SENSe<cnum>:MULTiplexer<id>:TSET9:PORT4? \nReturn Type Character \nDefault R1 \nSENSe:MULTiplexer<id>:TYPe <name> \n1788\n\n(Read-Write) Loads a configuration file for the specified type of external test set. \nThis command should be immediately followed by the SENSe:MULT:ADDRess command. \nParameters \n<name> \nString The name of the type of test set. Must be one of the items in the list \nreturned by the SENSe:MULT:CATalog? query. \n<id> Id of the external test set. Set by this command. Use consecutive values starting \nat 1. \nExamples SENS:MULT1:TYPE \"Z5623AK66\" ' use K66 test set, and reference \nit through ID 1 \nQuery Syntax SENSe:MULTiplexer<id>:TYPe? \nReturn Type String \nDefault Not Applicable \n1789\n\nSense:Offset Commands \nSets the offset frequency functions, causing the stimulus and response frequencies to be different. \nClick on a blue keyword to view the command details. \nSee Also \nExample Programs \nLearn about Frequency Offset \nSynchronizing the PNA and Controller \nSCPI Command Tree \nSENSe<cnum>:OFFSet:CW <bool> \n(Read-Write) Turns stimulus CW Override mode ON or OFF. Use this setting to establish a fixed \n(CW) stimulus frequency while measuring the Response over a swept frequency range. \nParameters \n<cnum> Any existing channel number. If unspecified, value is set to 1 \n<bool> ON (or 1) - turns CW override ON. \nOFF (or 0) - turns CW overide OFF. \nExamples SENS:OFFS:CW ON \nsense2:offset:cw off \nQuery Syntax SENSe<cnum>:OFFSet:CW? \nReturn Type Boolean \nDefault OFF \nSENSe<cnum>:OFFSet:DIVisor <num> \n1790\n\n(Read-Write) Specifies (along with the multiplier) the value to multiply by the stimulus. \nParameters \n<cnum> Any existing channel number. If unspecified, value is set to 1 \n<num> Divisor value. Range is 1 to 1000 \nExamples SENS:OFFS:DIV 3 \nsense2:offset:divisor 2 \nQuery Syntax SENSe<cnum>:OFFSet:DIVisor? \nReturn Type Numeric \nDefault 1 \nSENSe<cnum>:OFFSet:MULTiplier <num> \n(Read-Write) Specifies (along with the divisor) the value to multiply by the stimulus. \nParameters \n<cnum> Any existing channel number. If unspecified, value is set to 1 \n<num> Multiplier value. Range is +/- 1000. Negative multipliers cause the stimulus to \nsweep in decreasing direction. For mixer measurements, this would be for \nsetups requiring the RF frequency to be less than LO frequency \nExamples SENS:OFFS:MULT 2 \nsense2:offset:multiplier 4 \nQuery Syntax SENSe<cnum>:OFFSet:MULTplier? \nReturn Type Numeric \nDefault 1 \nSENSe<cnum>:OFFSet:OFFSet <num> \n1791\n\n(Read-Write) Specifies an absolute offset frequency in Hz. For mixer measurements, this would be \nthe LO frequency. \nParameters \n<cnum> Any existing channel number. If unspecified, value is set to 1 \n<num> Offset frequency. Range is +/- 1000 GHz. Offsets can be positive or negative \nExamples SENS:OFFS:OFFS 1GHz \nsense2:offset:offset 1e9 \nQuery Syntax SENSe<cnum>:OFFSet:OFFSet? \nReturn Type Numeric \nDefault 0 Hz \nSENSe<cnum>:OFFSet:STARt? \n(Read-Only) Returns the response start frequency \nParameters \n<cnum> Any existing channel number. If unspecified, value is set to 1 \nExamples SENS:OFFS:STAR? \nsense2:offset:start? \nReturn Type Numeric \nDefault Not applicable \nSENSe<cnum>:OFFSet:[STATe] <bool> \n(Read-Write) Enables Frequency Offset Mode on ALL measurements that are present on the active \nchannel. This immediately causes the source and receiver to tune to separate frequencies. The receiver \nfrequencies are specified with the other SENS:OFFSet commands. To make the stimulus settings use \nthe SENS:FREQ commands. \nTip: To avoid unnecessary errors, first make other offset frequency settings, then set Frequency Offset \nON. \nParameters \n<cnum> Any existing channel number. If unspecified, value is set to 1 \n<bool> ON (or 1) - turns Frequency Offset ON. \nOFF (or 0) - turns Frequency Offset OFF. \n1792\n\nExamples SENS:OFFS ON \nsense2:offset:state off \nQuery Syntax SENSe<cnum>:OFFSet:[STATe]? \nReturn Type Boolean \nDefault OFF (0) \nSENSe<cnum>:OFFSet:STOP? \n(Read-Only) Returns the response stop frequency. \nParameters \n<cnum> Any existing channel number. If unspecified, value is set to 1 \nExamples SENS:OFFS:STOP \nsense2:offset:stop \nReturn Type Numeric \nDefault Not applicable \n1793\n\nSense:Path:Configuration Commands \nControls the path configuration settings. \nClick on a blue keyword to view the command details. \nSee Also \nExample Programs \nLearn about Path Configuration \nSynchronizing the PNA and Controller \nSCPI Command Tree \nSENSe:PATH:CONFiguration:CATalog? \n(Read-only) Returns a list of configuration names stored in the PNA. \nExamples SENS:PATH:CONF:CAT? \nReturn Type Comma-separated list of double-quoted strings \nDefault Not Applicable \nSENSe:PATH:CONFiguration:DELete <string> \n1794\n\n(Write-only) Deletes the specified configuration name from the PNA. The factory configurations cannot be \ndeleted. This is the only method of distinguishing a factory configuration from a user-named configuration. \nParameters \n<string> Configuration name to be deleted. \nExamples SENS:PATH:CONF:DEL \"MyMixer\" \nReturn Type Not Applicable \nDefault Not Applicable \nSENSe:PATH:CONFiguration:DTEXt <string> \n(Read-Write) Write and read descriptive text associated with the configuration. This text is displayed in the path \nconfiguration dialog. Text is generally used to describe external connections that must be made manually to \ncomplete the configuration setup. \nParameters \n<string> Descriptive text enclosed in quotes. Double quotes are not allowed within the descriptive \ntext. \nExamples SENS:PATH:CONF:DTEX \"Connect J1 jumper on the rear panel.\" \nQuery Syntax SENSe<ch>:PATH:CONFiguration:DTEXt? \nReturn Type String \nDefault Not Applicable \nSENSe<ch>:PATH:CONFiguration:ELEMent:CATalog? \n1795\n\n(Read-only) Returns the names of configurable elements as a comma-delimited list of strings. \nSee a list of configurable elements and settings for various PNA models. \nParameters \n<ch> Any existing channel number; if unspecified, value is set to 1. \nExamples SENS:PATH:CONF:ELEM:CAT? \n'returns \n�Combiner�, �Src1�, �Src2� \nDefault Not Applicable \nSENSe<ch>:PATH:CONFiguration:ELEMent[:STATe] <elem>, <setting> \n(Read-Write) Write or read the setting of a specified element in the current configuration. \nSee a list of configurable elements and settings for various PNA models. \nParameters \n<ch> Any existing channel number; if unspecified, value is set to 1. \n<elem> Name of the element for which a setting is to be made. \n<setting> Element setting. Use SENS:PATH:CONF:ELEM:VAL:CAT? to return a list of valid \nsettings for the specified element. \nExamples SENS:PATH:CONF:ELEM \"Combiner\",\"Normal\" \nQuery Syntax SENSe<ch>:PATH:CONFiguration:ELEMent? \"Combiner\" \nReturns the current state of the Combiner element. \nReturn Type String \nDefault Not applicable \nSENSe<ch>:PATH:CONFiguration:ELEMent:VALue:CATalog? <element> \n1796\n\n(Read-only) Returns the list of valid settings that can be used with the specified element. \nSee a list of configurable elements and settings for various PNA models. \nParameters \n<ch> Any existing channel number; if unspecified, value is set to 1. \n<element> String. Element name for which to return valid settings. \nExamples SENS:PATH:CONF:ELEM:VAL:CAT? \"Combiner\" \n'returns \"Normal\", \"Reversed\" \nDefault Not Applicable \nSENSe<ch>:PATH:CONFiguration:NAME? \n(Read-only) Returns the name of the current configuration only if NO individual element settings had been \nchanged since selecting or storing a configuration. When element settings change, the path configuration name is \ncleared. \nParameters \n<ch> Any existing channel number; if unspecified, value is set to 1. \nExamples SENS:PATH:CONF:NAME? \n'returns \"Default\" \nReturn Type String \nDefault Not Applicable \nSENSe<ch>:PATH:CONFiguration:SELect <string> \n1797\n\n(Write only) Loads the named configuration onto the specified channel. \nUse SENS:PATH:CONF:CAT? to return the configuration names that are stored on the PNA. \nParameters \n<ch> Any existing channel number; if unspecified, value is set to 1. \n<string> Configuration name. \"Default\" is the default factory configuration. \nExamples SENS:PATH:CONF:SEL 'default' \nsense2:path:configuration:select \"MyMixer\" \nQuery Syntax Not Applicable \nDefault \"Default\" \nSENSe<ch>:PATH:CONFiguration:STORe <name> \n(Write only) Saves the path configuration currently associated with channel <ch> to the specified configuration \nname. \nParameters \n<ch> Any existing channel number; if unspecified, value is set to 1. \n<name> String. Configuration name. Factory configurations can NOT be overwritten. Specifying \nthe name of a pre-defined factory configuration will result in an error. \nExamples SENS:PATH:CONF:STOR \"MyMixer\" \nQuery Syntax Not Applicable \nDefault Not Applicable \nLast Modified: \n14-Dec-6 MX New Topic \n1798\n\nSense:Power Command \nLearn about Receiver Attenuation \nSENSe<cnum>:POWer:ATTenuation <recvr>,<num> \n(Read-Write) Sets the attenuation level for the specified receiver. \nNote: Attenuation cannot be set with Sweep Type set to Power \nParameters \n<cnum> Any existing channel number. If unspecified, value is set to 1 \n<recvr> Receiver to get attenuation. Choose from: \nARECeiver - receiver A \nBRECeiver - receiver B \nReceiver attenuation can not be set using logical receiver notation. \n<num> Choose from: \n0 to 35 dB - in 5 dB steps \nIf a number other than these is entered, the analyzer will select the next lower \nvalid value. For example, if 19.9 is entered for <num> the analyzer will switch \nin 15 dB attenuation. \nExamples SENS:POW:ATT AREC,10 \nsense2:power:attentuation breceiver,30 \nQuery Syntax SENSe<cnum>:POWer:ATTenuation? <rec> \nReturn Type Numeric \nDefault 0 \n1799\n\nSense:Pulse Commands \nConfigures the 5 pulse generators in the PNA-X. \nClick on a blue keyword to view the command details. \nPulse Definitions \nD = Delay; the time before each pulse begins \nW = Width; the time the pulse is ON \nP = Period; one complete pulse cycle \nDuty Cycle = W/P \nImportant: If D + W is greater than P, then undefined PNA behavior results. There is NO error \nmessage or warning. \nSee Also \nPNA-X IF Path Block diagram \nSENS:IF configuration commands \nExample Programs \nPNA-X Pulse Application \nSynchronizing the PNA and Controller \nSCPI Command Tree \n1800\n\nSENSe<ch>:PULSe<n>:DELay <value> \n(Read-Write) Sets the pulse delay. The amount of time before a new pulse begins. \nSee Pulse Definition diagram. \nParameters \n<ch> Any existing channel number; if unspecified, value is set to 1. \n<n> Pulse generator number. Choose from 0 to 4. \n0 is the generator that pulses the ADC. \n<value> Delay value in seconds. Choose a value from about 33ns to about 70 seconds. \nExamples SENS:PULS:DEL .5 \nQuery Syntax SENSe<ch>:PULSe<n>:DELay? \nReturn Type Numeric \nDefault 0 \nSENSe<ch>:PULSe<n>:DINCrement <value> \n(Read-Write) Sets the pulse delay increment. The delay increments with each pulse by the <value> \namount. \nFor example, in this diagram the delay starts as 1. On the second pulse, delay=2. On the third pulse, \ndelay=3. \nImportant: If D + W is greater than P, then undefined PNA behavior results. There is NO error \nmessage or warning. Delay includes the incremented value. \nThis is useful for pulse profiling. \nSee Pulse Definition diagram. \nParameters \n<ch> Any existing channel number; if unspecified, value is set to 1. \n1801\n\n<n> Pulse generator number. Choose from 0 to 4. \n0 is the generator that pulses the ADC. \n<value> Delay increment value in seconds. \nExamples SENS:PULS:DINC .5 \nQuery Syntax SENSe<ch>:PULSe<n>:DINCrement? \nReturn Type Numeric \nDefault 0 \nSENSe<ch>:PULSe:PERiod <value> \n(Read-Write) Sets the pulse-period (1/PRF) for ALL pulse generators. \nThe resolution of the period is 16.667nS. \nSee Pulse Definition diagram. \nParameters \n<ch> Any existing channel number; if unspecified, value is set to 1. \n<value> Pulse period in seconds. Choose a value from about 33ns to about 70 seconds. \nExamples SENS:PULS:PERiod .5 \nQuery Syntax SENSe<ch>:PULSe:PERiod? \nReturn Type Numeric \nDefault 1e-3 sec \nSENSe<ch>:PULSe<n>:STATe <bool> \n1802\n\n(Read-Write) Turns the pulse output ON and OFF. \nParameters \n<ch> Any existing channel number; if unspecified, value is set to 1. \n<n> Pulse generator number. Choose from 0 to 4. \n0 is the generator that pulses the ADC. \n<bool> ON (or 1) - turns pulse output ON. \nOFF (or 0) - turns pulse output OFF. \nExamples SENS:PULS:STAT 1 \nQuery Syntax SENSe<ch>:PULSe:STATe? \nReturn Type Boolean \nDefault OFF \nSENSe<ch>:PULSe<n>:WIDTh <value> \n(Read-Write) Sets the pulse width. The amount of time that the pulse is ON. \nSee Pulse Definition diagram. \nParameters \n<ch> Any existing channel number; if unspecified, value is set to 1. \n<n> Pulse generator number. Choose from 0 to 4. \n0 is the generator that pulses the ADC. \n<value> Pulse width in seconds. Choose a value from about 33ns to about 70 seconds. \nExamples SENS:PULS:WIDT .5 \nQuery Syntax SENSe<ch>:PULSe<n>:WIDTh? \nReturn Type Numeric \nDefault 1e-4 sec \nLast Modified: \n2-Jan-2007 MX New topic \n1803\n\nSense:Roscillator Command \nLearn about the Reference Osc. \nSENSe:ROSCillator:SOURce? \n(Read-only) Applying a signal to the Reference Oscillator connector automatically sets the Reference \nOscillator to EXTernal. This command allows you to check that it worked. \nEXT is returned when a signal is present at the Reference Oscillator connector. \nINT is returned when NO signal is present at the Reference Oscillator connector. \nExamples SENS:ROSC:SOUR? \nsense:roscillator:source? \nReturn Type Character \nDefault Not applicable \n1804\n\nSense:Segment Commands \nDefines the segment sweep settings. Enable segment sweep with SENS:SWE:TYPE SEGMent. \nClick on a blue keyword to view the command details. \nSee Also \nExample Programs \nLearn about Segment Sweep \nSynchronizing the PNA and Controller \nSCPI Command Tree \nSENSe<cnum>:SEGMent<snum>:ADD \n(Write-only) Adds a segment. \nParameters \n<cnum> Any existing channel number. If unspecified, value is set to 1 \n<snum> Segment number to add. If unspecified, value is set to 1. Segment numbers must \nbe sequential. If a new number is added where one currently exists, the existing \nsegment and those following are incremented by one. \nExamples Two Segments exist (1 and 2). The following command will add a new segment (1). The \nexisting (1 and 2) will become (2 and 3) respectively. \nSENS:SEGM1:ADD \nsense2:segment1:add \nQuery Syntax Not applicable. Use Sense:Segment:Count to determine the number of segments in a \ntrace. \nDefault Not Applicable \nSENSe<cnum>:SEGMent:ARBitrary <ON | OFF> \n1805\n\n(Read-Write) Enables you to setup a segment sweep with arbitrary frequencies. The start and stop \nfrequencies of each segment can overlap other segments. Also, each segment can have a start \nfrequency that is greater than its stop frequency which causes a reverse sweep over that segment. \nLearn more about Arbitrary Segment Sweep. \nParameters \n<cnum> Any existing channel number. If unspecified, value is set to 1. \n<ON | OFF> ON (or 1) - Allows the setup of arbitrary segment sweep. \nOFF (or 0) - Prevents the setup of arbitrary segment sweep. \nExamples SENS:SEGM:ARB ON \nsense2:segment:arbitrary off \nQuery Syntax SENSe<cnum>:SEGMent:ARBitrary? \nReturn Type Boolean (1 = ON, 0 = OFF) \nDefault OFF \nSENSe<cnum>:SEGMent<snum>:BWIDth[:RESolution] <num> \n(Read-Write) Sets the IF Bandwidth for the specified segment. First set \nSENS:SEGM:BWIDth:CONTrol ON. All subsequent segments that are added assume the \nnew IF Bandwidth value. \nParameters \n<cnum> Any existing channel number. If unspecified, value is set to 1 \n<snum> Segment number to modify. Choose any existing segment number. \n<num> IF Bandwidth in Hz. The list of valid IF Bandwidths is different depending on \nthe PNA model. (Click to see the lists.) If an invalid number is specified, the \nanalyzer will round up to the closest valid number. \nNote: This command will accept MIN or MAX instead of a numeric parameter. \nSee SCPI Syntax for more information. \nExamples SENS:SEGM:BWID 1KHZ \nsense2:segment2:bwidth:resolution max \nQuery Syntax SENSe<cnum>:SEGMent<snum>:BWIDth[:RESolution]? \nReturn Type Numeric \nDefault See Preset IFBW for your PNA model. \nSENSe<cnum>:SEGMent:BWIDth[:RESolution]:CONTrol <ON | OFF> \n1806\n\n(Read-Write) Specifies whether the IF Bandwidth resolution can be set independently for each \nsegment. \nParameters \n<cnum> Any existing channel number. If unspecified, value is set to 1 \n<ON | OFF> ON (or 1) - turns Bandwidth control ON. Bandwidth can be set for each \nsegment \nOFF (or 0) - turns Bandwidth control OFF. Use channel bandwidth setting \nExamples SENS:SEGM:BWID:CONT ON \nsense2:segment:bwidth:control off \nQuery Syntax SENSe<cnum>:SEGMent:BWIDth[:RESolution]:CONTrol? \nReturn Type Boolean (1 = ON, 0 = OFF) \nDefault OFF \nSENSe<cnum>:SEGMent:COUNt? \n(Read-only) Queries the number of segments that exist in the specified channel. \nParameters \n<cnum> Any existing channel number. If unspecified, value is set to 1 \nExamples SENS:SEGM:COUNt? \nsense2:segment:count? \nReturn Type Numeric \nDefault 1 segment \nSENSe<cnum>:SEGMent<snum>:DELete \n(Write-only) Deletes the specified sweep segment. When ALL segments are deleted, Sweep Mode \n(SENS:SWE:MODE) is automatically set to Linear because there are no segments to sweep. \n<cnum> Any existing channel number. If unspecified, value is set to 1 \n<snum> Number of the segment to delete. If unspecified, value is set to 1 \nExamples SENS:SEGM:DEL \nsense2:segment2:delete \nQuery Syntax Not applicable \nDefault Not Applicable \n1807\n\nSENSe<cnum>:SEGMent:DELete:ALL \n(Write-only) Deletes all sweep segments. When this command is executed, Sweep Mode \n(SENS:SWE:MODE) is automatically set to Linear because there are no segments to sweep. \nParameters \n<cnum> Any existing channel number. If unspecified, value is set to 1 \nExamples SENS:SEGM:DEL:ALL \nsense2:segment:delete:all \nQuery Syntax Not applicable \nDefault Not Applicable \nSENSe<cnum>:SEGMent<snum>:FREQuency:CENTer <num> \n(Read-Write) Sets the Center Frequency for the specified segment. The Frequency Span of the \nsegment remains the same. The Start and Stop Frequencies change accordingly. \nNote: All previous segment's Start and Stop Frequencies that are larger than the new Start Frequency \nare changed to the new Start Frequency. All following segment's start and stop frequencies that are \nsmaller than the new Stop Frequency are changed to the new Stop Frequency. \nParameters \n<cnum> Any existing channel number. If unspecified, value is set to 1 \n<snum> Segment number to modify. Choose any existing segment number. \n<num> Center Frequency in Hz. Choose any number between the minimum and \nmaximum frequency of the analyzer. \nNote: This command will accept MIN or MAX instead of a numeric parameter. \nSee SCPI Syntax for more information. \nExamples SENS:SEGM:FREQ:CENT 1MHZ \nsense2:segment2:frequency:center 1e9 \nQuery Syntax SENSe<cnum>:SEGMent<snum>:FREQuency:CENTer? \nReturn Type Numeric \nDefault Stop Frequency of the previous segment. If first segment, start frequency of the \nanalyzer. \nSENSe<cnum>:SEGMent<snum>:FREQuency:SPAN <num> \n1808\n\n(Read-Write) Sets the Frequency Span for the specified segment. The center frequency of the segment \nremains the same. The start and stop frequencies change accordingly. \nNote: All previous segment's Start and Stop Frequencies that are larger than the new Start Frequency \nare changed to the new Start Frequency. All following segment's start and stop frequencies that are \nsmaller than the new Stop Frequency are changed to the new Stop Frequency. \nParameters \n<cnum> Any existing channel number. If unspecified, value is set to 1 \n<snum> Segment number to modify. Choose any existing segment number. \n<num> Frequency Span in Hz. Choose any number between the minimum and \nmaximum frequency of the analyzer. \nNote: This command will accept MIN or MAX instead of a numeric parameter. \nSee SCPI Syntax for more information. \nExamples SENS:SEGM:FREQ:SPAN 1MHZ \nsense2:segment2:frequency:span max \nQuery Syntax SENSe<cnum>:SEGMent<snum>:FREQuency:SPAN? \nReturn Type Numeric \nDefault If first segment, frequency span of the analyzer. Otherwise 0. \nSENSe<cnum>:SEGMent<snum>:FREQuency:START <num> \n(Read-Write) Sets the Start Frequency for the specified sweep segment. \nNotes \nAll other segment Start and Stop Frequency values that are larger than this frequency are changed to \nthis frequency. \nTo return the start and stop frequency of the entire sweep (all segments), Use SENS:FREQ:STARt? \nand SENS:FREQ:STOP? \nParameters \n<cnum> Any existing channel number. If unspecified, value is set to 1 \n<snum> Segment number to modify. Choose any existing segment number. \n<num> Start Frequency in Hz. Choose any number between the minimum and \nmaximum frequency of the analyzer. \nNote: This command will accept MIN or MAX instead of a numeric parameter. \n1809\n\nSee SCPI Syntax for more information. \nExamples SENS:SEGM:FREQ:STAR 1MHZ \nsense2:segment2:frequency:start minimum \nQuery Syntax SENSe<cnum>:SEGMent<snum>:FREQuency:STARt? \nReturn Type Numeric \nDefault Stop Frequency of the previous segment. If first segment, start frequency of the \nanalyzer. \nSENSe<cnum>:SEGMent<snum>:FREQuency:STOP <num> \n(Read-Write) Sets the Stop Frequency for the specified sweep segment. \nNotes \nAll other segment Start and Stop Frequency values that are larger than this frequency are changed to \nthis frequency. \nTo return the start and stop frequency of the entire sweep (all segments), Use SENS:FREQ:STARt? \nand SENS:FREQ:STOP? \nParameters \n<cnum> Any existing channel number. If unspecified, value is set to 1 \n<snum> Segment number to modify. Choose any existing segment number. \n<num> Stop Frequency in Hz. Choose any number between the minimum and \nmaximum frequency of the analyzer. \nNote: This command will accept MIN or MAX instead of a numeric parameter. \nSee SCPI Syntax for more information. \nExamples SENS:SEGM:FREQ:STOP 1MHZ \nsense2:segment2:frequency:stop maximum \nQuery Syntax SENSe<cnum>:SEGMent<snum>:FREQuency:STOP? \nReturn Type Numeric \nDefault If first segment, stop frequency of the analyzer. Otherwise, start frequency of the \nsegment. \nSENSe<cnum>:SEGMent<snum>:POWer[<port>][:LEVel] <num> \n1810\n\n(Read-Write) Sets the Port Power level for the specified sweep segment. First set \nSENS:SEGM:POW:CONTrol ON. \nWhen port power is Coupled, setting port power for one port will apply port power for all source \nports. \nAll subsequent segments that are added assume the new Power Level value. \nParameters \n<cnum> Any existing channel number. If unspecified, value is set to 1 \n<snum> Segment number to modify. Choose any existing segment number. \n<port> Port number of the source. If unspecified, value is set to 1. \n<num> Power level. \nNote: The range of settable power values depends on the PNA model and if \nsource attenuators are installed. To determine the range of values, send \nSOUR:POW? MAX and SOUR:POW? MIN. (SOUR:POW:ATT:AUTO must \nbe set to ON). \nActual achievable leveled power depends on frequency. \nExamples SENS:SEGM:POW 0 \nsense2:segment2:power1:level -10 \nQuery Syntax SENSe<cnum>:SEGMent<snum>:POWer[<port>][:LEVel]? \nReturn Type Numeric \nDefault 0 \nSENSe<cnum>:SEGMent:POWer[:LEVel]:CONTrol <ON | OFF> \n1811\n\n(Read-Write) Specifies whether Power Level can be set independently for each segment. \nParameters \n<cnum> Any existing channel number. If unspecified, value is set to 1 \n<ON | OFF> ON (or 1) - turns Power Level control ON. Power level can be set for each \nsegment. \nOFF (or 0) - turns Power Level control OFF. Use the channel power level \nsetting. \nExamples SENS:SEGM:POW:CONT ON \nsense2:segment:power:level:control off \nQuery Syntax SENSe<cnum>:SEGMent:POWer[:LEVel]:CONTrol? \nReturn Type Boolean (1 = ON, 0 = OFF) \nDefault OFF \nSENSe<cnum>:SEGMent<snum>[:STATe] <ON | OFF> \n(Read-Write) Turns the specified sweep segment ON or OFF. At least ONE segment must be ON or \nSweep Mode is automatically set to Linear. \nParameters \n<cnum> Any existing channel number. If unspecified, value is set to 1 \n<snum> Segment number to be turned ON or OFF \n<ON | OFF> ON (or 1) - turns segment ON. \nOFF (or 0) - turns segment OFF. \nExamples SENS:SEGM ON \nsense2:segment2:state off \nQuery Syntax SENSe<cnum>:SEGMent<snum>[:STATe]? \nReturn Type Boolean (1 = ON, 0 = OFF) \nDefault OFF \nSENSe<cnum>:SEGMent<snum>:SWEep:POINts <num> \n1812\n\n(Read-Write) Sets the number of data points for the specified sweep segment. \nParameters \n<cnum> Any existing channel number. If unspecified, value is set to 1 \n<snum> Any existing segment number. If unspecified, value is set to 1 \n<num> Number of points in the segment. The total number of points in all segments \ncannot exceed 16001. A segment can have as few as 1 point. \nNote: This command will accept MIN or MAX instead of a numeric parameter. \nSee SCPI Syntax for more information. \nExamples SENS:SEGM:SWE:POIN 51 \nsense2:segment2:sweep:points maximum \nQuery Syntax SENSe<cnum>:SEGMent<snum>:SWEep:POINts? \nReturn Type Numeric \nDefault 21 \nSENSe<cnum>:SEGMent<snum>:SWEep:TIME <num> \n(Read-Write) Sets the time the analyzer takes to sweep the specified sweep segment. \nParameters \n<cnum> Any existing channel number. If unspecified, value is set to 1 \n<snum> Any existing segment number. \n<num> Sweep time in seconds. Choose a number between 0 and 100 \nNote: This command will accept MIN or MAX instead of a numeric \nparameter. See SCPI Syntax for more information. \nExamples SENS:SEGM:SWE:TIME 1ms \nsense2:segment2:sweep:time .001 \nQuery Syntax SENSe<cnum>:SEGMent<snum>:SWEep:TIME? \nReturn Type Numeric \nDefault Not Applicable \nSENSe<cnum>:SEGMent:SWEep:TIME:CONTrol <ON | OFF> \n1813\n\n(Read-Write) Specifies whether Sweep Time can be set independently for each sweep segment. \nParameters \n<cnum> Any existing channel number. If unspecified, value is set to 1 \n<ON | OFF> ON (or 1) - turns Sweep Time control ON. Sweep Time can be set for each \nsegment. \nOFF (or 0) - turns Sweep Time control OFF. Uses the channel Sweep Time \nsetting. \nExamples SENS:SEGM:SWE:TIM:CONT ON \nsense2:segment:sweep:time:control off \nQuery Syntax SENSe<cnum>:SEGMent:SWEep:TIME:CONTrol? \nReturn Type Boolean (1 = ON, 0 = OFF) \nDefault OFF \nSENSe<cnum>:SEGMent<snum>:X:SPACing <char> \n(Read-Write) Sets X-axis spacing ON or OFF \nParameters \n<cnum> Any existing channel number. If unspecified, value is set to 1 \n<snum> Any existing segment number. (This parameter is ignored) \n<char> LINear - turns X-axis point spacing OFF \nOBASe - turns X-axis point spacing ON \nExamples SENS:SEGM:X:SPACing LIN \nsense2:segment1:spacing obase \nQuery Syntax SENSe<cnum>:SEGMent<snum>:X:SPACing? \nReturn Type Character \nDefault LINear \n1814\n\nSense:Sweep Commands \nSpecifies the sweep functions of the analyzer. \nClick on a blue keyword to view the command details. \nSee Also \nExample Programs \nExample Triggering the PNA using SCPI \nLearn about Sweeping \nSynchronizing the PNA and Controller \nSCPI Command Tree \nNote: All of the commands in this block will accept MIN or MAX instead of a numeric parameter. \nAlso, kHZ, MHz, and GHz are accepted as suffixes/units. \nSee SCPI Syntax for more information. \nSENSe<cnum>:SWEep:DWELl <num> \n(Read-Write) Sets the dwell time between each sweep point. \nDwell time is ONLY available with SENSe:SWEep:GENeration set to STEPped; It is Not available in \nANALOG. \nSending dwell = 0 is the same as setting SENS:SWE:DWEL:AUTO ON. Sending a dwell time > 0 sets \nSENS:SWE:DWEL:AUTO OFF. \nParameters \n<cnum> Any existing channel number. If unspecified, value is set to 1 \n<num> Dwell time in seconds. \nSee Note \nExamples SENS:SWE:DWEL .1 \nsense2:sweep:dwell min \n1815\n\nQuery Syntax SENSe<cnum>:SWEep:DWELl? \nReturn Type Numeric \nDefault 0 - (Note: dwell time set to 0 is the same as dwell:auto ON) \nSENSe<cnum>:SWEep:DWELl:AUTO <ON | OFF> \n(Read-Write) Specifies whether or not to automatically calculate and set the minimum possible dwell time. Setting \nAuto ON has the same effect as setting dwell time to 0. \nParameters \n<cnum> Any existing channel number. If unspecified, value is set to 1 \n<ON | OFF> ON (or 1) - turns dwell ON. \nOFF (or 0) - turns dwell OFF. \nExamples SENS:SWE:DWEL:AUTO ON \nsense2:sweep:dwell:auto off \nQuery Syntax SENSe<cnum>:SWEep:DWELl:AUTO? \nReturn Type Boolean (1 = ON, 0 = OFF) \nDefault ON \nSENSe<cnum>:SWEep:GENeration <char> \n(Read-Write) Sets sweep as Stepped or Analog. \nParameters \n<cnum> Any existing channel number. If unspecified, value is set to 1 \n<char> Choose from: \nSTEPped - source frequency is CONSTANT during measurement of eah displayed \npoint. More accurate than ANALog. Dwell time can be set in this mode. \nANALog - source frequency is continuously RAMPING during measurement of each \ndisplayed point. Faster than STEPped. Sweep time (not dwell time) can be set in this \nmode. \nExamples SENS:SWE:GEN STEP \nsense2:sweep:generation analog \nQuery Syntax SENSe<cnum>:SWEep:GENeration? \nReturn Type Character \nSENSe<cnum>:SWEep:GROups:COUNt <num>\n1816\n\nDefault Analog \nSENSe<cnum>:SWEep:GROups:COUNt <num> \n(Read-Write) Sets the trigger count (groups) for the specified channel. Set trigger mode to group after setting this \ncount. \nParameters \n<cnum> Any existing channel number. If unspecified, value is set to 1 \n<num> Count (groups) number. Choose any number between: \n1 and 2e6 (1 is the same as single trigger) \nExamples SENS:SWE:GRO:COUN 10 \nsense2:sweep:groups:count 50 \nQuery Syntax SENSe<cnum>:SWEep:GROups:COUNt? \nReturn Type Numeric \nDefault 1 \nSENSe<cnum>:SWEep:MODE <char> \n(Read-Write) Sets the number of trigger signals the specified channel will ACCEPT. \nSee Triggering the PNA Using SCPI. \nParameters \n<cnum> Any existing channel number. If unspecified, value is set to 1 \n<char> Trigger mode. Choose from: \nHOLD - channel will not trigger \nCONTinuous - channel triggers indefinitely \nGROups - channel accepts the number of triggers specified with the last \nSENS:SWE:GRO:COUN <num>. This is one of the PNA overlapped commands. Learn \nmore. \nHow to specify Single Trigger - Internal or External: \n1. Send SENS:SWE:GRO:COUN 1 \n2. Send SENS:SWE:MODE GROups. When received, the specified PNA channel \nIMMEDIATELY accepts one trigger signal, if available, then goes into hold. To accept \nanother trigger signal, resend SENS:SWE:MODE GROups. \n1817\n\nExamples SENS:SWE:MODE CONT \nsense2:sweep:mode hold \nQuery Syntax SENSe<cnum>:SWEep:MODE? \nReturn Type Character \nDefault CONTinuous \nSENSe<cnum>:SWEep:POINts <num> \n(Read-Write) Sets the number of data points for the measurement. \nParameters \n<cnum> Any existing channel number. If unspecified, value is set to 1 \n<num> Choose any number between 1 and 16001 \nNote: This command will accept MIN or MAX instead of a numeric parameter. See SCPI \nSyntax for more information. \nExamples SENS:SWE:POIN 51 \nsense2:sweep:points max \nQuery Syntax SENSe<cnum>:SWEep:POINts? \nReturn Type Numeric \nDefault 201 \nSENSe<cnum>:SWEep:SRCPort <1 | 2> Superseded \nThis command is superseded. The Calc:Par:Def:Ext and Calc:Par:Mod:Ext can now optionally include the source \nport. \n(Read-Write) Sets the source port when making non S-parameter measurements. Has no effect on S-parameter \nmeasurements. \nParameters \n<cnum> Any existing channel number. If unspecified, value is set to 1 \n<1 | 2> 1 - Source power comes out Port 1 \n2 - Source power comes out Port 2 \nExamples SENS:SWE:SRCP 1 \nsense2:sweep:srcport 2 \nQuery Syntax SENSe<cnum>:SWEep:SRCPort? \n1818\n\nReturn Type Character \nDefault 1 \nSENSe<cnum>:SWEep:TIME <num> \n(Read-Write) Sets the time the analyzer takes to complete one sweep. If sweep time accuracy is critical, use \nONLY the values that are attained using the up and down arrows next to the sweep time entry box. See Sweep \nTime. \nParameters \n<cnum> Any existing channel number. If unspecified, value is set to 1 \n<num> Sweep time in seconds. Choose a number between 0 and 86,400 (24hrs), \nTo select the fastest sweep speed, either send MIN as an argument to this command, or \nsend SENS:SWE:TIME:AUTO 1 \nSee Note \nExamples SENS:SWE:TIME 1ms \nsense2:sweep:time .001 \nQuery Syntax SENSe<cnum>:SWEep:TIME? \nReturn Type Numeric \nDefault NA \nSENSe<cnum>:SWEep:TIME:AUTO <ON | OFF> \n(Read-Write) Turns the automatic sweep time function ON or OFF. \nParameters \n<cnum> Any existing channel number. If unspecified, value is set to 1 \n<ON | OFF> ON (or 1) - turns the automatic sweep time ON. \nOFF (or 0) - turns the automatic sweep time OFF. \nExamples SENS:SWE:TIME:AUTO \nsense2:sweep:time:auto off \nQuery Syntax SENSe<cnum>:SWEep:TIME:AUTO? \nReturn Type Boolean (1 = ON, 0 = OFF) \nDefault ON \n1819\n\nSENSe<cnum>:SWEep:TRIGger:DELay <num> \n(Read-Write) Sets and reads the trigger delay for all measurements in the specified CHANNEL. This delay is only \napplied while TRIG:SOURce EXTernal and TRIG:SCOP CURRent . After an external trigger is applied, the start \nof the sweep is delayed for the specified delay value plus any inherent latency. \nTo apply a trigger delay for all channels (Global), use TRIG:DEL \nParameters \n<cnum> Any existing channel number. If unspecified, value is set to 1 \n<num> Trigger delay value in seconds. Range is from 0 to 107 seconds \nExamples SENS:SWE:TRIG:DELay .003 \nsense2:sweep:trigger:delay 1 \nQuery Syntax SENSe<cnum>:SWEep:TRIGger:DELay? \nReturn Type Numeric \nDefault 0 \nSENSe<cnum>:SWEep:TRIGger:POINt <ON | OFF> \n(Read-Write) Specifies whether the specified channel will measure one point for each trigger or all of the \nmeasurements in the channel. Setting any channel to POINt mode will automatically set the TRIGger:SCOPe = \nCURRent.\nParameters \n<cnum> Any existing channel number. If unspecified, value is set to 1 \n<ON | OFF> ON (or 1) - Channel measures one data point per trigger. \nOFF (or 0) - All measurements in the channel made per trigger. \nExamples SENS:SWE:TRIG:POIN ON \nsense2:sweep:trigger:point off \nQuery Syntax SENSe<cnum>:SWEep:TRIGger:POINt? \nReturn Type Boolean (1 = Point, 0 = Measurement) \nDefault 0 - Measurement \nSENSe<cnum>:SWEep:TYPE <char> \n1820\n\n(Read-Write) Sets the type of analyzer sweep mode. \nParameters \n<cnum> Any existing channel number. If unspecified, value is set to 1 \n<char> Choose from: \nLINear | LOGarithmic | POWer | CW | SEGMent \nNote: SWEep TYPE cannot be set to SEGMent if there are no segments turned ON. A \nsegment is automatically turned ON when the analyzer is started. \nExamples SENS:SWE:TYPE LIN \nsense2:sweep:type segment \nQuery Syntax SENSe<cnum>:SWEep:TYPE? \nReturn Type Character \nDefault LINear \nLast Modified: \n24-Apr-2007 Clarified Sweep mode \n1821\n\nX Values Command \nSENSe<cnum>:X[:VALues]? \n(Read-only) Returns the stimulus values for the specified channel. If the channel is sweeping the \nsource backwards, the values will be in descending order. \nParameters \n<cnum> Any existing channel number; if unspecified, value is set to 1. \nExamples SENS:X? \nsense2:x:values? \nReturn Type Depends on FORM:DATA command \nDefault Not applicable \n1822\n\nSource Commands \nControls the power delivered to the DUT. \nClick on a blue keyword to view the command details. \nSee Also \nExample Programs \nLearn about Power Settings \nSynchronizing the PNA and Controller \nSCPI Command Tree \nSOURce<cnum>:CATalog? \n1823\n\n(Read-Write) Returns a list of valid port names that can be controlled. Some of these port names can \nNOT be accessed through the normal <port> argument used in many Source: commands. These string \nnames are used in the [src] argument. \nParameters \nExamples SOUR:CAT? \nsource:catalog \n'returns \n\"Port 1,Port 2,Port 3,Port 4,Port 1 Src2\" \nReturn Type Comma-separated list of strings. \nDefault Not applicable \nSOURce<cnum>:POWer<port>:ALC[:MODE]:CATalog?, [src] \n(Read-Write) Returns a list of valid ALC modes for the specified channel and port number. Use the \nreturned values to set SOUR:POW:ALC:MODE. \nParameters \n<cnum> Any existing channel number. If unspecified, value is set to 1 \n<port> Port number of the PNA. If unspecified, value is set to 1. To make settings for \nports that are not simple numbers, use the [src] argument. \n[src] String. (NOT case sensitive). Source port. Optional. Use SOUR:CAT? to \nreturn a list of valid port names. \nWhile this argument can be used to make settings for ALL ports, it is designed \nto access ports that are not simple numbers, such as \"Port 1 Src2\". Otherwise, \nthe <port> argument performs the same function. If both arguments are \nspecified, [src] takes priority. \nExamples SOUR:POW:ALC:MODE:CAT? \nsource2:power2:alc:mode:catalog? \nsource:power:alc:mode:catalog? \"Port 1 Src2\" \nReturn Type Comma-separated list of strings. \nDefault Not applicable \nSOURce<cnum>:POWer<port>:ALC[:MODE] <char>, [src] \n1824\n\n(Read-Write) Sets and returns the ALC mode for the specified channel and port. Use \nSOUR:POW:ALC:MODE:CAT? to return a list of valid ALC modes for the PNA. \nLearn more about ALC mode. \nParameters \n<cnum> Any existing channel number. If unspecified, value is set to 1 \n<port> Port number of the PNA. If unspecified, value is set to 1. To make settings for \nports that are not simple numbers, use the [src] argument. \n<char> ALC Mode. \nFor the PNA-X choose from: \nINTernal Standard ALC loop \nOPENloop No ALC loop \n[src] String. (NOT case sensitive). Source port. Optional. Use SOUR:CAT? to \nreturn a list of valid port names. \nWhile this argument can be used to make settings for ALL ports, it is designed \nto access ports that are not simple numbers, such as \"Port 1 Src2\". Otherwise, \nthe <port> argument performs the same function. If both arguments are \nspecified, [src] takes priority. \nExamples SOUR:POW:ALC INT \nsource2:power2:alc:mode openloop \nsource:power:alc:mode openloop,\"Port 1 Src2\" \nQuery Syntax SOURce<cnum>:POWer<port>:ALC:MODE? [src] \nReturn Type Character \nDefault INTernal \nSOURce<cnum>:POWer<port>:ATTenuation <num>, [src] \n1825\n\n(Read-Write) Sets the attenuation level for the selected channel. Sending this command turns \nautomatic attenuation control (SOUR:POW:ATT:AUTO) to OFF. If the ports are coupled, changing \nthe attenuation on one port will also change the attenuation on all other ports. To turn port coupling \nOFF use SOURce:POWer:COUPle OFF. \nNote: Attenuation cannot be set with Sweep Type set to Power \nParameters \n<cnum> Any existing channel number. If unspecified, value is set to 1 \n<port> Port number of the PNA. If unspecified, value is set to 1. To make settings for \nports that are not simple numbers, use the [src] argument. \n<num> Attenuation value. The range of settable values depends on the PNA model. \nTo determine the range of values, perform a query using MAX, then MIN, as \nan argument. Example: SOURce:POWer:ATT? Max \nEnter a value between MAX and MIN in 10 dB steps. \nIf a number other than these is entered, the analyzer will select the next lower \nvalid value. For example, if 19.9 is entered for <num> the analyzer will switch \nin 10 dB attenuation. \nNote: This command will accept MIN or MAX instead of a numeric \nparameter. See SCPI Syntax for more information. \n[src] String. (NOT case sensitive). Source port. Optional. Use SOUR:CAT? to \nreturn a list of valid port names. \nWhile this argument can be used to make settings for ALL ports, it is designed \nto access ports that are not simple numbers, such as \"Port 1 Src2\". Otherwise, \nthe <port> argument performs the same function. If both arguments are \nspecified, [src] takes priority. \nExamples SOUR:POW:ATT 10 \nsource2:power2:attentuation maximum \nsource:power:att 2, \"Port 1 Src2\" \nQuery Syntax SOURce<cnum>:POWer<port>:ATTenuation? [src] \nReturn Type Numeric \nDefault 0 \nSOURce<cnum>:POWer<port>:ATTenuation:AUTO <bool>, [src] \n1826\n\n(Read-Write) Turns automatic attenuation control ON or OFF. Setting an attenuation value (using"
uses:
  PNA-X.lvlib
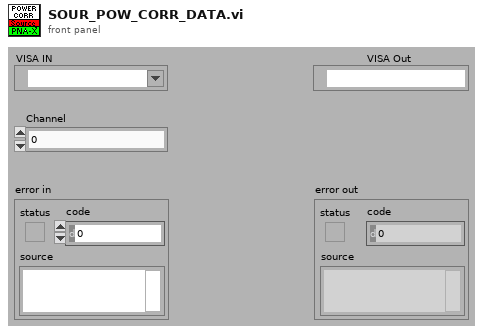
[diagram p1: front panel]
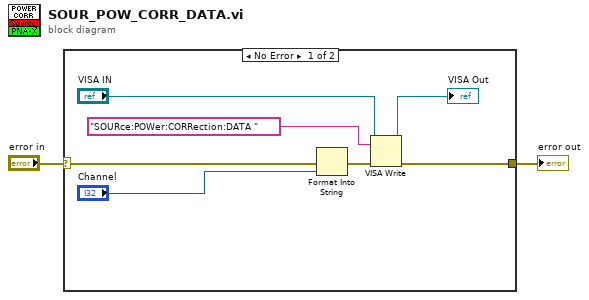
[diagram p0: block diagram]
diagram:
  n1 = case shown="No Error" "error in" {
    selector: "error in" -> [w9 w10]
    tunnel: [w6 w10] -> w1
    frame No Error {
      n2 = Format Into String(error in=w9, "Channel") -> (error out=w8:errorcluster)  [unwired: 2 in, 1 out]
      n3 = VISA Write(VISA resource name="VISA IN", write buffer="SOURce:POWer:CORRection:DATA " ("Cmdline"), error in (no error)=w8) -> (VISA resource name out=→"VISA Out":refnum<visa-resource-name>, error out=w6:errorcluster)  [unwired: 1 out]
    }
    frame Error {
    }
  }
  "error out" <- w1
